vi "ScriptedStateMachine.vi"(8 "ErrorArray In":errorcluster[](array[cluster]), 9 "Data in":variant, 10 "Script":string[](array[string])=["Test,1,2,3", "stop"], 11 "Bus":refnum<class "Bus.lvclass">) -> (0 "ErrorArray Out":errorcluster[](array[cluster]), 2 "Data out":variant, 3 "Bus":refnum<class "Bus.lvclass">)   [LabVIEW 2014, in "Bus_class.lvlib" / "Bus.lvclass"]
uses:
  Bus.lvclass
  Public/TypeDefs/clBusData.ctl
  FrontPanel/TypeDefs/clEventConfig.ctl
  Modules/PmuImpairPlugins/PmuImpairPluginBase_class/TypeDefs/clImpairConfig.ctl
  Modules/EventPlugins/EventPluginBaseClass/TypeDefs/clEvtReportArray.ctl
  Modules/EventPlugins/EventPluginBaseClass/TypeDefs/clEvtReport.ctl
  Modules/EventPlugins/EventPluginBaseClass/TypeDefs/dblEvtSignalArray.ctl
  Modules/NetworkImpairmentModule/PublicAPI/Arguments/Broadcasts/dblNetworkTime.ctl
  Modules/NetworkImpairmentModule/PublicAPI/Arguments/Broadcasts/dblPktLoss.ctl
  Modules/FlagImpairModule/PublicAPI/Arguments/Broadcasts/ui32FlagImpairmentArray.ctl
  Modules/OutputToFilePlugins/OutputToFileBasePlugin/Typedefs/PmuCfgOpt.ctl
  Bus.lvclass/Bus.ctl
  BdcstInfo.ctl
  ModuleType.ctl
  FrontPanel/TypeDefs/clFrontPanelControlRefs.ctl
  Modules/PmuImpairModule/PublicAPI/Arguments/Broadcasts/clErrorRpt.ctl
  Modules/EventPlugins/EventPluginBaseClass/TypeDefs/clEvtConfig.ctl
  Accessors/Read AppModuleID.vi
  Accessors/Read OutputToFileModuleID.vi
  <vilib>/Utility/error.llb/Error Cluster From Error Code.vi
  <vilib>/Analysis/1siggen.llb/Ramp Pattern by Delta.vi
  <vilib>/ErrorRing/Error Ring.xnode
  <userlib>/NIST/NISTErrorLib/NISTErrorLib.lvlib
  Framework.lvlib
  Modules/EventModule/EventModule.lvlib
  Modules/EventPlugins/EventPluginBaseClass/EventPluginBaseClass.lvclass
  <vilib>/Analysis/NI_AALBase.lvlib
  Modules/PmuImpairModule/PmuImpairModule.lvlib
  Modules/NetworkImpairmentModule/NetworkImpairmentModule.lvlib
  Modules/FlagImpairModule/FlagImpairModule.lvlib
  Modules/PmuImpairPlugins/PmuImpairPluginBase_class/PmuImpairPluginBase.lvclass
  Modules/OutputToFilePlugins/OutputToFileBasePlugin/OutputToFileBasePlugin.lvclass
  Modules/OutputToFileModule/OutputToFileModule.lvlib
  Modules/AppModule/AppModule.lvlib
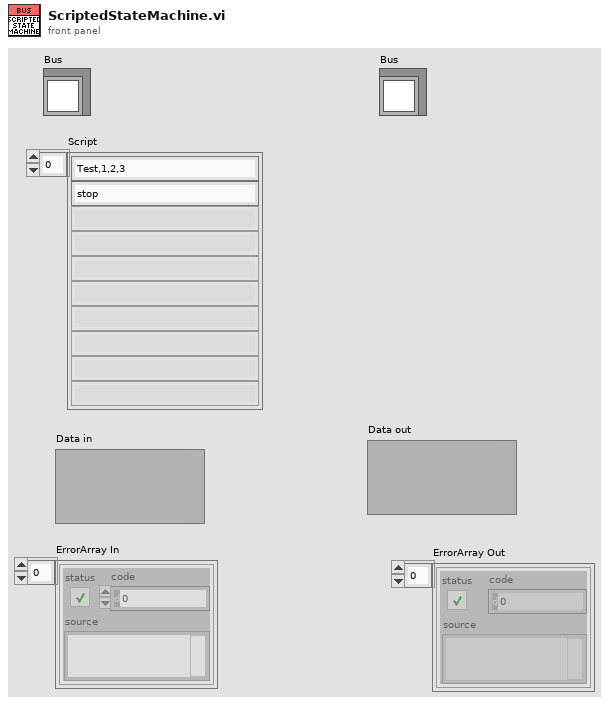
[diagram p1: front panel]
types:
  T1 = typedef "Bus_class.lvlib/Bus.lvclass/clBusData.ctl" = cluster{"BusNumber":u8, "EvtPluginINIFilePath":path, "EvtParams":string[][], "EvtConfig":T2, "Start Time":dbl, "End Time":dbl, "PmuImpairPluginINIFilePath":path, "PmuImpairParams ":string[][], "PmuImpairConfig":T3, "NetImpPluginINIFilePath":path, "NetImpParams":string[][], "FlagImpPluginINIFilePath":path, "FlagImpParams":string[][], "EvtReportArray":T4, "EventSignalArray":T6, "ImpairReportArray":T4, "NetworkTime":T7, "PktLoss":T8, "FlagImpArray":T9, "OutputToFilePluginINIFilePath":path, "Output File Path":path, "clConfigOptions":T10, "AppPluginINIFilePath":path, "AppConfig":variant, "AppOutput":variant}
  T2 = typedef "Framework.lvlib/clEventConfig.ctl" = cluster{"UTC Time 0":timestamp, "Nominal Frequency":u16, "Reporting Rate":u16, "Fsamp":u32, "PosSeq":bool}
  T3 = typedef "PmuImpairPlugins.lvlib/PmuImpairPluginBase.lvclass/clImpairConfig.ctl" = cluster{"FilterType":string, "bPosSeq":bool}
  T4 = typedef "EventPlugins.lvlib/EventPluginBaseClass.lvclass/clEvtReportArray.ctl" = T5[]
  T5 = typedef "EventPlugins.lvlib/EventPluginBaseClass.lvclass/clEvtReport.ctl" = cluster{"Timestamp":dbl, "Synx":cdb[], "Freq":dbl, "ROCOF":dbl, "ID":i16}
  T6 = typedef "EventPlugins.lvlib/EventPluginBaseClass.lvclass/dblEvtSignalArray.ctl" = dbl[][]
  T7 = typedef "NetworkImpairmentModule.lvlib/dblNetworkTime.ctl" = dbl[]
  T8 = typedef "NetworkImpairmentModule.lvlib/dblPktLoss.ctl" = dbl[]
  T9 = typedef "FlagImpairModule.lvlib/ui32FlagImpairmentArray.ctl" = u32[]
  T10 = typedef "OutputToFilePlugins.lvlib/OutputToFileBasePlugin.lvclass/PmuCfgOpt.ctl" = cluster{"TIME_BASE":u64, "STN":string, "IDCODE":u16, "rdoPolRect":enum32{"Rectangular", "Polar"}, "rdoFloatInt":enum32{"Float", "Integer"}, "PHUNIT":u64, "rdoFreqDfreq":enum32{"Float", "Integer"}, "CHNAM":string[], "chkCfg2Prefix":bool}
  T11 = typedef "Bus_class.lvlib/Bus.lvclass/ModuleType.ctl" = enum16{"PMU", "Event", "Network", "Flag", "App", "OutToFile"}
  T12 = typedef "Bus_class.lvlib/Bus.lvclass/BdcstInfo.ctl" = cluster{"ModuleType":T11, "ModuleID":i32, "UsrEvtRef":variant, "ScriptCmd":string}
  T13 = typedef "Framework.lvlib/clFrontPanelControlRefs.ctl" = cluster{"TestFilePathRef":refnum<vi>, "BusNumberRef":refnum<vi>, "NumberOfBusesRef":refnum<vi>, "EvtTypeRef":refnum<vi>, "EvtParamsRef":refnum<vi>, "EvtConfigRef":refnum<vi>, "StartTimeRef":refnum<vi>, "EndTimeRef":refnum<vi>, "PmuImpairTypeRef":refnum<vi>, "PmuImpairParamsRef":refnum<vi>, "NetImpairParamsRef":refnum<vi>, "FlagImpairTypeRef":refnum<vi>, "FlagImpairParamsRef":refnum<vi>, "NetImpairTypeRef":refnum<vi>, "OutputFileType":refnum<vi>, "PmuImpairConfigRef":refnum<vi>, "AppTypeRef":refnum<vi>, "ScriptPathRef":refnum<vi>, "ShowPanels?":refnum<vi>}
  T14 = typedef "PmuImpairModule.lvlib/clErrorRpt.ctl" = cluster{"error":errorcluster, "AdditionalInfo":string}
  T15 = typedef "EventPlugins.lvlib/EventPluginBaseClass.lvclass/clEvtConfig.ctl" = cluster{"T0(UTC)":dbl, "F0":dbl, "Fs":i32, "FSamp":u32, "bPosSeq":bool}
  T16 = typedef "EventModule.lvlib/clBroadcastEvents.ctl" = cluster{"DidInit":refnum<user-event>, "StatusUpdate":refnum<user-event>, "ErrorReport":refnum<user-event>, "DidStop":refnum<user-event>, "ReadEvtConfig":refnum<user-event>, "ReadTimeArray":refnum<user-event>, "ReadEvtParams":refnum<user-event>, "GetEvtReportArray":refnum<user-event>, "ReadPathToPlugin":refnum<user-event>, "GetEvtSignal":refnum<user-event>, "ReadBusNumber":refnum<user-event>}
  T17 = typedef "PmuImpairModule.lvlib/clBroadcastEvents.ctl" = cluster{"DidInit":refnum<user-event>, "StatusUpdate":refnum<user-event>, "ErrorReport":refnum<user-event>, "DidStop":refnum<user-event>, "ImpairConfig":refnum<user-event>, "ImpairParams":refnum<user-event>, "ImpairReports":refnum<user-event>, "PathToPlugin":refnum<user-event>, "BusNumber":refnum<user-event>}
  T18 = typedef "NetworkImpairmentModule.lvlib/clBroadcastEvents.ctl" = cluster{"DidInit":refnum<user-event>, "StatusUpdate":refnum<user-event>, "ErrorReport":refnum<user-event>, "DidStop":refnum<user-event>, "ReadNetImpParams":refnum<user-event>, "ReadLossThreshold":refnum<user-event>, "GetNetworkTime":refnum<user-event>, "GetPktLoss":refnum<user-event>, "ReadPathToPlugin":refnum<user-event>}
  T19 = typedef "FlagImpairModule.lvlib/clBroadcastEvents.ctl" = cluster{"DidInit":refnum<user-event>, "StatusUpdate":refnum<user-event>, "ErrorReport":refnum<user-event>, "DidStop":refnum<user-event>, "ReadFlagImpairConfig":refnum<user-event>, "ReadPluginINIFilePath":refnum<user-event>, "ReadFlagImpairParams":refnum<user-event>, "ReadTimeArray":refnum<user-event>, "GetFlagImpairment":refnum<user-event>}
  T20 = typedef "OutputToFileModule.lvlib/clBroadcastEvents.ctl" = cluster{"DidInit":refnum<user-event>, "StatusUpdate":refnum<user-event>, "ErrorReport":refnum<user-event>, "DidStop":refnum<user-event>, "PathToPlugin":refnum<user-event>, "PmuConfig":refnum<user-event>, "OutputPath":refnum<user-event>}
  T21 = typedef "AppModule.lvlib/clBroadcastEvents.ctl" = cluster{"DidInit":refnum<user-event>, "StatusUpdate":refnum<user-event>, "ErrorReport":refnum<user-event>, "DidStop":refnum<user-event>, "PathToINI":refnum<user-event>, "InputData":refnum<user-event>, "OutputData":refnum<user-event>, "BcAppInfo":refnum<user-event>, "ConfigData":refnum<user-event>}
  T22 = typedef "Framework.lvlib/clFrameworkData.ctl" = cluster{"EvtINIFilePaths":path[], "BusClassInstances":refnum<class "Bus.lvclass">[], "PmuImpairINIFilePaths":path[], "FlagImpairINIFilePaths":path[], "NetImpairINIFilePaths":path[], "OutputToFileINIFilePaths":path[], "AppINIFilePaths":path[], "AppModuleID":i32, "OutputToFileID":i32}
  T23 = typedef "Framework.lvlib/QueRef.ctl" = refnum<queue>
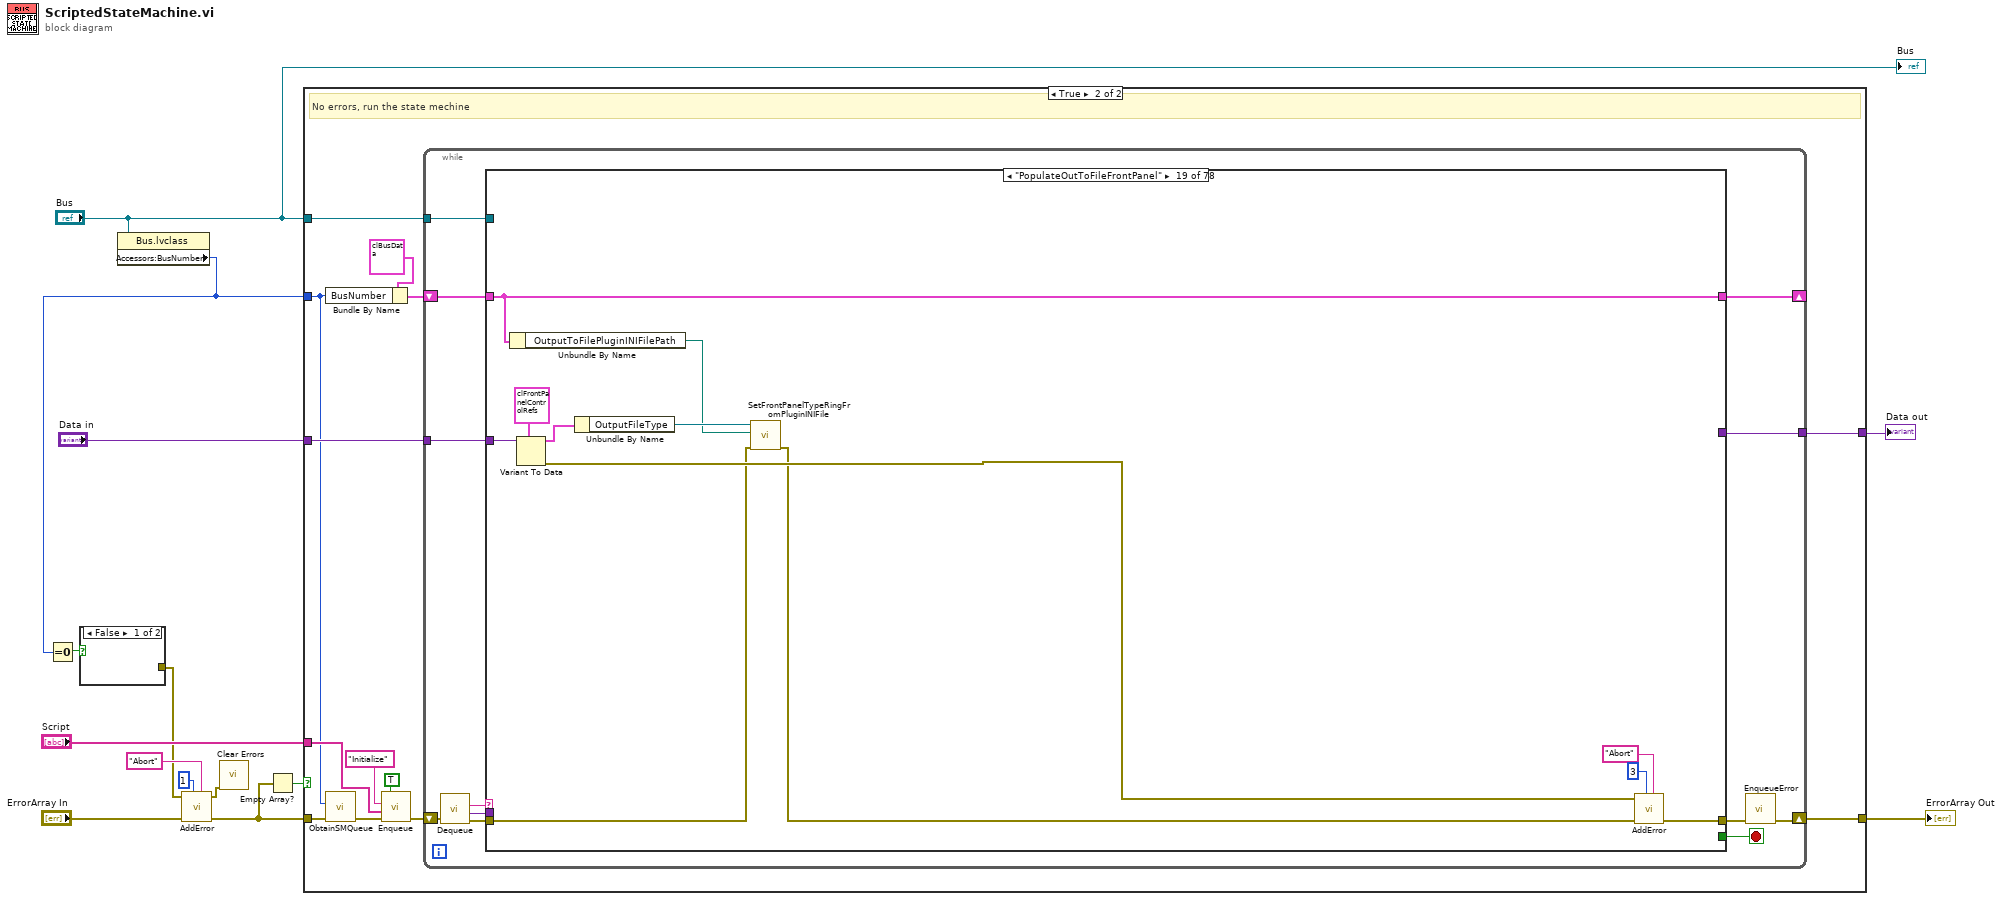
[diagram p0: block diagram]
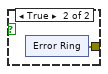
[diagram p2: hidden frame]
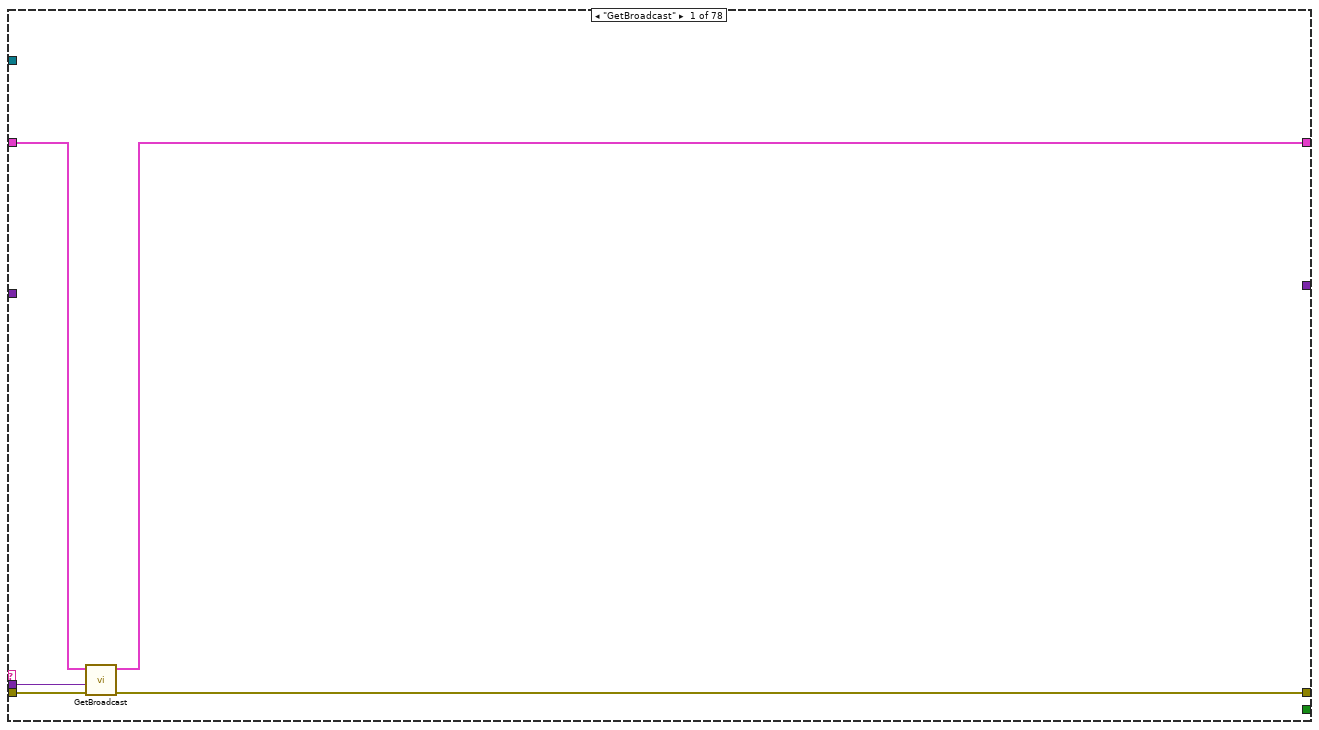
[diagram p4: hidden frame]
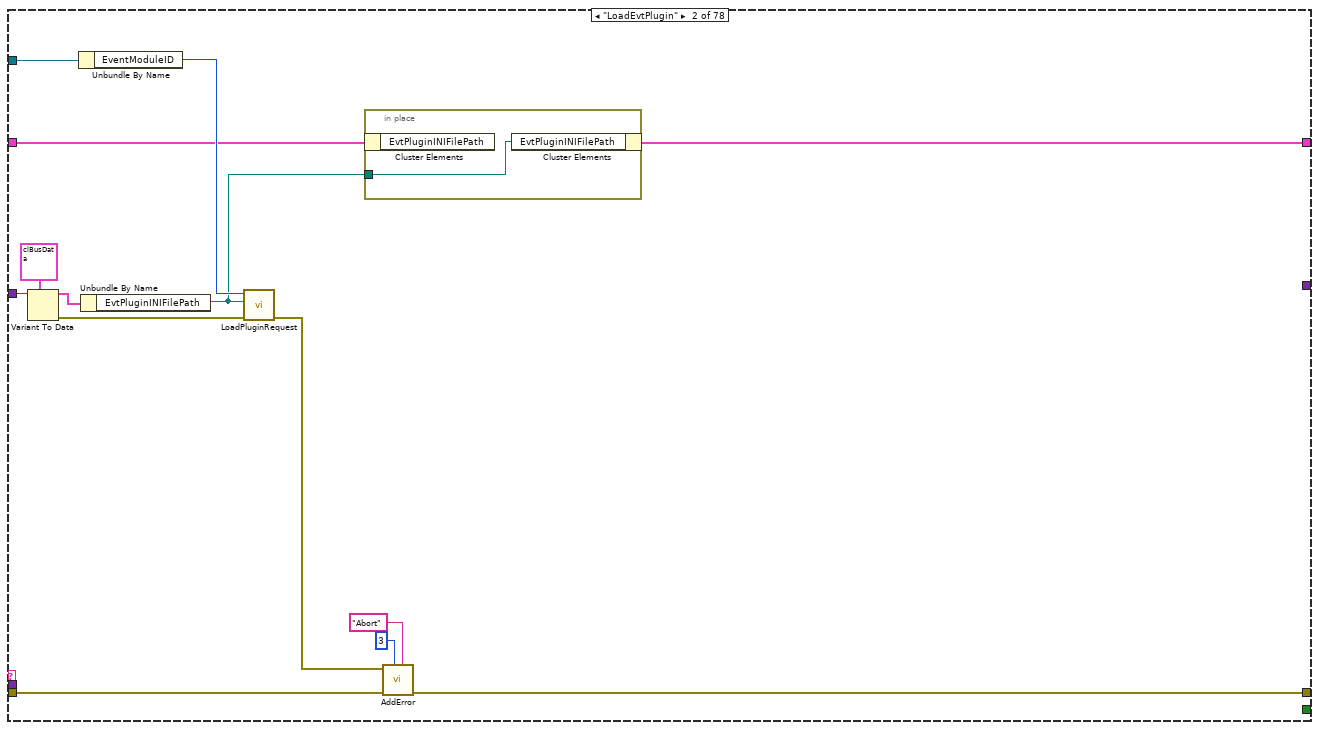
[diagram p5: hidden frame]
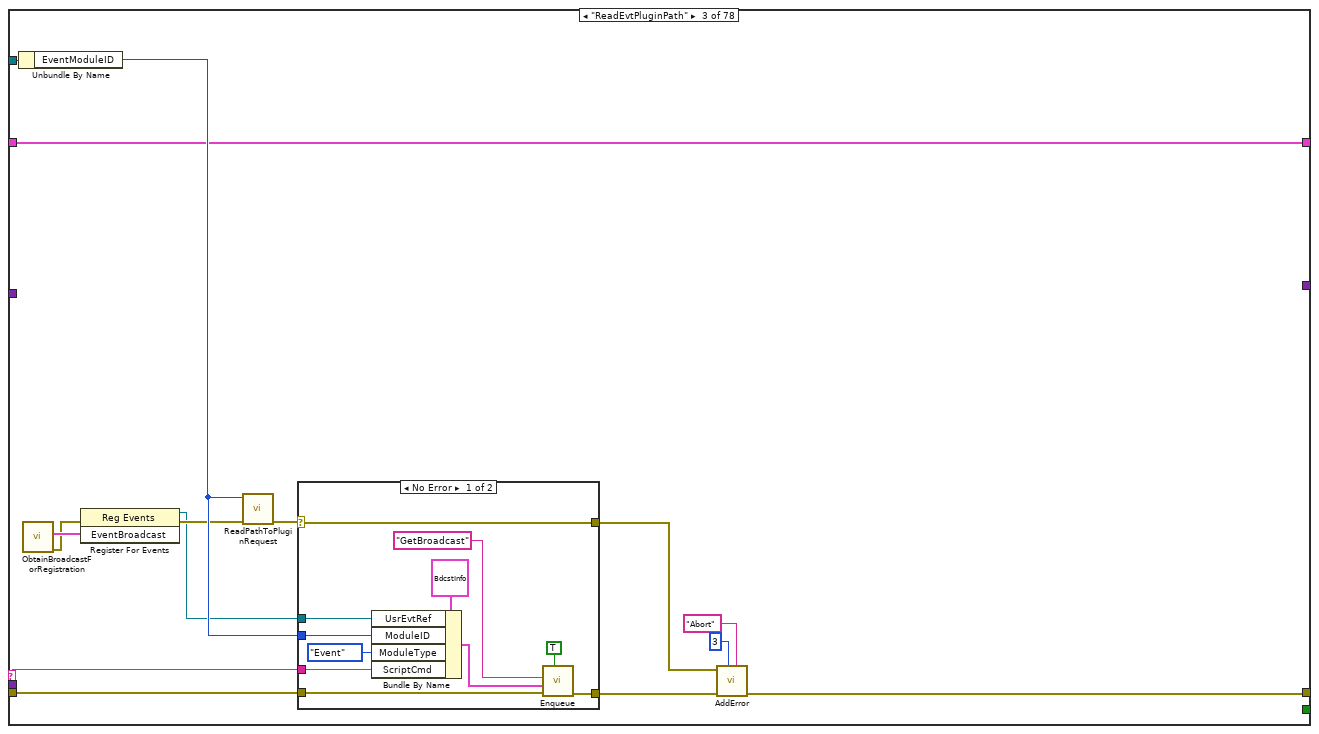
[diagram p6: hidden frame]
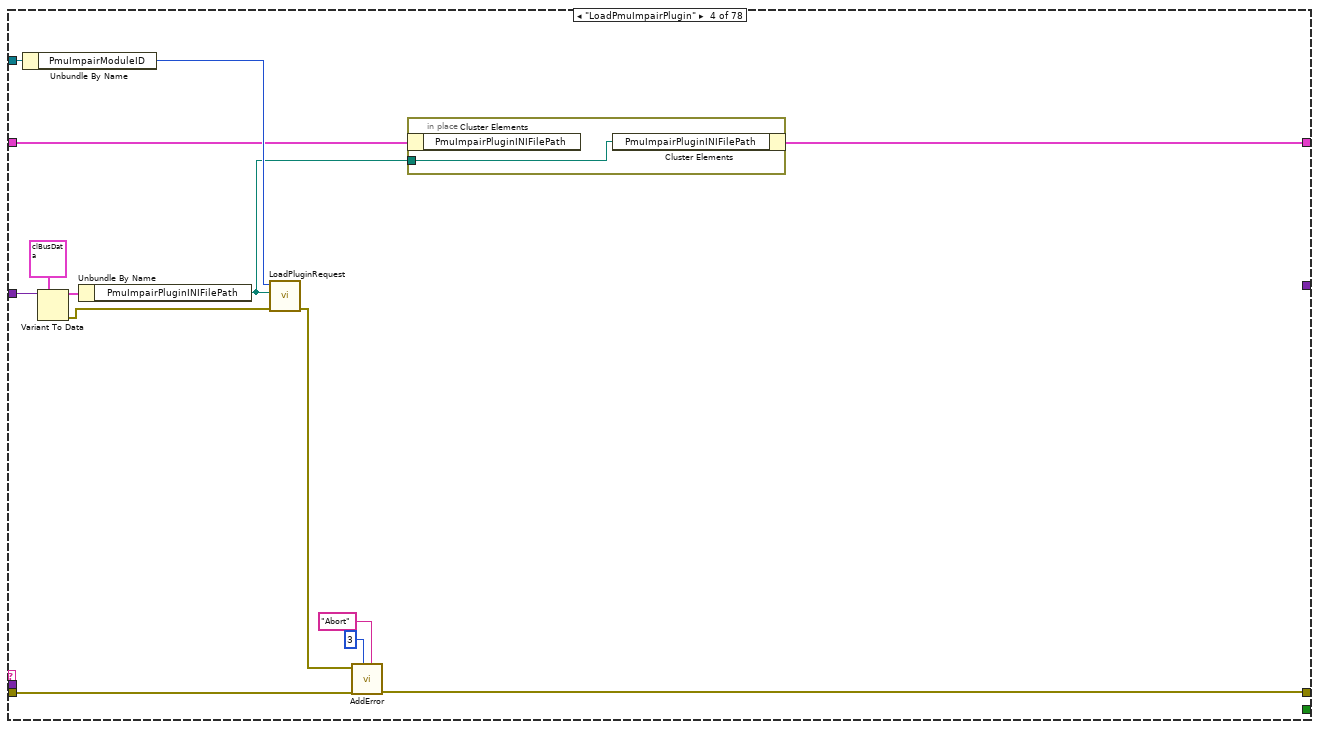
[diagram p8: hidden frame]
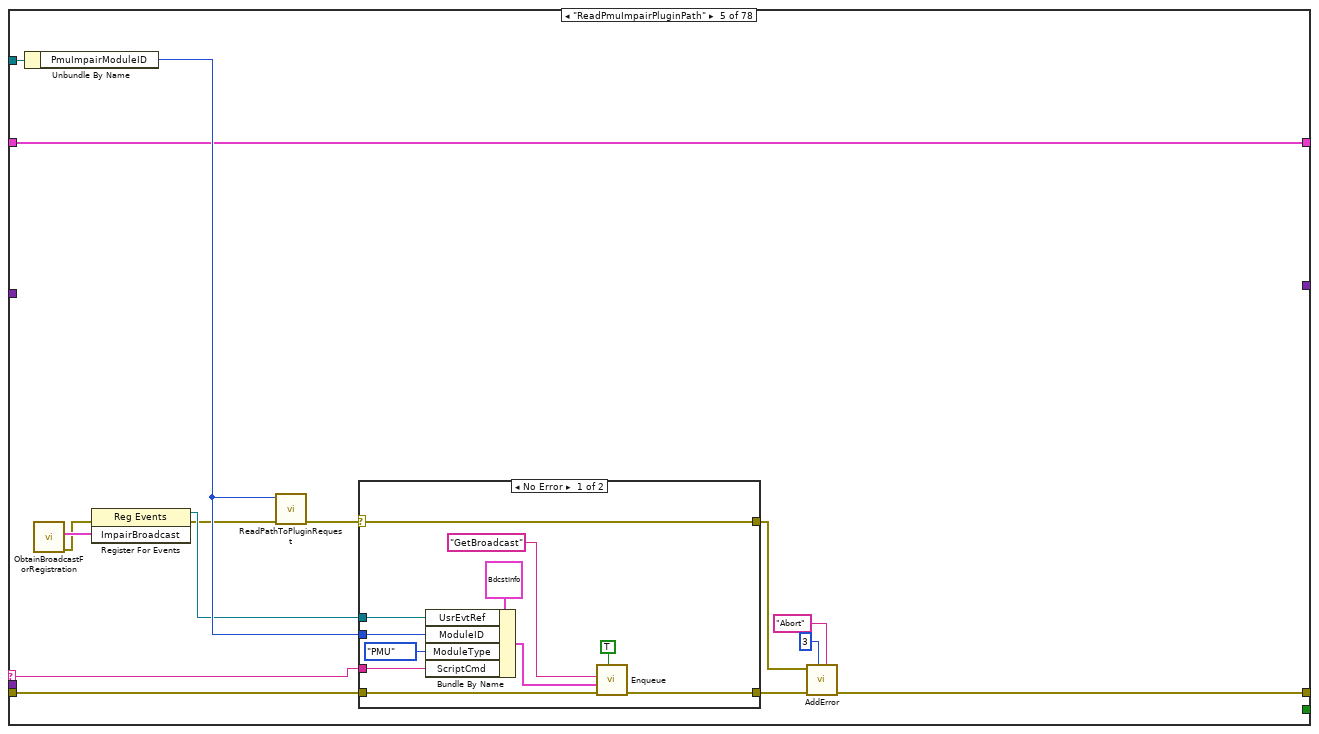
[diagram p9: hidden frame]
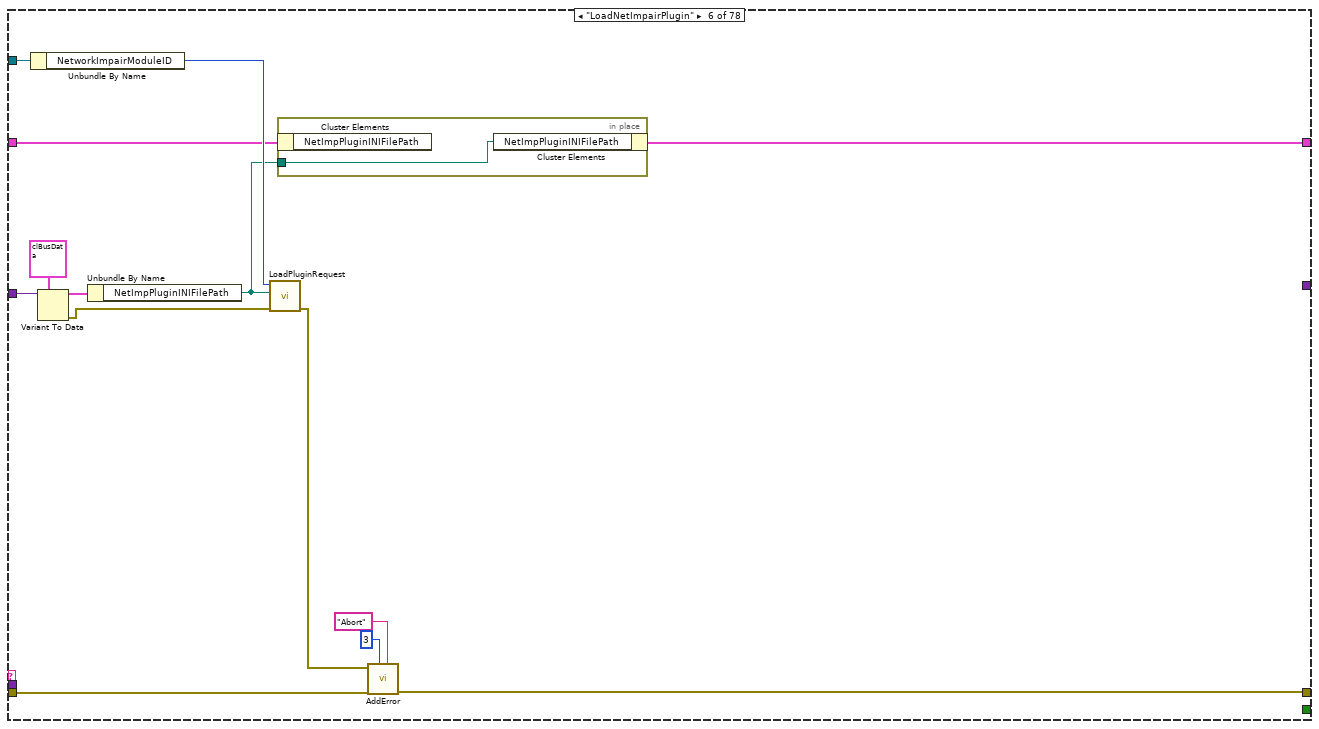
[diagram p11: hidden frame]
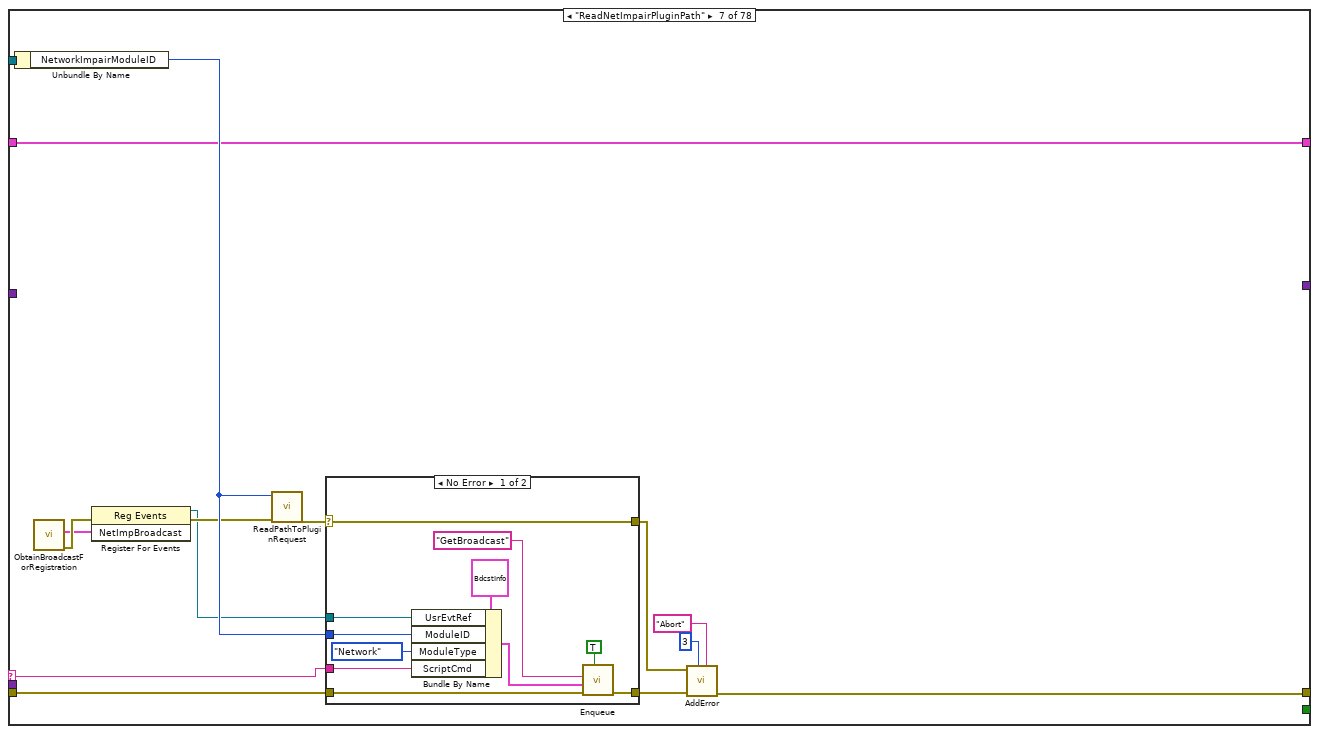
[diagram p12: hidden frame]
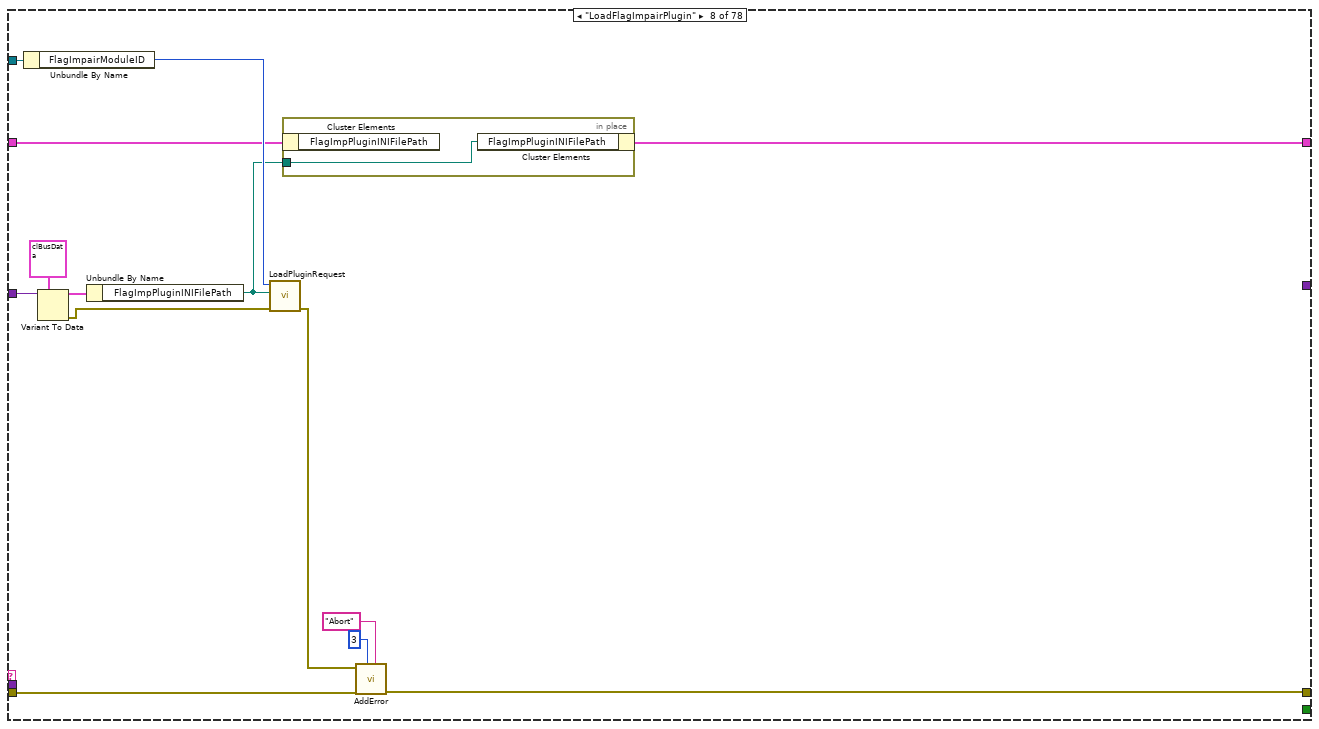
[diagram p14: hidden frame]
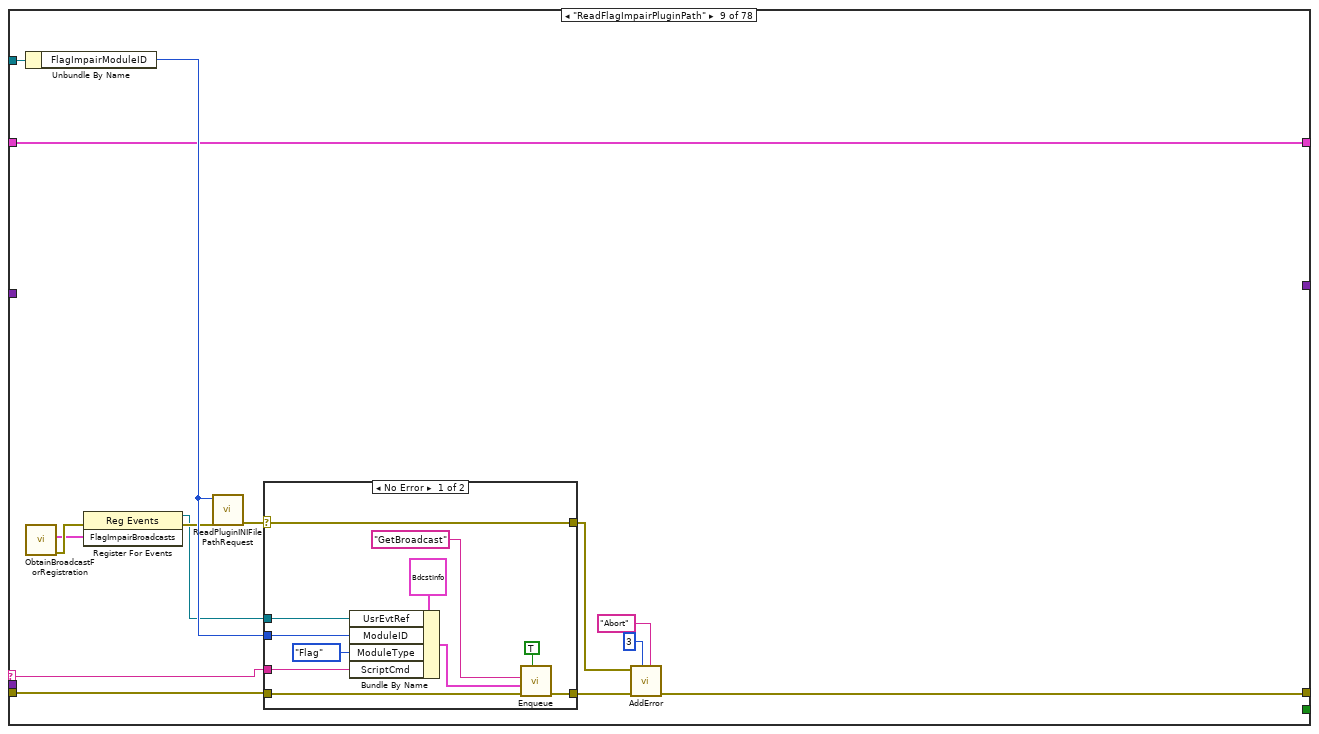
[diagram p15: hidden frame]
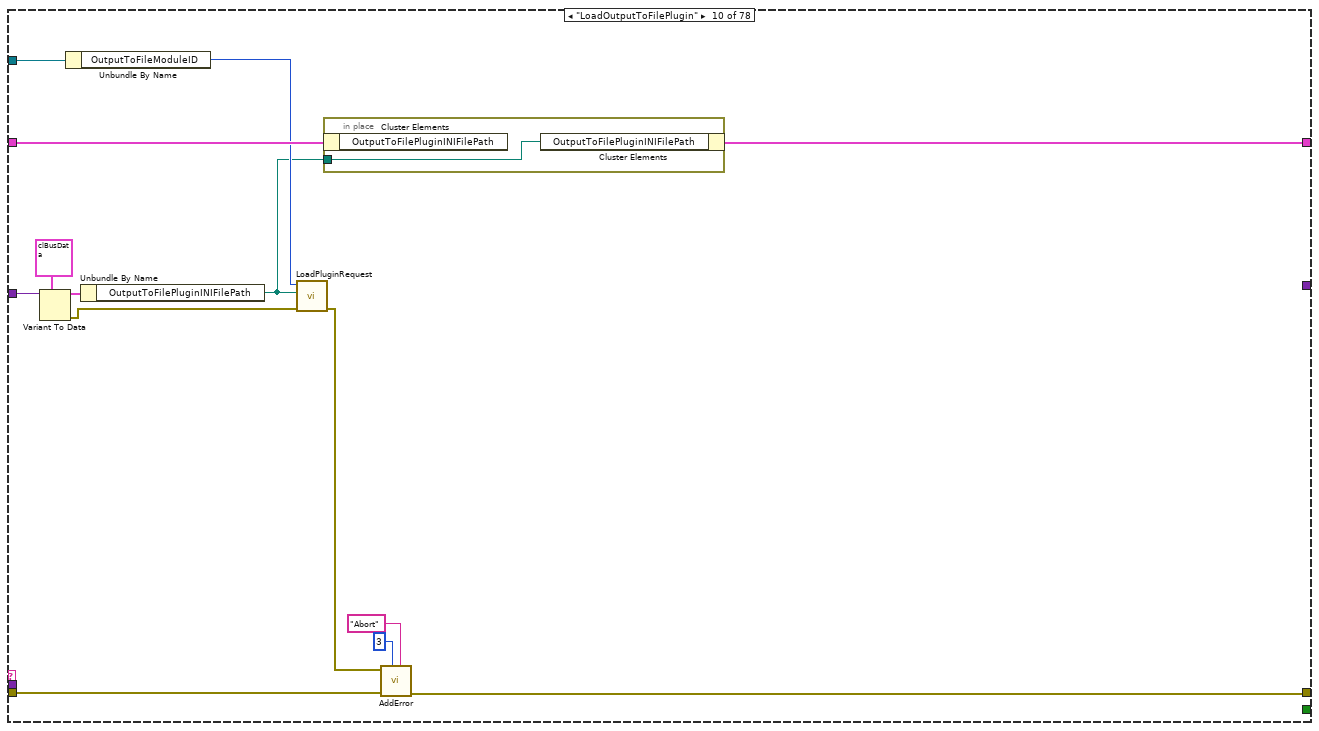
[diagram p17: hidden frame]
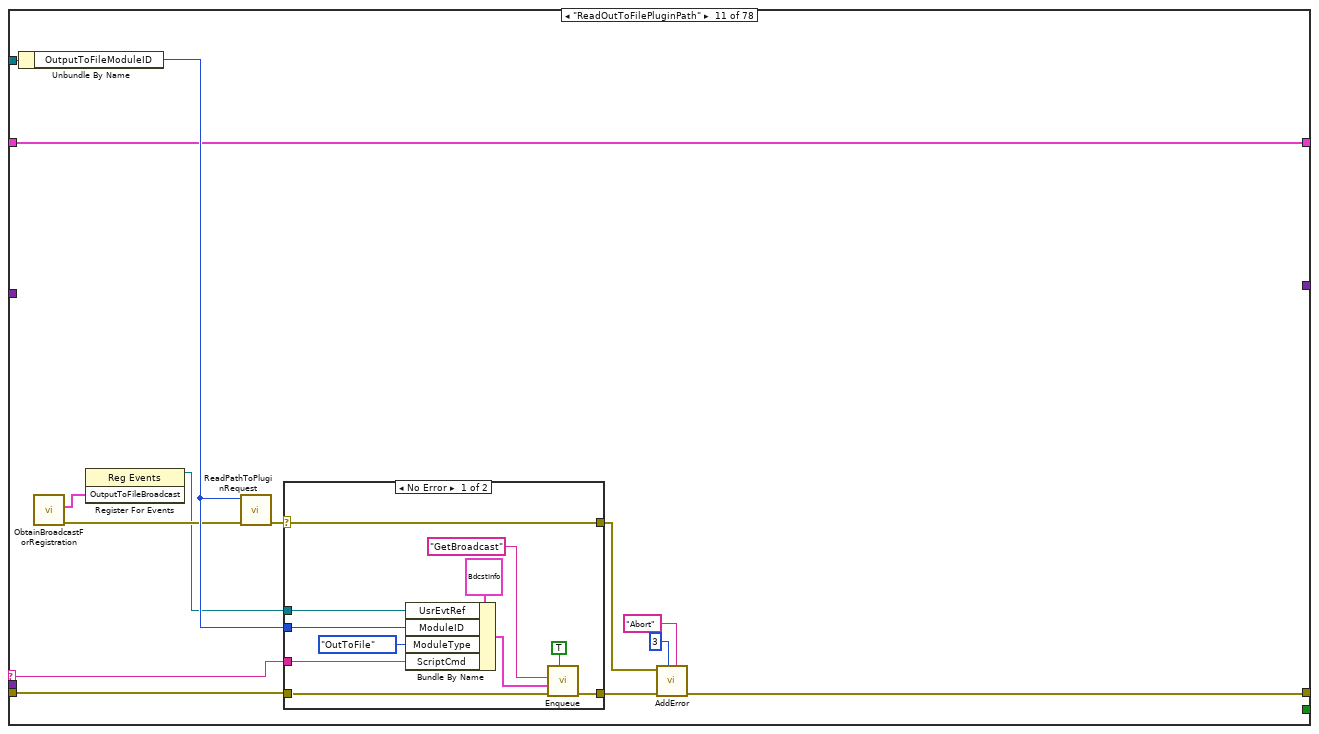
[diagram p18: hidden frame]
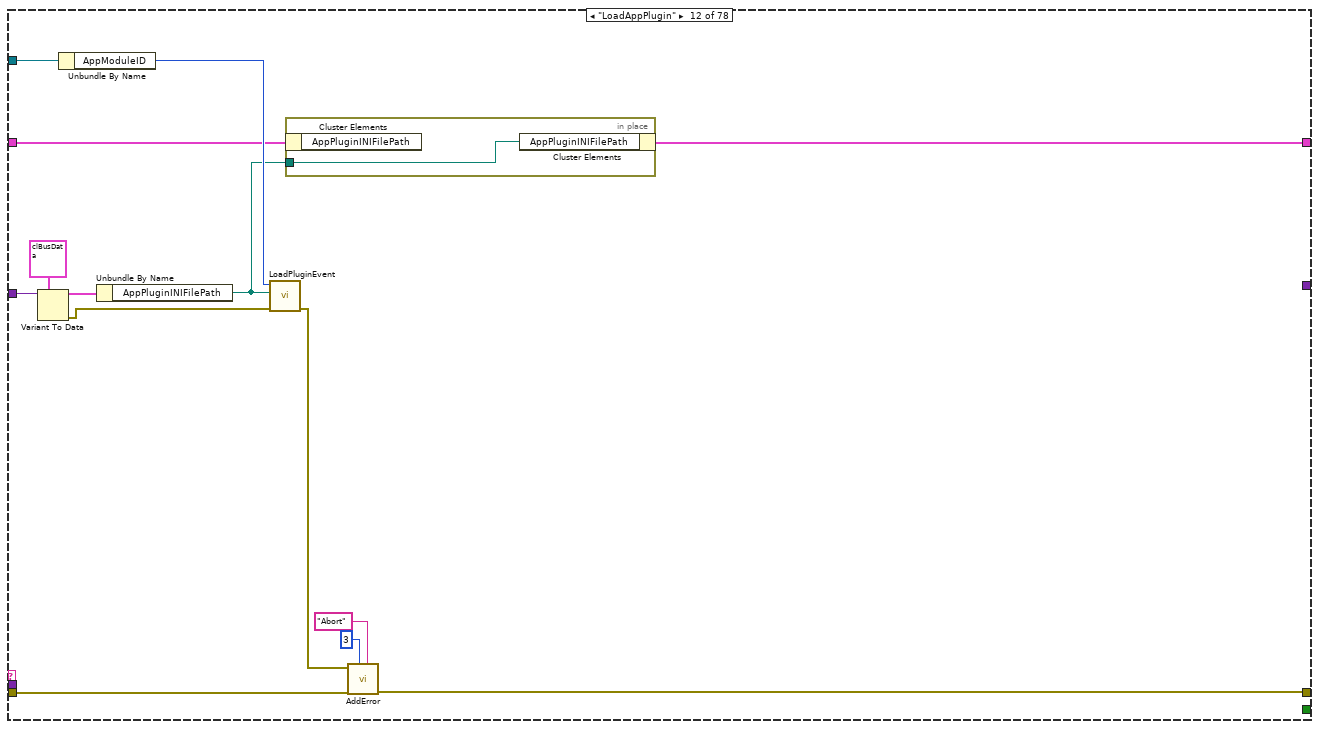
[diagram p20: hidden frame]
diagram:
  n1 = property class="Bus.lvclass"(reference="Bus") -> ("Accessors:BusNumber"=w2:u8)  [unwired: 1 in, 2 out]
  n2 = Equal To 0?(x=w2) -> (x = 0?=w5:bool)
  n3 = case shown="False" w5 {
    tunnel: [_ w15] -> w4
    frame False {
    }
    frame True {
      n4 = xnode "Error Ring"() -> ("error out"=w15:errorcluster)
    }
  }
  n5 = call <userlib>:"AddError.vi"("Severity"="Abort" ("String"), "Priority"=u8 1, "ErrorArray"="ErrorArray In", "error in (no error)"=w4) -> ("ErrorArray"=w8:errorcluster[], "error out"=w3:errorcluster)  [unwired: 6 in]
  n6 = call <vilib>:"Clear Errors.vi"("error in (no error)"=w3) -> ()  [unwired: 5 in, 2 out]
  n7 = Empty Array?(array=w8) -> (empty?=w14:bool)
  n8 = case shown="True" w14 {
    tunnel: w8 -> [w17 w30]
    tunnel: [w17 w25] -> w13
    tunnel: "Bus" -> [_ w24]
    tunnel: "Script" -> [_ w23]
    tunnel: "Data in" -> [_ w22]
    tunnel: [_ w21] -> w10
    tunnel: w2 -> [_ w18]
    frame False {
      # "Errors coming into the state machine, don't run it."
    }
    frame True {
      # "No errors, run the state mechine"
      n9 = Bundle By Name(cluster=T1 {"BusNumber"=0, "EvtPluginINIFilePath"=path "", "EvtParams"=[], "EvtConfig"={"UTC Time 0"=timestamp(0 s since 1904-01-01), "Nominal Frequency"=60, "Reporting Rate"=60, "Fsamp"=960, "PosSeq"=FALSE}, "Start Time"=0.0, "End Time"=0.0, "PmuImpairPluginINIFilePath"=path "", "PmuImpairParams "=[["960"], ["8.19"], ["164"]], "PmuImpairConfig"={"FilterType"="", "bPosSeq"=TRUE}, "NetImpPluginINIFilePath"=path "", "NetImpParams"=[], "FlagImpPluginINIFilePath"=path "", "FlagImpParams"=[], "EvtReportArray"=[], "EventSignalArray"=[], "ImpairReportArray"=[], "NetworkTime"=[], "PktLoss"=[], "FlagImpArray"=[], "OutputToFilePluginINIFilePath"=path "", "Output File Path"=path "", "clConfigOptions"={"TIME_BASE"=1000000, "STN"="Bus_1", "IDCODE"=0, "rdoPolRect"=enum."Rectangular", "rdoFloatInt"=enum."Float", "PHUNIT"=1000000, "rdoFreqDfreq"=enum."Float", "CHNAM"=["VA", "VB", "VC", "V+", "IA", "IB", "IC", "I+"], "chkCfg2Prefix"=TRUE}, "AppPluginINIFilePath"=path "", "AppConfig"=variant, "AppOutput"=variant} ("clBusData"), "BusNumber"=w18) -> (w19:T1)
      n10 = call "ObtainSMQueue.vi"("ErrorArray"=w30, "BusNumber"=w18) -> ("ErrorArray"=w29:errorcluster[])  [unwired: 8 in, 1 out]
      n11 = call "Enqueue.vi"("Priority (f)"=TRUE, "ErrorArray"=w29, "Data"=w23, "Msg"="Initialize") -> ("ErrorArray"=w26:errorcluster[])  [unwired: 7 in]
      n12 = while {
        shift-right: [w37] -> w25
        shift-left: w26 -> [w42]
        tunnel: w24 -> [w35]
        tunnel: w22 -> [w34]
        tunnel: [w33] -> w21
        shift-right: [w32] -> _
        shift-left: w19 -> [w31]
        stop <- w38 stop-if-true
        n13 = call "Dequeue.vi"("ErrorArray"=w42) -> ("ErrorArray"=w40:errorcluster[], "Data"=w39:variant, "Msg"=w41:string)  [unwired: 8 in]
        n14 = case shown="\"PopulateOutToFileFrontPanel\"" w41 {
          selector: w41 -> [_ _ w70 _ w114 _ w156 _ w199 _ w241 _ w283 _ _ _ _ _ _ _ w480 _ w524 w556 _ w602 w629 _ w671 _ w708 _ w754 _ w808 _ w879 w909 _ _ _ w994 _ w1044 _ w1089 _ _ w1145 _ _ _ _ _ _ _ _ _ _ _ _ w1355 _ _ w1416 _ _ _ _ _ w1539 _ w1590 w1619 _ w1662 w1710 w1747]
          tunnel: w40 -> [w44 w53 w69 w96 w112 w139 w155 w182 w198 w221 w240 w267 w282 w331 w339 w369 w385 w404 w416 w429 w478 w520 w529 w555 w586 w601 w628 w652 w670 w701 w715 w742 w761 w796 w815 w842 w886 w914 w953 w969 w980 w1001 w1029 w1042 w1069 w1087 w1115 w1129 w1143 w1223 w1233 w1243 w1253 w1263 w1274 w1284 w1294 w1310 w1319 w1329 w1343 w1363 w1385 w1404 w1424 w1446 w1463 w1481 w1517 w1532 w1538 _ w1595 w1624 w1648 w1668 w1707 w1753]
          tunnel: w39 -> [w43 _ _ _ _ _ _ _ _ _ _ _ _ _ _ _ _ _ _ _ _ _ _ _ _ _ _ _ _ _ _ _ _ _ _ _ _ _ _ _ _ _ _ _ _ _ _ _ _ _ _ _ _ _ _ _ _ _ _ _ _ _ _ _ _ _ _ w1479 _ _ _ w1558 _ _ _ _ _ _]
          tunnel: [w45 w55 w73 w97 w116 w140 w159 w183 w202 w223 w244 w268 w286 w305 w343 w376 w386 w407 w419 w429 w474 w515 w531 w559 w588 w605 w632 w654 w674 w703 w717 w744 w763 w798 w817 w843 w890 w916 w936 w970 w982 w1003 w1031 w1045 w1071 w1090 w1117 w1137 w1146 w1229 w1235 w1245 w1255 w1265 w1276 w1286 w1296 w1312 w1321 w1331 w1345 w1365 w1386 w1406 w1426 w1448 w1466 w1482 w1520 w1524 w1537 w1552 w1599 w1628 w1649 w1672 w1692 w1757] -> w36
          tunnel: [_ _ _ _ _ _ _ _ _ _ _ _ _ _ _ _ _ _ _ _ _ _ _ _ _ _ _ _ _ _ _ _ _ _ _ _ _ _ _ _ _ _ _ _ _ _ _ _ _ _ _ _ _ _ _ _ _ _ _ _ _ _ _ _ _ _ _ _ _ TRUE _ _ _ _ _ _ _ _] -> w38
          tunnel: w35 -> [_ w59 w77 w104 w120 w147 w163 w190 w206 w233 w248 w275 w290 _ _ _ _ _ _ _ w486 w522 w536 w563 w585 w609 w636 w659 w678 w700 w721 w741 w767 w805 w822 w853 w893 w921 _ w979 _ w1006 w1028 w1050 w1079 w1095 w1124 w1136 w1153 w1228 w1241 w1251 w1261 w1271 w1281 w1291 w1301 w1317 w1326 w1336 w1353 w1369 w1396 w1414 w1430 w1454 w1469 _ _ _ _ w1551 w1604 w1633 w1659 w1677 _ w1762]
          tunnel: w34 -> [_ w61 _ w102 _ w145 _ w188 _ w231 _ w273 _ w337 w361 w382 w402 w414 w426 _ _ _ _ _ w593 _ _ w663 _ w698 _ w750 _ w803 _ w852 _ _ _ _ _ _ w1024 _ w1077 _ w1122 w1134 _ w1226 _ _ _ _ _ _ _ _ _ _ w1351 _ _ w1412 _ w1459 _ _ _ _ _ _ _ _ _ _ _ _]
          tunnel: [_ _ _ _ _ _ _ _ _ _ _ _ _ _ _ _ _ _ _ _ _ _ _ _ _ _ _ _ _ _ _ _ _ _ _ _ _ _ _ _ _ _ _ _ _ _ _ _ _ _ _ _ _ _ _ _ _ _ _ _ _ _ _ _ _ _ _ _ _ w1522 variant ("Data in") _ _ _ _ _ _ _] -> w33
          tunnel: [w46 w48 w71 w91 w115 w134 w157 w178 w200 w226 w242 w262 w284 w304 w341 w374 w384 w406 w418 w427 w479 w516 w530 w557 w582 w603 w630 w651 w672 w692 w716 w736 w762 w783 w816 w839 w888 w915 w935 w956 w986 w1002 w1021 w1048 w1064 w1093 w1111 w1126 w1150 w1211 w1242 w1252 w1262 w1272 w1282 w1292 w1302 w1318 w1327 w1337 w1339 w1364 w1395 w1400 w1425 w1445 w1468 w1470 w1516 w1521 w1534 w1550 w1596 w1627 w1658 w1671 w1704 w1756] -> w32
          tunnel: w31 -> [w47 w49 w71 w92 w115 w136 w157 w179 w200 w232 w242 w264 w284 w304 w341 w374 w384 w406 w418 w428 w479 w516 w530 w557 w583 w603 w630 w661 w672 w694 w716 w737 w762 w784 w816 w840 w888 w915 w935 w956 w986 w1002 w1023 w1048 w1065 w1093 w1112 w1128 w1151 w1211 w1242 w1252 w1262 w1272 w1282 w1292 w1302 w1318 w1327 w1337 w1340 w1364 w1395 w1401 w1425 w1457 w1468 w1470 w1516 w1521 w1534 w1550 w1596 w1627 w1658 w1671 w1705 w1756]
          frame "GetBroadcast" {
            n15 = call "GetBroadcast.vi"("Error In"=w44, "BdcstInfo"=w43, "clBusData In"=w47) -> ("Error Out"=w45:errorcluster[], "clBusData Out"=w46:T1)  [unwired: 7 in]
          }
          frame "LoadEvtPlugin" {
            n16 = Variant To Data(type=T1 {"BusNumber"=0, "EvtPluginINIFilePath"=path "", "EvtParams"=[], "EvtConfig"={"UTC Time 0"=timestamp(0 s since 1904-01-01), "Nominal Frequency"=60, "Reporting Rate"=60, "Fsamp"=960, "PosSeq"=FALSE}, "Start Time"=0.0, "End Time"=0.0, "PmuImpairPluginINIFilePath"=path "", "PmuImpairParams "=[["960"], ["8.19"], ["164"]], "PmuImpairConfig"={"FilterType"="", "bPosSeq"=TRUE}, "NetImpPluginINIFilePath"=path "", "NetImpParams"=[], "FlagImpPluginINIFilePath"=path "", "FlagImpParams"=[], "EvtReportArray"=[], "EventSignalArray"=[], "ImpairReportArray"=[], "NetworkTime"=[], "PktLoss"=[], "FlagImpArray"=[], "OutputToFilePluginINIFilePath"=path "", "Output File Path"=path "", "clConfigOptions"={"TIME_BASE"=1000000, "STN"="Bus_1", "IDCODE"=0, "rdoPolRect"=enum."Rectangular", "rdoFloatInt"=enum."Float", "PHUNIT"=1000000, "rdoFreqDfreq"=enum."Float", "CHNAM"=["VA", "VB", "VC", "V+", "IA", "IB", "IC", "I+"], "chkCfg2Prefix"=TRUE}, "AppPluginINIFilePath"=path "", "AppConfig"=variant, "AppOutput"=variant} ("clBusData"), Variant=w61) -> (data=w51:T1, error out=w52:errorcluster)  [unwired: 1 in]
            n17 = Unbundle By Name(w59) -> ("EventModuleID"=w58:i32)
            n18 = Unbundle By Name(w51) -> ("EvtPluginINIFilePath"=w50:path)
            n19 = call "LoadPluginRequest.vi"("error in (no error)"=w52, "PathToPlugin"=w50, "ModuleID"=w58) -> ("error out"=w54:errorcluster)  [unwired: 8 in]
            n20 = in-place {
              in-place-border: w50 -> [w62]
              n21 = in-place-cluster #1(w49) -> ()  [unwired: 1 out]
              n22 = in-place-cluster #1("EvtPluginINIFilePath"=w62) -> (w48:T1)
            }
            n23 = call <userlib>:"AddError.vi"("Severity"="Abort" ("String"), "Priority"=u8 3, "ErrorArray"=w53, "error in (no error)"=w54) -> ("ErrorArray"=w55:errorcluster[])  [unwired: 6 in, 1 out]
          }
          frame "ReadEvtPluginPath" {
            n24 = Unbundle By Name(w77) -> ("EventModuleID"=w76:i32)
            n25 = call "ObtainBroadcastForRegistration.vi"() -> ("error out"=w65:errorcluster, "EventBroadcast"=w66:T16)  [unwired: 10 in]
            n26 = register-events(error in=w65, w66) -> (reference out=w63:refnum<event-registration>, error out=w64:errorcluster)  [unwired: 1 in]
            n27 = call "ReadPathToPluginRequest.vi"("error in (no error)"=w64, "ModuleID"=w76) -> ("error out"=w67:errorcluster)  [unwired: 9 in]
            n28 = case shown="No Error" w67 {
              selector: w67 -> [w80 w89]
              tunnel: w69 -> [w88 w90]
              tunnel: w76 -> [w85 _]
              tunnel: [w83 w90] -> w68
              tunnel: [w80 w89] -> w72
              tunnel: w70 -> [w79 _]
              tunnel: w63 -> [w78 _]
              frame No Error {
                n29 = Bundle By Name(cluster=T12 {"ModuleType"=enum."PMU", "ModuleID"=0, "UsrEvtRef"=variant, "ScriptCmd"=""} ("GetBdcstData"), "UsrEvtRef"=w78, "ModuleID"=w85, "ModuleType"=ModuleType."Event", "ScriptCmd"=w79) -> (w84:T12)
                n30 = call "Enqueue.vi"("Priority (f)"=TRUE, "ErrorArray"=w88, "Data"=w84, "Msg"="GetBroadcast") -> ("ErrorArray"=w83:errorcluster[])  [unwired: 7 in]
              }
              frame Error {
              }
            }
            n31 = call <userlib>:"AddError.vi"("Severity"="Abort" ("String"), "Priority"=u8 3, "ErrorArray"=w68, "error in (no error)"=w72) -> ("ErrorArray"=w73:errorcluster[])  [unwired: 6 in, 1 out]
          }
          frame "LoadPmuImpairPlugin" {
            n32 = Unbundle By Name(w104) -> ("PmuImpairModuleID"=w100:i32)
            n33 = Variant To Data(type=T1 {"BusNumber"=0, "EvtPluginINIFilePath"=path "", "EvtParams"=[], "EvtConfig"={"UTC Time 0"=timestamp(0 s since 1904-01-01), "Nominal Frequency"=60, "Reporting Rate"=60, "Fsamp"=960, "PosSeq"=FALSE}, "Start Time"=0.0, "End Time"=0.0, "PmuImpairPluginINIFilePath"=path "", "PmuImpairParams "=[["960"], ["8.19"], ["164"]], "PmuImpairConfig"={"FilterType"="", "bPosSeq"=TRUE}, "NetImpPluginINIFilePath"=path "", "NetImpParams"=[], "FlagImpPluginINIFilePath"=path "", "FlagImpParams"=[], "EvtReportArray"=[], "EventSignalArray"=[], "ImpairReportArray"=[], "NetworkTime"=[], "PktLoss"=[], "FlagImpArray"=[], "OutputToFilePluginINIFilePath"=path "", "Output File Path"=path "", "clConfigOptions"={"TIME_BASE"=1000000, "STN"="Bus_1", "IDCODE"=0, "rdoPolRect"=enum."Rectangular", "rdoFloatInt"=enum."Float", "PHUNIT"=1000000, "rdoFreqDfreq"=enum."Float", "CHNAM"=["VA", "VB", "VC", "V+", "IA", "IB", "IC", "I+"], "chkCfg2Prefix"=TRUE}, "AppPluginINIFilePath"=path "", "AppConfig"=variant, "AppOutput"=variant} ("clBusData"), Variant=w102) -> (data=w101:T1, error out=w95:errorcluster)  [unwired: 1 in]
            n34 = Unbundle By Name(w101) -> ("PmuImpairPluginINIFilePath"=w93:path)
            n35 = call "LoadPluginRequest.vi"("error in (no error)"=w95, "PathToPlugin"=w93, "ModuleID"=w100) -> ("error out"=w94:errorcluster)  [unwired: 8 in]
            n36 = call <userlib>:"AddError.vi"("Severity"="Abort" ("String"), "Priority"=u8 3, "ErrorArray"=w96, "error in (no error)"=w94) -> ("ErrorArray"=w97:errorcluster[])  [unwired: 6 in, 1 out]
            n37 = in-place {
              in-place-border: w93 -> [w105]
              n38 = in-place-cluster #2(w92) -> ()  [unwired: 1 out]
              n39 = in-place-cluster #2("PmuImpairPluginINIFilePath"=w105) -> (w91:T1)
            }
          }
          frame "ReadPmuImpairPluginPath" {
            n40 = Unbundle By Name(w120) -> ("PmuImpairModuleID"=w119:i32)
            n41 = call "ObtainBroadcastForRegistration.vi"() -> ("error out"=w108:errorcluster, "ImpairBroadcast"=w109:T17)  [unwired: 10 in]
            n42 = register-events(error in=w108, w109) -> (reference out=w107:refnum<event-registration>, error out=w106:errorcluster)  [unwired: 1 in]
            n43 = call "ReadPathToPluginRequest.vi"("error in (no error)"=w106, "ModuleID"=w119) -> ("error out"=w110:errorcluster)  [unwired: 9 in]
            n44 = case shown="No Error" w110 {
              selector: w110 -> [w125 w133]
              tunnel: [w128 w132] -> w111
              tunnel: [w125 w133] -> w113
              tunnel: w112 -> [w124 w132]
              tunnel: w119 -> [w123 _]
              tunnel: w114 -> [w122 _]
              tunnel: w107 -> [w121 _]
              frame No Error {
                n45 = Bundle By Name(cluster=T12 {"ModuleType"=enum."PMU", "ModuleID"=0, "UsrEvtRef"=variant, "ScriptCmd"=""} ("GetBdcstData"), "UsrEvtRef"=w121, "ModuleID"=w123, "ModuleType"=ModuleType."PMU", "ScriptCmd"=w122) -> (w129:T12)
                n46 = call "Enqueue.vi"("Priority (f)"=TRUE, "ErrorArray"=w124, "Data"=w129, "Msg"="GetBroadcast") -> ("ErrorArray"=w128:errorcluster[])  [unwired: 7 in]
              }
              frame Error {
              }
            }
            n47 = call <userlib>:"AddError.vi"("Severity"="Abort" ("String"), "Priority"=u8 3, "ErrorArray"=w111, "error in (no error)"=w113) -> ("ErrorArray"=w116:errorcluster[])  [unwired: 6 in, 1 out]
          }
          frame "LoadNetImpairPlugin" {
            n48 = Unbundle By Name(w147) -> ("NetworkImpairModuleID"=w143:i32)
            n49 = Variant To Data(type=T1 {"BusNumber"=0, "EvtPluginINIFilePath"=path "", "EvtParams"=[], "EvtConfig"={"UTC Time 0"=timestamp(0 s since 1904-01-01), "Nominal Frequency"=60, "Reporting Rate"=60, "Fsamp"=960, "PosSeq"=FALSE}, "Start Time"=0.0, "End Time"=0.0, "PmuImpairPluginINIFilePath"=path "", "PmuImpairParams "=[["960"], ["8.19"], ["164"]], "PmuImpairConfig"={"FilterType"="", "bPosSeq"=TRUE}, "NetImpPluginINIFilePath"=path "", "NetImpParams"=[], "FlagImpPluginINIFilePath"=path "", "FlagImpParams"=[], "EvtReportArray"=[], "EventSignalArray"=[], "ImpairReportArray"=[], "NetworkTime"=[], "PktLoss"=[], "FlagImpArray"=[], "OutputToFilePluginINIFilePath"=path "", "Output File Path"=path "", "clConfigOptions"={"TIME_BASE"=1000000, "STN"="Bus_1", "IDCODE"=0, "rdoPolRect"=enum."Rectangular", "rdoFloatInt"=enum."Float", "PHUNIT"=1000000, "rdoFreqDfreq"=enum."Float", "CHNAM"=["VA", "VB", "VC", "V+", "IA", "IB", "IC", "I+"], "chkCfg2Prefix"=TRUE}, "AppPluginINIFilePath"=path "", "AppConfig"=variant, "AppOutput"=variant} ("clBusData"), Variant=w145) -> (data=w144:T1, error out=w138:errorcluster)  [unwired: 1 in]
            n50 = Unbundle By Name(w144) -> ("NetImpPluginINIFilePath"=w135:path)
            n51 = call "LoadPluginRequest.vi"("error in (no error)"=w138, "PathToPlugin"=w135, "ModuleID"=w143) -> ("error out"=w137:errorcluster)  [unwired: 8 in]
            n52 = in-place {
              in-place-border: w135 -> [w148]
              n53 = in-place-cluster #3(w136) -> ()  [unwired: 1 out]
              n54 = in-place-cluster #3("NetImpPluginINIFilePath"=w148) -> (w134:T1)
            }
            n55 = call <userlib>:"AddError.vi"("Severity"="Abort" ("String"), "Priority"=u8 3, "ErrorArray"=w139, "error in (no error)"=w137) -> ("ErrorArray"=w140:errorcluster[])  [unwired: 6 in, 1 out]
          }
          frame "ReadNetImpairPluginPath" {
            n56 = Unbundle By Name(w163) -> ("NetworkImpairModuleID"=w162:i32)
            n57 = call "ObtainBroadcastForRegistration.vi"() -> ("error out"=w152:errorcluster, "NetImpBroadcast"=w151:T18)  [unwired: 10 in]
            n58 = register-events(error in=w152, w151) -> (reference out=w149:refnum<event-registration>, error out=w150:errorcluster)  [unwired: 1 in]
            n59 = call "ReadPathToPluginRequest.vi"("error in (no error)"=w150, "ModuleID"=w162) -> ("error out"=w153:errorcluster)  [unwired: 9 in]
            n60 = case shown="No Error" w153 {
              selector: w153 -> [w168 w176]
              tunnel: [w171 w175] -> w154
              tunnel: [w168 w176] -> w158
              tunnel: w155 -> [w167 w175]
              tunnel: w162 -> [w166 _]
              tunnel: w156 -> [w165 _]
              tunnel: w149 -> [w164 _]
              frame No Error {
                n61 = Bundle By Name(cluster=T12 {"ModuleType"=enum."PMU", "ModuleID"=0, "UsrEvtRef"=variant, "ScriptCmd"=""} ("GetBdcstData"), "UsrEvtRef"=w164, "ModuleID"=w166, "ModuleType"=ModuleType."Network", "ScriptCmd"=w165) -> (w172:T12)
                n62 = call "Enqueue.vi"("Priority (f)"=TRUE, "ErrorArray"=w167, "Data"=w172, "Msg"="GetBroadcast") -> ("ErrorArray"=w171:errorcluster[])  [unwired: 7 in]
              }
              frame Error {
              }
            }
            n63 = call <userlib>:"AddError.vi"("Severity"="Abort" ("String"), "Priority"=u8 3, "ErrorArray"=w154, "error in (no error)"=w158) -> ("ErrorArray"=w159:errorcluster[])  [unwired: 6 in, 1 out]
          }
          frame "LoadFlagImpairPlugin" {
            n64 = Unbundle By Name(w190) -> ("FlagImpairModuleID"=w186:i32)
            n65 = Variant To Data(type=T1 {"BusNumber"=0, "EvtPluginINIFilePath"=path "", "EvtParams"=[], "EvtConfig"={"UTC Time 0"=timestamp(0 s since 1904-01-01), "Nominal Frequency"=60, "Reporting Rate"=60, "Fsamp"=960, "PosSeq"=FALSE}, "Start Time"=0.0, "End Time"=0.0, "PmuImpairPluginINIFilePath"=path "", "PmuImpairParams "=[["960"], ["8.19"], ["164"]], "PmuImpairConfig"={"FilterType"="", "bPosSeq"=TRUE}, "NetImpPluginINIFilePath"=path "", "NetImpParams"=[], "FlagImpPluginINIFilePath"=path "", "FlagImpParams"=[], "EvtReportArray"=[], "EventSignalArray"=[], "ImpairReportArray"=[], "NetworkTime"=[], "PktLoss"=[], "FlagImpArray"=[], "OutputToFilePluginINIFilePath"=path "", "Output File Path"=path "", "clConfigOptions"={"TIME_BASE"=1000000, "STN"="Bus_1", "IDCODE"=0, "rdoPolRect"=enum."Rectangular", "rdoFloatInt"=enum."Float", "PHUNIT"=1000000, "rdoFreqDfreq"=enum."Float", "CHNAM"=["VA", "VB", "VC", "V+", "IA", "IB", "IC", "I+"], "chkCfg2Prefix"=TRUE}, "AppPluginINIFilePath"=path "", "AppConfig"=variant, "AppOutput"=variant} ("clBusData"), Variant=w188) -> (data=w187:T1, error out=w181:errorcluster)  [unwired: 1 in]
            n66 = Unbundle By Name(w187) -> ("FlagImpPluginINIFilePath"=w177:path)
            n67 = call "LoadPluginRequest.vi"("error in (no error)"=w181, "PathToPlugin"=w177, "ModuleID"=w186) -> ("error out"=w180:errorcluster)  [unwired: 8 in]
            n68 = in-place {
              in-place-border: w177 -> [w191]
              n69 = in-place-cluster #4(w179) -> ()  [unwired: 1 out]
              n70 = in-place-cluster #4("FlagImpPluginINIFilePath"=w191) -> (w178:T1)
            }
            n71 = call <userlib>:"AddError.vi"("Severity"="Abort" ("String"), "Priority"=u8 3, "ErrorArray"=w182, "error in (no error)"=w180) -> ("ErrorArray"=w183:errorcluster[])  [unwired: 6 in, 1 out]
          }
          frame "ReadFlagImpairPluginPath" {
            n72 = Unbundle By Name(w206) -> ("FlagImpairModuleID"=w205:i32)
            n73 = call "ObtainBroadcastForRegistration.vi"() -> ("error out"=w195:errorcluster, "FlagImpairBroadcasts"=w194:T19)  [unwired: 10 in]
            n74 = register-events(error in=w195, w194) -> (reference out=w192:refnum<event-registration>, error out=w193:errorcluster)  [unwired: 1 in]
            n75 = call "ReadPluginINIFilePathRequest.vi"("error in (no error)"=w193, "ModuleID"=w205) -> ("error out"=w196:errorcluster)  [unwired: 9 in]
            n76 = case shown="No Error" w196 {
              selector: w196 -> [w211 w219]
              tunnel: [w214 w218] -> w197
              tunnel: [w211 w219] -> w201
              tunnel: w198 -> [w210 w218]
              tunnel: w205 -> [w209 _]
              tunnel: w199 -> [w208 _]
              tunnel: w192 -> [w207 _]
              frame No Error {
                n77 = Bundle By Name(cluster=T12 {"ModuleType"=enum."PMU", "ModuleID"=0, "UsrEvtRef"=variant, "ScriptCmd"=""} ("GetBdcstData"), "UsrEvtRef"=w207, "ModuleID"=w209, "ModuleType"=ModuleType."Flag", "ScriptCmd"=w208) -> (w215:T12)
                n78 = call "Enqueue.vi"("Priority (f)"=TRUE, "ErrorArray"=w210, "Data"=w215, "Msg"="GetBroadcast") -> ("ErrorArray"=w214:errorcluster[])  [unwired: 7 in]
              }
              frame Error {
              }
            }
            n79 = call <userlib>:"AddError.vi"("Severity"="Abort" ("String"), "Priority"=u8 3, "ErrorArray"=w197, "error in (no error)"=w201) -> ("ErrorArray"=w202:errorcluster[])  [unwired: 6 in, 1 out]
          }
          frame "LoadOutputToFilePlugin" {
            n80 = Variant To Data(type=T1 {"BusNumber"=0, "EvtPluginINIFilePath"=path "", "EvtParams"=[], "EvtConfig"={"UTC Time 0"=timestamp(0 s since 1904-01-01), "Nominal Frequency"=60, "Reporting Rate"=60, "Fsamp"=960, "PosSeq"=FALSE}, "Start Time"=0.0, "End Time"=0.0, "PmuImpairPluginINIFilePath"=path "", "PmuImpairParams "=[["960"], ["8.19"], ["164"]], "PmuImpairConfig"={"FilterType"="", "bPosSeq"=TRUE}, "NetImpPluginINIFilePath"=path "", "NetImpParams"=[], "FlagImpPluginINIFilePath"=path "", "FlagImpParams"=[], "EvtReportArray"=[], "EventSignalArray"=[], "ImpairReportArray"=[], "NetworkTime"=[], "PktLoss"=[], "FlagImpArray"=[], "OutputToFilePluginINIFilePath"=path "", "Output File Path"=path "", "clConfigOptions"={"TIME_BASE"=1000000, "STN"="Bus_1", "IDCODE"=0, "rdoPolRect"=enum."Rectangular", "rdoFloatInt"=enum."Float", "PHUNIT"=1000000, "rdoFreqDfreq"=enum."Float", "CHNAM"=["VA", "VB", "VC", "V+", "IA", "IB", "IC", "I+"], "chkCfg2Prefix"=TRUE}, "AppPluginINIFilePath"=path "", "AppConfig"=variant, "AppOutput"=variant} ("clBusData"), Variant=w231) -> (data=w229:T1, error out=w227:errorcluster)  [unwired: 1 in]
            n81 = Unbundle By Name(w233) -> ("OutputToFileModuleID"=w228:i32)
            n82 = Unbundle By Name(w229) -> ("OutputToFilePluginINIFilePath"=w220:path)
            n83 = call "LoadPluginRequest.vi"("error in (no error)"=w227, "PathToPlugin"=w220, "Numeric"=w228) -> ("error out"=w222:errorcluster)  [unwired: 8 in]
            n84 = in-place {
              in-place-border: w220 -> [w234]
              n85 = in-place-cluster #5(w232) -> ()  [unwired: 1 out]
              n86 = in-place-cluster #5("OutputToFilePluginINIFilePath"=w234) -> (w226:T1)
            }
            n87 = call <userlib>:"AddError.vi"("Severity"="Abort" ("String"), "Priority"=u8 3, "ErrorArray"=w221, "error in (no error)"=w222) -> ("ErrorArray"=w223:errorcluster[])  [unwired: 6 in, 1 out]
          }
          frame "ReadOutToFilePluginPath" {
            n88 = Unbundle By Name(w248) -> ("OutputToFileModuleID"=w247:i32)
            n89 = call "ObtainBroadcastForRegistration.vi"() -> ("error out"=w237:errorcluster, "OutputToFileBroadcast"=w236:T20)  [unwired: 10 in]
            n90 = register-events(w236) -> (reference out=w235:refnum<event-registration>)  [unwired: 2 in, 1 out]
            n91 = call "ReadPathToPluginRequest.vi"("error in (no error)"=w237, "ModuleID"=w247) -> ("error out"=w238:errorcluster)  [unwired: 9 in]
            n92 = case shown="No Error" w238 {
              selector: w238 -> [w253 w261]
              tunnel: [w256 w260] -> w239
              tunnel: [w253 w261] -> w243
              tunnel: w240 -> [w252 w260]
              tunnel: w247 -> [w251 _]
              tunnel: w235 -> [w250 _]
              tunnel: w241 -> [w249 _]
              frame No Error {
                n93 = Bundle By Name(cluster=T12 {"ModuleType"=enum."PMU", "ModuleID"=0, "UsrEvtRef"=variant, "ScriptCmd"=""} ("GetBdcstData"), "UsrEvtRef"=w250, "ModuleID"=w251, "ModuleType"=ModuleType."OutToFile", "ScriptCmd"=w249) -> (w257:T12)
                n94 = call "Enqueue.vi"("Priority (f)"=TRUE, "ErrorArray"=w252, "Data"=w257, "Msg"="GetBroadcast") -> ("ErrorArray"=w256:errorcluster[])  [unwired: 7 in]
              }
              frame Error {
              }
            }
            n95 = call <userlib>:"AddError.vi"("Severity"="Abort" ("String"), "Priority"=u8 3, "ErrorArray"=w239, "error in (no error)"=w243) -> ("ErrorArray"=w244:errorcluster[])  [unwired: 6 in, 1 out]
          }
          frame "LoadAppPlugin" {
            n96 = Variant To Data(type=T1 {"BusNumber"=0, "EvtPluginINIFilePath"=path "", "EvtParams"=[], "EvtConfig"={"UTC Time 0"=timestamp(0 s since 1904-01-01), "Nominal Frequency"=60, "Reporting Rate"=60, "Fsamp"=960, "PosSeq"=FALSE}, "Start Time"=0.0, "End Time"=0.0, "PmuImpairPluginINIFilePath"=path "", "PmuImpairParams "=[["960"], ["8.19"], ["164"]], "PmuImpairConfig"={"FilterType"="", "bPosSeq"=TRUE}, "NetImpPluginINIFilePath"=path "", "NetImpParams"=[], "FlagImpPluginINIFilePath"=path "", "FlagImpParams"=[], "EvtReportArray"=[], "EventSignalArray"=[], "ImpairReportArray"=[], "NetworkTime"=[], "PktLoss"=[], "FlagImpArray"=[], "OutputToFilePluginINIFilePath"=path "", "Output File Path"=path "", "clConfigOptions"={"TIME_BASE"=1000000, "STN"="Bus_1", "IDCODE"=0, "rdoPolRect"=enum."Rectangular", "rdoFloatInt"=enum."Float", "PHUNIT"=1000000, "rdoFreqDfreq"=enum."Float", "CHNAM"=["VA", "VB", "VC", "V+", "IA", "IB", "IC", "I+"], "chkCfg2Prefix"=TRUE}, "AppPluginINIFilePath"=path "", "AppConfig"=variant, "AppOutput"=variant} ("clBusData"), Variant=w273) -> (data=w272:T1, error out=w266:errorcluster)  [unwired: 1 in]
            n97 = Unbundle By Name(w275) -> ("AppModuleID"=w271:i32)
            n98 = Unbundle By Name(w272) -> ("AppPluginINIFilePath"=w263:path)
            n99 = call "LoadPluginEvent.vi"("error in (no error)"=w266, "PathToPlugin"=w263, "ModuleID"=w271) -> ("error out"=w265:errorcluster)  [unwired: 8 in]
            n100 = in-place {
              in-place-border: w263 -> [w276]
              n101 = in-place-cluster #6(w264) -> ()  [unwired: 1 out]
              n102 = in-place-cluster #6("AppPluginINIFilePath"=w276) -> (w262:T1)
            }
            n103 = call <userlib>:"AddError.vi"("Severity"="Abort" ("String"), "Priority"=u8 3, "ErrorArray"=w267, "error in (no error)"=w265) -> ("ErrorArray"=w268:errorcluster[])  [unwired: 6 in, 1 out]
          }
          frame "ReadAppPluginPath" {
            n104 = call "ObtainBroadcastForRegistration.vi"() -> ("error out"=w279:errorcluster, "AppModuleBroadcast"=w278:T21)  [unwired: 10 in]
            n105 = Unbundle By Name(w290) -> ("AppModuleID"=w289:i32)
            n106 = register-events(w278) -> (reference out=w277:refnum<event-registration>)  [unwired: 2 in, 1 out]
            n107 = call "ReadPathToIniRequest.vi"("error in (no error)"=w279, "ModuleID"=w289) -> ("error out"=w280:errorcluster)  [unwired: 9 in]
            n108 = case shown="No Error" w280 {
              selector: w280 -> [w295 w303]
              tunnel: [w298 w302] -> w281
              tunnel: [w295 w303] -> w285
              tunnel: w282 -> [w294 w302]
              tunnel: w289 -> [w293 _]
              tunnel: w277 -> [w292 _]
              tunnel: w283 -> [w291 _]
              frame No Error {
                n109 = Bundle By Name(cluster=T12 {"ModuleType"=enum."PMU", "ModuleID"=0, "UsrEvtRef"=variant, "ScriptCmd"=""} ("GetBdcstData"), "UsrEvtRef"=w292, "ModuleID"=w293, "ModuleType"=ModuleType."App", "ScriptCmd"=w291) -> (w299:T12)
                n110 = call "Enqueue.vi"("Priority (f)"=TRUE, "ErrorArray"=w294, "Data"=w299, "Msg"="GetBroadcast") -> ("ErrorArray"=w298:errorcluster[])  [unwired: 7 in]
              }
              frame Error {
              }
            }
            n111 = call <userlib>:"AddError.vi"("Severity"="Abort" ("String"), "Priority"=u8 3, "ErrorArray"=w281, "error in (no error)"=w285) -> ("ErrorArray"=w286:errorcluster[])  [unwired: 6 in, 1 out]
          }
          frame "PopulateEvtFrontPanel" {
            n112 = Unbundle By Name(w304) -> ("EvtPluginINIFilePath"=w326:path)
            n113 = Variant To Data(type=T13 {"TestFilePathRef"=refnum, "BusNumberRef"=refnum, "NumberOfBusesRef"=refnum, "EvtTypeRef"=refnum, "EvtParamsRef"=refnum, "EvtConfigRef"=refnum, "StartTimeRef"=refnum, "EndTimeRef"=refnum, "PmuImpairTypeRef"=refnum, "PmuImpairParamsRef"=refnum, "NetImpairParamsRef"=refnum, "FlagImpairTypeRef"=refnum, "FlagImpairParamsRef"=refnum, "NetImpairTypeRef"=refnum, "OutputFileType"=refnum, "PmuImpairConfigRef"=refnum, "AppTypeRef"=refnum, "ScriptPathRef"=refnum, "ShowPanels?"=refnum} ("clFrontPanelControlRefs"), Variant=w337) -> (data=w318:T13, error out=w332:errorcluster)  [unwired: 1 in]
            n114 = Unbundle By Name(w318) -> ("EvtParamsRef"=w328:refnum<vi>, "EvtTypeRef"=w335:refnum<vi>)
            n115 = call <userlib>:"AddError.vi"("Severity"="Abort" ("String"), "Priority"=u8 3, "ErrorArray"=w331, "error in (no error)"=w332) -> ("ErrorArray"=w330:errorcluster[])  [unwired: 6 in, 1 out]
            n116 = call "GetSetFrameworkData.vi"("Set (F)"=FALSE ("Set/Get")) -> ("clFrameworkData Out"=w324:T22)  [unwired: 10 in]
            n117 = Unbundle By Name(w324) -> ("EvtINIFilePaths"=w323:path[])
            n118 = Unbundle By Name(w304) -> ("EvtParams"=w322:string[][])
            n119 = call "SetFrontPanelTypeRingFromPluginINIFile.vi"("ErrorArray In"=w330, "INIFilePath"=w326, "TypeRef In"=w335) -> ("ErrorArray Out"=w327:errorcluster[], "TypeRef Out"=w329:refnum<vi>)  [unwired: 7 in]
            n120 = call "UpdateParamsHeaders.vi"("ErrorArray In"=w327, "INIFilePaths (from Framework Data)"=w323, "ParamsRef In"=w328, "TypeRef"=w329) -> ("ErrorArray Out"=w307:errorcluster[], "ParamsRef Out"=w321:refnum<vi>)  [unwired: 6 in]
            n121 = Unbundle By Name(w304) -> ("EvtConfig"=w319:T2)
            n122 = Unbundle By Name(w318) -> ("EvtConfigRef"=w320:refnum<vi>)
            n123 = property class="Tbl (strict)"(reference=w321, "Value"=w322) -> (error out=w310:errorcluster)  [unwired: 1 in, 1 out]
            n124 = property class="Clust (strict)"(reference=w320, "Value"=w319) -> (error out=w311:errorcluster)  [unwired: 1 in, 1 out]
            n125 = Unbundle By Name(w318) -> ("StartTimeRef"=w317:refnum<vi>, "EndTimeRef"=w316:refnum<vi>)
            n126 = Unbundle By Name(w304) -> ("Start Time"=w315:dbl, "End Time"=w314:dbl)
            n127 = property class="DigNum (strict)"(reference=w317, "Value"=w315) -> (error out=w312:errorcluster)  [unwired: 1 in, 1 out]
            n128 = property class="DigNum (strict)"(reference=w316, "Value"=w314) -> (error out=w313:errorcluster)  [unwired: 1 in, 1 out]
            n129 = Merge Errors(w312, w313, w311, w310) -> (w306:errorcluster)
            n130 = call <userlib>:"AddError.vi"("Severity"="Abort" ("String"), "Priority"=u8 3, "ErrorArray"=w307, "error in (no error)"=w306) -> ("ErrorArray"=w305:errorcluster[])  [unwired: 6 in, 1 out]
          }
          frame "PopulatePmuImpairFrontPanel" {
            # "Get the path to the module's plugin's .ini file.\nThen, set the event type from the .ini file and\nupdate the Params row and column headers."
            n131 = Unbundle By Name(w341) -> ("PmuImpairConfig"=w349:T3, "PmuImpairParams"=w351:string[][], "PmuImpairPluginINIFilePath"=w357:path)
            n132 = Variant To Data(type=T13 {"TestFilePathRef"=refnum, "BusNumberRef"=refnum, "NumberOfBusesRef"=refnum, "EvtTypeRef"=refnum, "EvtParamsRef"=refnum, "EvtConfigRef"=refnum, "StartTimeRef"=refnum, "EndTimeRef"=refnum, "PmuImpairTypeRef"=refnum, "PmuImpairParamsRef"=refnum, "NetImpairParamsRef"=refnum, "FlagImpairTypeRef"=refnum, "FlagImpairParamsRef"=refnum, "NetImpairTypeRef"=refnum, "OutputFileType"=refnum, "PmuImpairConfigRef"=refnum, "AppTypeRef"=refnum, "ScriptPathRef"=refnum, "ShowPanels?"=refnum} ("clFrontPanelControlRefs"), Variant=w361) -> (data=w359:T13, error out=w348:errorcluster)  [unwired: 1 in]
            n133 = Unbundle By Name(w359) -> ("PmuImpairConfigRef"=w350:refnum<vi>, "PmuImpairTypeRef"=w358:refnum<vi>, "PmuImpairParamsRef"=w353:refnum<vi>)
            n134 = call "GetSetFrameworkData.vi"("Set (F)"=FALSE ("Set/Get")) -> ("clFrameworkData Out"=w356:T22)  [unwired: 10 in]
            n135 = Unbundle By Name(w356) -> ("PmuImpairINIFilePaths"=w354:path[])
            n136 = call "SetFrontPanelTypeRingFromPluginINIFile.vi"("ErrorArray In"=w339, "INIFilePath"=w357, "TypeRef In"=w358) -> ("ErrorArray Out"=w340:errorcluster[], "TypeRef Out"=w355:refnum<vi>)  [unwired: 7 in]
            n137 = call "UpdateParamsHeaders.vi"("ErrorArray In"=w340, "INIFilePaths (from Framework Data)"=w354, "ParamsRef In"=w353, "TypeRef"=w355) -> ("ErrorArray Out"=w338:errorcluster[], "ParamsRef Out"=w352:refnum<vi>)  [unwired: 6 in]
            n138 = property class="Tbl (strict)"(reference=w352, error in=w348, "Value"=w351) -> (error out=w347:errorcluster)  [unwired: 1 out]
            n139 = property class="Clust (strict)"(reference=w350, error in=w347, "Value"=w349) -> (error out=w342:errorcluster)  [unwired: 1 out]
            n140 = call <userlib>:"AddError.vi"("Severity"="Abort" ("String"), "Priority"=u8 3, "ErrorArray"=w338, "error in (no error)"=w342) -> ("ErrorArray"=w343:errorcluster[])  [unwired: 6 in, 1 out]
          }
          frame "PopulateNetImpairFrontPanel" {
            n141 = Unbundle By Name(w374) -> ("NetImpParams"=w379:string[][], "NetImpPluginINIFilePath"=w371:path)
            n142 = Variant To Data(type=T13 {"TestFilePathRef"=refnum, "BusNumberRef"=refnum, "NumberOfBusesRef"=refnum, "EvtTypeRef"=refnum, "EvtParamsRef"=refnum, "EvtConfigRef"=refnum, "StartTimeRef"=refnum, "EndTimeRef"=refnum, "PmuImpairTypeRef"=refnum, "PmuImpairParamsRef"=refnum, "NetImpairParamsRef"=refnum, "FlagImpairTypeRef"=refnum, "FlagImpairParamsRef"=refnum, "NetImpairTypeRef"=refnum, "OutputFileType"=refnum, "PmuImpairConfigRef"=refnum, "AppTypeRef"=refnum, "ScriptPathRef"=refnum, "ShowPanels?"=refnum} ("clFrontPanelControlRefs"), Variant=w382) -> (data=w380:T13, error out=w370:errorcluster)  [unwired: 1 in]
            n143 = call "GetSetFrameworkData.vi"("Set (F)"=FALSE) -> ("clFrameworkData Out"=w373:T22)  [unwired: 10 in]
            n144 = Unbundle By Name(w380) -> ("NetImpairParamsRef"=w364:refnum<vi>, "NetImpairTypeRef"=w372:refnum<vi>)
            n145 = Unbundle By Name(w373) -> ("NetImpairINIFilePaths"=w365:path[])
            n146 = call "SetFrontPanelTypeRingFromPluginINIFile.vi"("ErrorArray In"=w369, "INIFilePath"=w371, "TypeRef In"=w372) -> ("ErrorArray Out"=w367:errorcluster[], "TypeRef Out"=w368:refnum<vi>)  [unwired: 7 in]
            n147 = call "UpdateParamsHeaders.vi"("ErrorArray In"=w367, "INIFilePaths (from Framework Data)"=w365, "ParamsRef In"=w364, "TypeRef"=w368) -> ("ErrorArray Out"=w366:errorcluster[], "ParamsRef Out"=w363:refnum<vi>)  [unwired: 6 in]
            n148 = property class="Tbl (strict)"(reference=w363, error in=w370, "Value"=w379) -> (error out=w375:errorcluster)  [unwired: 1 out]
            n149 = call <userlib>:"AddError.vi"("Severity"="Abort" ("String"), "Priority"=u8 3, "ErrorArray"=w366, "error in (no error)"=w375) -> ("ErrorArray"=w376:errorcluster[])  [unwired: 6 in, 1 out]
          }
          frame "PopulateFlagImpairFrontPanel" {
            # "Get the path to the module's plugin's .ini file.\nThen, set the event type from the .ini file and\nupdate the Params row and column headers."
            n150 = Variant To Data(type=T13 {"TestFilePathRef"=refnum, "BusNumberRef"=refnum, "NumberOfBusesRef"=refnum, "EvtTypeRef"=refnum, "EvtParamsRef"=refnum, "EvtConfigRef"=refnum, "StartTimeRef"=refnum, "EndTimeRef"=refnum, "PmuImpairTypeRef"=refnum, "PmuImpairParamsRef"=refnum, "NetImpairParamsRef"=refnum, "FlagImpairTypeRef"=refnum, "FlagImpairParamsRef"=refnum, "NetImpairTypeRef"=refnum, "OutputFileType"=refnum, "PmuImpairConfigRef"=refnum, "AppTypeRef"=refnum, "ScriptPathRef"=refnum, "ShowPanels?"=refnum} ("clFrontPanelControlRefs"), Variant=w402) -> (data=w400:T13, error out=w391:errorcluster)  [unwired: 1 in]
            n151 = Unbundle By Name(w384) -> ("FlagImpParams"=w392:string[][], "FlagImpPluginINIFilePath"=w398:path)
            n152 = Unbundle By Name(w400) -> ("FlagImpairTypeRef"=w399:refnum<vi>, "FlagImpairParamsRef"=w394:refnum<vi>)
            n153 = call "GetSetFrameworkData.vi"("Set (F)"=FALSE ("Set/Get")) -> ("clFrameworkData Out"=w397:T22)  [unwired: 10 in]
            n154 = Unbundle By Name(w397) -> ("FlagImpairINIFilePaths"=w395:path[])
            n155 = call "SetFrontPanelTypeRingFromPluginINIFile.vi"("INIFilePath"=w398, "TypeRef In"=w399) -> ("TypeRef Out"=w396:refnum<vi>)  [unwired: 8 in, 1 out]
            n156 = call "UpdateParamsHeaders.vi"("INIFilePaths (from Framework Data)"=w395, "ParamsRef In"=w394, "TypeRef"=w396) -> ("ParamsRef Out"=w393:refnum<vi>)  [unwired: 7 in, 1 out]
            n157 = property class="Tbl (strict)"(reference=w393, error in=w391, "Value"=w392) -> (error out=w383:errorcluster)  [unwired: 1 out]
            n158 = call <userlib>:"AddError.vi"("Severity"="Abort" ("String"), "Priority"=u8 3, "ErrorArray"=w385, "error in (no error)"=w383) -> ("ErrorArray"=w386:errorcluster[], "error out"=w387:errorcluster)  [unwired: 6 in]
            n159 = call <vilib>:"Clear Errors.vi"("error in (no error)"=w387) -> ()  [unwired: 5 in, 2 out]
          }
          frame "PopulateAppFrontPanel" {
            n160 = Variant To Data(type=T13 {"TestFilePathRef"=refnum, "BusNumberRef"=refnum, "NumberOfBusesRef"=refnum, "EvtTypeRef"=refnum, "EvtParamsRef"=refnum, "EvtConfigRef"=refnum, "StartTimeRef"=refnum, "EndTimeRef"=refnum, "PmuImpairTypeRef"=refnum, "PmuImpairParamsRef"=refnum, "NetImpairParamsRef"=refnum, "FlagImpairTypeRef"=refnum, "FlagImpairParamsRef"=refnum, "NetImpairTypeRef"=refnum, "OutputFileType"=refnum, "PmuImpairConfigRef"=refnum, "AppTypeRef"=refnum, "ScriptPathRef"=refnum, "ShowPanels?"=refnum} ("clFrontPanelControlRefs"), Variant=w414) -> (data=w412:T13, error out=w405:errorcluster)  [unwired: 1 in]
            n161 = Unbundle By Name(w406) -> ("AppPluginINIFilePath"=w410:path)
            n162 = Unbundle By Name(w412) -> ("AppTypeRef"=w411:refnum<vi>)
            n163 = call "SetFrontPanelTypeRingFromPluginINIFile.vi"("ErrorArray In"=w404, "INIFilePath"=w410, "TypeRef In"=w411) -> ("ErrorArray Out"=w403:errorcluster[])  [unwired: 7 in, 1 out]
            n164 = call <userlib>:"AddError.vi"("Severity"="Abort" ("String"), "Priority"=u8 3, "ErrorArray"=w403, "error in (no error)"=w405) -> ("ErrorArray"=w407:errorcluster[])  [unwired: 6 in, 1 out]
          }
          frame "PopulateOutToFileFrontPanel" {
            n165 = Unbundle By Name(w418) -> ("OutputToFilePluginINIFilePath"=w422:path)
            n166 = Variant To Data(type=T13 {"TestFilePathRef"=refnum, "BusNumberRef"=refnum, "NumberOfBusesRef"=refnum, "EvtTypeRef"=refnum, "EvtParamsRef"=refnum, "EvtConfigRef"=refnum, "StartTimeRef"=refnum, "EndTimeRef"=refnum, "PmuImpairTypeRef"=refnum, "PmuImpairParamsRef"=refnum, "NetImpairParamsRef"=refnum, "FlagImpairTypeRef"=refnum, "FlagImpairParamsRef"=refnum, "NetImpairTypeRef"=refnum, "OutputFileType"=refnum, "PmuImpairConfigRef"=refnum, "AppTypeRef"=refnum, "ScriptPathRef"=refnum, "ShowPanels?"=refnum} ("clFrontPanelControlRefs"), Variant=w426) -> (data=w424:T13, error out=w417:errorcluster)  [unwired: 1 in]
            n167 = Unbundle By Name(w424) -> ("OutputFileType"=w423:refnum<vi>)
            n168 = call "SetFrontPanelTypeRingFromPluginINIFile.vi"("ErrorArray In"=w416, "INIFilePath"=w422, "TypeRef In"=w423) -> ("ErrorArray Out"=w415:errorcluster[])  [unwired: 7 in, 1 out]
            n169 = call <userlib>:"AddError.vi"("Severity"="Abort" ("String"), "Priority"=u8 3, "ErrorArray"=w415, "error in (no error)"=w417) -> ("ErrorArray"=w419:errorcluster[])  [unwired: 6 in, 1 out]
          }
          frame "StripIniPaths" {
            n170 = in-place {
              n171 = in-place-cluster #7(w428) -> ("EvtPluginINIFilePath"=w459:path, "PmuImpairPluginINIFilePath"=w461:path, "NetImpPluginINIFilePath"=w463:path, "FlagImpPluginINIFilePath"=w465:path, "OutputToFilePluginINIFilePath"=w471:path, "AppPluginINIFilePath"=w434:path)
              n172 = Strip Path(path=w471) -> (stripped path=w469:path, name=w467:string)
              n173 = Strip Path(path=w434) -> (stripped path=w430:path, name=w436:string)
              n174 = Strip Path(path=w459) -> (stripped path=w460:path, name=w442:string)
              n175 = Strip Path(path=w465) -> (stripped path=w466:path, name=w448:string)
              n176 = Strip Path(path=w461) -> (stripped path=w462:path, name=w444:string)
              n177 = Strip Path(path=w463) -> (stripped path=w464:path, name=w446:string)
              n178 = Strip Path(path=w469) -> (name=w458:string)  [unwired: 1 out]
              n179 = Strip Path(path=w430) -> (name=w433:string)  [unwired: 1 out]
              n180 = Strip Path(path=w460) -> (name=w441:string)  [unwired: 1 out]
              n181 = Strip Path(path=w466) -> (name=w447:string)  [unwired: 1 out]
              n182 = Strip Path(path=w462) -> (name=w443:string)  [unwired: 1 out]
              n183 = Strip Path(path=w464) -> (name=w445:string)  [unwired: 1 out]
              n184 = Concatenate Strings(w458, "\\" ("string"), w467) -> (w468:string)
              n185 = Concatenate Strings(w433, "\\" ("string"), w436) -> (w435:string)
              n186 = Concatenate Strings(w445, "\\" ("string"), w446) -> (w454:string)
              n187 = Concatenate Strings(w447, "\\" ("string"), w448) -> (w455:string)
              n188 = Concatenate Strings(w443, "\\" ("string"), w444) -> (w451:string)
              n189 = Concatenate Strings(w441, "\\" ("string"), w442) -> (w450:string)
              n190 = String To Path(string=w468) -> (path=w470:path)
              n191 = String To Path(string=w435) -> (path=w432:path)
              n192 = String To Path(string=w454) -> (path=w439:path)
              n193 = String To Path(string=w455) -> (path=w440:path)
              n194 = String To Path(string=w451) -> (path=w438:path)
              n195 = String To Path(string=w450) -> (path=w437:path)
              n196 = in-place-cluster #7("EvtPluginINIFilePath"=w437, "PmuImpairPluginINIFilePath"=w438, "NetImpPluginINIFilePath"=w439, "FlagImpPluginINIFilePath"=w440, "OutputToFilePluginINIFilePath"=w470, "AppPluginINIFilePath"=w432) -> (w427:T1)
            }
          }
          frame "Aggregate" {
            n197 = call "ObtainBroadcastForRegistration.vi"() -> ("error out"=w485:errorcluster, "AppModuleBroadcast"=w484:T21)  [unwired: 10 in]
            n198 = Unbundle By Name(w486) -> ("AppModuleID"=w481:i32)
            n199 = register-events(w484) -> (reference out=w483:refnum<event-registration>)  [unwired: 2 in, 1 out]
            n200 = call "AggregateRequest.vi"("error in (no error)"=w485, "ModuleID"=w481) -> ("error out"=w482:errorcluster)  [unwired: 9 in]
            n201 = while {
              tunnel: w483 -> [w497]
              tunnel: w480 -> [w494]
              tunnel: w482 -> [w496]
              shift-right: [w489] -> w476
              shift-left: w478 -> [w491]
              tunnel: [w487] -> w477
              stop <- w488 stop-if-true
              # "Loop waits for Errors, Completion Msg, or Timeout"
              n202 = event shown="[0] <AppModuleBroadcast.StatusUpdate>: User Event" {
                selector: w497 -> [_ _ _]
                dyn-events: [_ _ _] -> w487
                timeout: 10000 -> [_ _ _]
                tunnel: w496 -> [_ _ w504]
                tunnel: [_ w499 w505] -> w490
                tunnel: w494 -> [_ _ w506]
                tunnel: [TRUE _ TRUE] -> w488
                event User Event {
                  n203 = event-data() -> ()  [unwired: 1 in, 1 out]
                }
                event User Event {
                  n204 = event-data() -> ("Data"=w500:variant)  [unwired: 1 in]
                  n205 = Variant To Data(type=T14 {"error"={"status"=FALSE, "code"=0, "source"=""}, "AdditionalInfo"=""} ("Cluster"), Variant=w500) -> (data=w501:T14)  [unwired: 1 in, 1 out]
                  n206 = Unbundle By Name(w501) -> ("error"=w499:errorcluster)
                }
                event Timeout {
                  n207 = event-data() -> ()  [unwired: 1 in, 1 out]
                  n208 = xnode "Error Ring"("parameter 0"=w506) -> ("error out"=w507:errorcluster)
                  n209 = Merge Errors(w504, w507) -> (w505:errorcluster)
                }
              }
              n210 = call <userlib>:"AddError.vi"("Severity"="Abort" ("String"), "Priority"=u8 3, "ErrorArray"=w491, "error in (no error)"=w490) -> ("ErrorArray"=w489:errorcluster[])  [unwired: 6 in, 1 out]
            }
            n211 = Unregister For Events(event registration refnum=w477) -> (error out=w475:errorcluster)  [unwired: 1 in]
            n212 = call <userlib>:"AddError.vi"("Severity"="Inform", "Priority"=u8 4, "ErrorArray"=w476, "error in (no error)"=w475) -> ("ErrorArray"=w474:errorcluster[])  [unwired: 6 in, 1 out]
          }
          frame "CalcAppOutput" {
            n213 = property class="Bus.lvclass"(reference=w522) -> ("Accessors:AppModuleID"=w521:i32)  [unwired: 1 in, 2 out]
            n214 = call "CalcAppOutputRequest.vi"("ModuleID"=w521) -> ("error out"=w519:errorcluster)  [unwired: 10 in]
            n215 = call <userlib>:"AddError.vi"("Severity"="Abort", "Priority"=u8 3, "ErrorArray"=w520, "error in (no error)"=w519) -> ("ErrorArray"=w515:errorcluster[])  [unwired: 6 in, 1 out]
          }
          frame "GetAppOutput" {
            n216 = call "ObtainBroadcastForRegistration.vi"() -> ("error out"=w535:errorcluster, "AppModuleBroadcast"=w534:T21)  [unwired: 10 in]
            n217 = Unbundle By Name(w536) -> ("AppModuleID"=w525:i32)
            n218 = register-events(w534) -> (reference out=w526:refnum<event-registration>)  [unwired: 2 in, 1 out]
            n219 = call "GetAppOutputRequest.vi"("error in (no error)"=w535, "ModuleID"=w525) -> ("error out"=w527:errorcluster)  [unwired: 9 in]
            n220 = case shown="No Error" w527 {
              selector: w527 -> [w541 w549]
              tunnel: [w544 w548] -> w528
              tunnel: [w541 w549] -> w523
              tunnel: w529 -> [w540 w548]
              tunnel: w525 -> [w539 _]
              tunnel: w526 -> [w538 _]
              tunnel: w524 -> [w537 _]
              frame No Error {
                n221 = Bundle By Name(cluster=T12 {"ModuleType"=enum."PMU", "ModuleID"=0, "UsrEvtRef"=variant, "ScriptCmd"=""} ("GetBdcstData"), "UsrEvtRef"=w538, "ModuleID"=w539, "ModuleType"=ModuleType."App", "ScriptCmd"=w537) -> (w545:T12)
                n222 = call "Enqueue.vi"("Priority (f)"=TRUE, "ErrorArray"=w540, "Data"=w545, "Msg"="GetBroadcast") -> ("ErrorArray"=w544:errorcluster[])  [unwired: 7 in]
              }
              frame Error {
              }
            }
            n223 = call <userlib>:"AddError.vi"("Severity"="Abort" ("String"), "Priority"=u8 3, "ErrorArray"=w528, "error in (no error)"=w523) -> ("ErrorArray"=w531:errorcluster[])  [unwired: 6 in, 1 out]
          }
          frame "ReadAppInputData" {
            n224 = Unbundle By Name(w563) -> ("AppModuleID"=w562:i32)
            n225 = call "ObtainBroadcastForRegistration.vi"() -> ("error out"=w552:errorcluster, "AppModuleBroadcast"=w551:T21)  [unwired: 10 in]
            n226 = register-events(w551) -> (reference out=w550:refnum<event-registration>)  [unwired: 2 in, 1 out]
            n227 = call "ReadAppInputDataRequest.vi"("error in (no error)"=w552, "ModuleID"=w562) -> ("error out"=w553:errorcluster)  [unwired: 9 in]
            n228 = case shown="No Error" w553 {
              selector: w553 -> [w568 w576]
              tunnel: [w571 w575] -> w554
              tunnel: [w568 w576] -> w558
              tunnel: w555 -> [w567 w575]
              tunnel: w562 -> [w566 _]
              tunnel: w550 -> [w565 _]
              tunnel: w556 -> [w564 _]
              frame No Error {
                n229 = Bundle By Name(cluster=T12 {"ModuleType"=enum."PMU", "ModuleID"=0, "UsrEvtRef"=variant, "ScriptCmd"=""} ("GetBdcstData"), "UsrEvtRef"=w565, "ModuleID"=w566, "ModuleType"=ModuleType."App", "ScriptCmd"=w564) -> (w572:T12)
                n230 = call "Enqueue.vi"("Priority (f)"=TRUE, "ErrorArray"=w567, "Data"=w572, "Msg"="GetBroadcast") -> ("ErrorArray"=w571:errorcluster[])  [unwired: 7 in]
              }
              frame Error {
              }
            }
            n231 = call <userlib>:"AddError.vi"("Severity"="Abort" ("String"), "Priority"=u8 3, "ErrorArray"=w554, "error in (no error)"=w558) -> ("ErrorArray"=w559:errorcluster[])  [unwired: 6 in, 1 out]
          }
          frame "WriteAppConfig" {
            # "Write the App Config XML to the App"
            n232 = Variant To Data(type=T1 {"BusNumber"=0, "EvtPluginINIFilePath"=path "", "EvtParams"=[], "EvtConfig"={"UTC Time 0"=timestamp(0 s since 1904-01-01), "Nominal Frequency"=60, "Reporting Rate"=60, "Fsamp"=960, "PosSeq"=FALSE}, "Start Time"=0.0, "End Time"=0.0, "PmuImpairPluginINIFilePath"=path "", "PmuImpairParams "=[["960"], ["8.19"], ["164"]], "PmuImpairConfig"={"FilterType"="", "bPosSeq"=TRUE}, "NetImpPluginINIFilePath"=path "", "NetImpParams"=[], "FlagImpPluginINIFilePath"=path "", "FlagImpParams"=[], "EvtReportArray"=[], "EventSignalArray"=[], "ImpairReportArray"=[], "NetworkTime"=[], "PktLoss"=[], "FlagImpArray"=[], "OutputToFilePluginINIFilePath"=path "", "Output File Path"=path "", "clConfigOptions"={"TIME_BASE"=1000000, "STN"="Bus_1", "IDCODE"=0, "rdoPolRect"=enum."Rectangular", "rdoFloatInt"=enum."Float", "PHUNIT"=1000000, "rdoFreqDfreq"=enum."Float", "CHNAM"=["VA", "VB", "VC", "V+", "IA", "IB", "IC", "I+"], "chkCfg2Prefix"=TRUE}, "AppPluginINIFilePath"=path "", "AppConfig"=variant, "AppOutput"=variant} ("clBusData"), Variant=w593) -> (data=w592:T1, error out=w580:errorcluster)  [unwired: 1 in]
            n233 = Unbundle By Name(w585) -> ("AppModuleID"=w584:i32)
            n234 = Unbundle By Name(w592) -> ("AppConfig"=w577:variant)
            n235 = Variant To Data(error in=w580, type="", Variant=w577) -> (data=w581:string, error out=w579:errorcluster)
            n236 = call "WriteAppConfigRequest.vi"("error in (no error)"=w579, "AppConfigXML"=w581, "ModuleID"=w584) -> ("error out"=w587:errorcluster)  [unwired: 8 in]
            n237 = in-place {
              in-place-border: w577 -> [w595]
              n238 = in-place-cluster #8(w583) -> ()  [unwired: 1 out]
              n239 = in-place-cluster #8("AppConfig"=w595) -> (w582:T1)
            }
            n240 = call <userlib>:"AddError.vi"("Severity"="Abort" ("String"), "Priority"=u8 3, "ErrorArray"=w586, "error in (no error)"=w587) -> ("ErrorArray"=w588:errorcluster[], "error out"=w589:errorcluster)  [unwired: 6 in]
            n241 = call <vilib>:"Clear Errors.vi"("error in (no error)"=w589) -> ()  [unwired: 5 in, 2 out]
          }
          frame "ReadAppConfig" {
            n242 = Unbundle By Name(w609) -> ("AppModuleID"=w608:i32)
            n243 = call "ObtainBroadcastForRegistration.vi"() -> ("error out"=w598:errorcluster, "AppModuleBroadcast"=w597:T21)  [unwired: 10 in]
            n244 = register-events(w597) -> (reference out=w596:refnum<event-registration>)  [unwired: 2 in, 1 out]
            n245 = call "ReadAppConfigRequest.vi"("error in (no error)"=w598, "ModuleID"=w608) -> ("error out"=w599:errorcluster)  [unwired: 9 in]
            n246 = case shown="No Error" w599 {
              selector: w599 -> [w614 w622]
              tunnel: [w617 w621] -> w600
              tunnel: [w614 w622] -> w604
              tunnel: w601 -> [w613 w621]
              tunnel: w608 -> [w612 _]
              tunnel: w596 -> [w611 _]
              tunnel: w602 -> [w610 _]
              frame No Error {
                n247 = Bundle By Name(cluster=T12 {"ModuleType"=enum."PMU", "ModuleID"=0, "UsrEvtRef"=variant, "ScriptCmd"=""} ("GetBdcstData"), "UsrEvtRef"=w611, "ModuleID"=w612, "ModuleType"=ModuleType."App", "ScriptCmd"=w610) -> (w618:T12)
                n248 = call "Enqueue.vi"("Priority (f)"=TRUE, "ErrorArray"=w613, "Data"=w618, "Msg"="GetBroadcast") -> ("ErrorArray"=w617:errorcluster[])  [unwired: 7 in]
              }
              frame Error {
              }
            }
            n249 = call <userlib>:"AddError.vi"("Severity"="Abort" ("String"), "Priority"=u8 3, "ErrorArray"=w600, "error in (no error)"=w604) -> ("ErrorArray"=w605:errorcluster[])  [unwired: 6 in, 1 out]
          }
          frame "ReadOutputFilePath" {
            n250 = Unbundle By Name(w636) -> ("OutputToFileModuleID"=w635:i32)
            n251 = call "ObtainBroadcastForRegistration.vi"() -> ("error out"=w625:errorcluster, "OutputToFileBroadcast"=w624:T20)  [unwired: 10 in]
            n252 = register-events(w624) -> (reference out=w623:refnum<event-registration>)  [unwired: 2 in, 1 out]
            n253 = call "ReadOutputPathRequest.vi"("error in (no error)"=w625, "ModuleID"=w635) -> ("error out"=w626:errorcluster)  [unwired: 9 in]
            n254 = case shown="No Error" w626 {
              selector: w626 -> [w641 w649]
              tunnel: [w644 w648] -> w627
              tunnel: [w641 w649] -> w631
              tunnel: w628 -> [w640 w648]
              tunnel: w635 -> [w639 _]
              tunnel: w623 -> [w638 _]
              tunnel: w629 -> [w637 _]
              frame No Error {
                n255 = Bundle By Name(cluster=T12 {"ModuleType"=enum."PMU", "ModuleID"=0, "UsrEvtRef"=variant, "ScriptCmd"=""} ("GetBdcstData"), "UsrEvtRef"=w638, "ModuleID"=w639, "ModuleType"=ModuleType."OutToFile", "ScriptCmd"=w637) -> (w645:T12)
                n256 = call "Enqueue.vi"("Priority (f)"=TRUE, "ErrorArray"=w640, "Data"=w645, "Msg"="GetBroadcast") -> ("ErrorArray"=w644:errorcluster[])  [unwired: 7 in]
              }
              frame Error {
              }
            }
            n257 = call <userlib>:"AddError.vi"("Severity"="Abort" ("String"), "Priority"=u8 3, "ErrorArray"=w627, "error in (no error)"=w631) -> ("ErrorArray"=w632:errorcluster[])  [unwired: 6 in, 1 out]
          }
          frame "WriteOutputFilePath" {
            n258 = property class="Bus.lvclass"(reference=w659) -> ("Accessors:OutputToFileModuleID"=w658:i32)  [unwired: 1 in, 2 out]
            n259 = Variant To Data(type=T1 {"BusNumber"=0, "EvtPluginINIFilePath"=path "", "EvtParams"=[], "EvtConfig"={"UTC Time 0"=timestamp(0 s since 1904-01-01), "Nominal Frequency"=60, "Reporting Rate"=60, "Fsamp"=960, "PosSeq"=FALSE}, "Start Time"=0.0, "End Time"=0.0, "PmuImpairPluginINIFilePath"=path "", "PmuImpairParams "=[["960"], ["8.19"], ["164"]], "PmuImpairConfig"={"FilterType"="", "bPosSeq"=TRUE}, "NetImpPluginINIFilePath"=path "", "NetImpParams"=[], "FlagImpPluginINIFilePath"=path "", "FlagImpParams"=[], "EvtReportArray"=[], "EventSignalArray"=[], "ImpairReportArray"=[], "NetworkTime"=[], "PktLoss"=[], "FlagImpArray"=[], "OutputToFilePluginINIFilePath"=path "", "Output File Path"=path "", "clConfigOptions"={"TIME_BASE"=1000000, "STN"="Bus_1", "IDCODE"=0, "rdoPolRect"=enum."Rectangular", "rdoFloatInt"=enum."Float", "PHUNIT"=1000000, "rdoFreqDfreq"=enum."Float", "CHNAM"=["VA", "VB", "VC", "V+", "IA", "IB", "IC", "I+"], "chkCfg2Prefix"=TRUE}, "AppPluginINIFilePath"=path "", "AppConfig"=variant, "AppOutput"=variant} ("clBusData"), Variant=w663) -> (data=w660:T1, error out=w657:errorcluster)  [unwired: 1 in]
            n260 = Unbundle By Name(w660) -> ("Output File Path"=w650:path)
            n261 = in-place {
              in-place-border: w650 -> [w664]
              n262 = in-place-cluster #9(w661) -> ()  [unwired: 1 out]
              n263 = in-place-cluster #9("Output File Path"=w664) -> (w651:T1)
            }
            n264 = call "WriteOutputPathRequest.vi"("error in (no error)"=w657, "OutPath"=w650, "ModuleID"=w658) -> ("error out"=w653:errorcluster)  [unwired: 8 in]
            n265 = call <userlib>:"AddError.vi"("Severity"="Abort" ("String"), "Priority"=u8 3, "ErrorArray"=w652, "error in (no error)"=w653) -> ("ErrorArray"=w654:errorcluster[])  [unwired: 6 in, 1 out]
          }
          frame "ReadOutToFileConfig" {
            n266 = Unbundle By Name(w678) -> ("OutputToFileModuleID"=w677:i32)
            n267 = call "ObtainBroadcastForRegistration.vi"() -> ("error out"=w667:errorcluster, "OutputToFileBroadcast"=w666:T20)  [unwired: 10 in]
            n268 = register-events(w666) -> (reference out=w665:refnum<event-registration>)  [unwired: 2 in, 1 out]
            n269 = call "ReadPmuConfigRequest.vi"("error in (no error)"=w667, "ModuleID"=w677) -> ("error out"=w668:errorcluster)  [unwired: 9 in]
            n270 = case shown="No Error" w668 {
              selector: w668 -> [w683 w691]
              tunnel: [w686 w690] -> w669
              tunnel: [w683 w691] -> w673
              tunnel: w670 -> [w682 w690]
              tunnel: w677 -> [w681 _]
              tunnel: w665 -> [w680 _]
              tunnel: w671 -> [w679 _]
              frame No Error {
                n271 = Bundle By Name(cluster=T12 {"ModuleType"=enum."PMU", "ModuleID"=0, "UsrEvtRef"=variant, "ScriptCmd"=""} ("GetBdcstData"), "UsrEvtRef"=w680, "ModuleID"=w681, "ModuleType"=ModuleType."OutToFile", "ScriptCmd"=w679) -> (w687:T12)
                n272 = call "Enqueue.vi"("Priority (f)"=TRUE, "ErrorArray"=w682, "Data"=w687, "Msg"="GetBroadcast") -> ("ErrorArray"=w686:errorcluster[])  [unwired: 7 in]
              }
              frame Error {
              }
            }
            n273 = call <userlib>:"AddError.vi"("Severity"="Abort" ("String"), "Priority"=u8 3, "ErrorArray"=w669, "error in (no error)"=w673) -> ("ErrorArray"=w674:errorcluster[])  [unwired: 6 in, 1 out]
          }
          frame "WriteEvtBusNumber" {
            # "Write the event parameters to the event module"
            n274 = Variant To Data(type=T1 {"BusNumber"=0, "EvtPluginINIFilePath"=path "", "EvtParams"=[], "EvtConfig"={"UTC Time 0"=timestamp(0 s since 1904-01-01), "Nominal Frequency"=60, "Reporting Rate"=60, "Fsamp"=960, "PosSeq"=FALSE}, "Start Time"=0.0, "End Time"=0.0, "PmuImpairPluginINIFilePath"=path "", "PmuImpairParams "=[["960"], ["8.19"], ["164"]], "PmuImpairConfig"={"FilterType"="", "bPosSeq"=TRUE}, "NetImpPluginINIFilePath"=path "", "NetImpParams"=[], "FlagImpPluginINIFilePath"=path "", "FlagImpParams"=[], "EvtReportArray"=[], "EventSignalArray"=[], "ImpairReportArray"=[], "NetworkTime"=[], "PktLoss"=[], "FlagImpArray"=[], "OutputToFilePluginINIFilePath"=path "", "Output File Path"=path "", "clConfigOptions"={"TIME_BASE"=1000000, "STN"="Bus_1", "IDCODE"=0, "rdoPolRect"=enum."Rectangular", "rdoFloatInt"=enum."Float", "PHUNIT"=1000000, "rdoFreqDfreq"=enum."Float", "CHNAM"=["VA", "VB", "VC", "V+", "IA", "IB", "IC", "I+"], "chkCfg2Prefix"=TRUE}, "AppPluginINIFilePath"=path "", "AppConfig"=variant, "AppOutput"=variant} ("clBusData"), Variant=w698) -> (data=w696:T1, error out=w695:errorcluster)  [unwired: 1 in]
            n275 = Unbundle By Name(w700) -> ("EventModuleID"=w699:i32)
            n276 = Unbundle By Name(w696) -> ("BusNumber"=w693:u8)
            n277 = call "WriteBusNumberRequest.vi"("error in (no error)"=w695, "BusNumber"=w693, "ModuleID"=w699) -> ("error out"=w702:errorcluster)  [unwired: 8 in]
            n278 = in-place {
              in-place-border: w693 -> [w706]
              n279 = in-place-cluster #10(w694) -> ()  [unwired: 1 out]
              n280 = in-place-cluster #10("BusNumber"=w706) -> (w692:T1)
            }
            n281 = call <userlib>:"AddError.vi"("Severity"="Abort" ("String"), "Priority"=u8 3, "ErrorArray"=w701, "error in (no error)"=w702) -> ("ErrorArray"=w703:errorcluster[])  [unwired: 6 in, 1 out]
          }
          frame "ReadEvtBusNumber" {
            n282 = call "ObtainBroadcastForRegistration.vi"() -> ("error out"=w713:errorcluster, "EventBroadcast"=w722:T16)  [unwired: 10 in]
            n283 = Unbundle By Name(w721) -> ("EventModuleID"=w709:i32)
            n284 = register-events(error in=w713, w722) -> (reference out=w710:refnum<event-registration>, error out=w712:errorcluster)  [unwired: 1 in]
            n285 = call "ReadBusNumberRequest.vi"("error in (no error)"=w712, "ModuleID"=w709) -> ("error out"=w711:errorcluster)  [unwired: 9 in]
            n286 = case shown="No Error" w711 {
              selector: w711 -> [w727 w735]
              tunnel: [w730 w734] -> w714
              tunnel: [w727 w735] -> w707
              tunnel: w715 -> [w726 w734]
              tunnel: w710 -> [w725 _]
              tunnel: w709 -> [w724 _]
              tunnel: w708 -> [w723 _]
              frame No Error {
                n287 = Bundle By Name(cluster=T12 {"ModuleType"=enum."PMU", "ModuleID"=0, "UsrEvtRef"=variant, "ScriptCmd"=""} ("GetBdcstData"), "UsrEvtRef"=w725, "ModuleID"=w724, "ModuleType"=ModuleType."Event", "ScriptCmd"=w723) -> (w731:T12)
                n288 = call "Enqueue.vi"("Priority (f)"=TRUE, "ErrorArray"=w726, "Data"=w731, "Msg"="GetBroadcast") -> ("ErrorArray"=w730:errorcluster[])  [unwired: 7 in]
              }
              frame Error {
              }
            }
            n289 = call <userlib>:"AddError.vi"("Severity"="Abort" ("String"), "Priority"=u8 3, "ErrorArray"=w714, "error in (no error)"=w707) -> ("ErrorArray"=w717:errorcluster[], "error out"=w718:errorcluster)  [unwired: 6 in]
            n290 = call <vilib>:"Clear Errors.vi"("error in (no error)"=w718) -> ()  [unwired: 5 in, 2 out]
          }
          frame "WriteEvtParams" {
            # "Write the event parameters to the event module"
            n291 = Variant To Data(type=T1 {"BusNumber"=0, "EvtPluginINIFilePath"=path "", "EvtParams"=[], "EvtConfig"={"UTC Time 0"=timestamp(0 s since 1904-01-01), "Nominal Frequency"=60, "Reporting Rate"=60, "Fsamp"=960, "PosSeq"=FALSE}, "Start Time"=0.0, "End Time"=0.0, "PmuImpairPluginINIFilePath"=path "", "PmuImpairParams "=[["960"], ["8.19"], ["164"]], "PmuImpairConfig"={"FilterType"="", "bPosSeq"=TRUE}, "NetImpPluginINIFilePath"=path "", "NetImpParams"=[], "FlagImpPluginINIFilePath"=path "", "FlagImpParams"=[], "EvtReportArray"=[], "EventSignalArray"=[], "ImpairReportArray"=[], "NetworkTime"=[], "PktLoss"=[], "FlagImpArray"=[], "OutputToFilePluginINIFilePath"=path "", "Output File Path"=path "", "clConfigOptions"={"TIME_BASE"=1000000, "STN"="Bus_1", "IDCODE"=0, "rdoPolRect"=enum."Rectangular", "rdoFloatInt"=enum."Float", "PHUNIT"=1000000, "rdoFreqDfreq"=enum."Float", "CHNAM"=["VA", "VB", "VC", "V+", "IA", "IB", "IC", "I+"], "chkCfg2Prefix"=TRUE}, "AppPluginINIFilePath"=path "", "AppConfig"=variant, "AppOutput"=variant} ("clBusData"), Variant=w750) -> (data=w749:T1, error out=w739:errorcluster)  [unwired: 1 in]
            n292 = Unbundle By Name(w741) -> ("EventModuleID"=w740:i32)
            n293 = Unbundle By Name(w749) -> ("EvtParams"=w738:string[][])
            n294 = call "2DstrTableTodblArray.vi"("strTable"=w738) -> ("dbl2DArray"=w748:dbl[][])  [unwired: 10 in]
            n295 = call "WriteEvtParamsRequest.vi"("error in (no error)"=w739, "EvtParams"=w748, "ModuleID"=w740) -> ("error out"=w743:errorcluster)  [unwired: 8 in]
            n296 = in-place {
              in-place-border: w738 -> [w752]
              n297 = in-place-cluster #11(w737) -> ()  [unwired: 1 out]
              n298 = in-place-cluster #11("EvtParams"=w752) -> (w736:T1)
            }
            n299 = call <userlib>:"AddError.vi"("Severity"="Abort" ("String"), "Priority"=u8 3, "ErrorArray"=w742, "error in (no error)"=w743) -> ("ErrorArray"=w744:errorcluster[], "error out"=w745:errorcluster)  [unwired: 6 in]
            n300 = call <vilib>:"Clear Errors.vi"("error in (no error)"=w745) -> ()  [unwired: 5 in, 2 out]
          }
          frame "ReadEvtParams" {
            n301 = call "ObtainBroadcastForRegistration.vi"() -> ("error out"=w759:errorcluster, "EventBroadcast"=w768:T16)  [unwired: 10 in]
            n302 = Unbundle By Name(w767) -> ("EventModuleID"=w755:i32)
            n303 = register-events(error in=w759, w768) -> (reference out=w756:refnum<event-registration>, error out=w758:errorcluster)  [unwired: 1 in]
            n304 = call "ReadEvtParamsRequest.vi"("error in (no error)"=w758, "ModuleID"=w755) -> ("error out"=w757:errorcluster)  [unwired: 9 in]
            n305 = case shown="No Error" w757 {
              selector: w757 -> [w773 w781]
              tunnel: [w776 w780] -> w760
              tunnel: [w773 w781] -> w753
              tunnel: w761 -> [w772 w780]
              tunnel: w756 -> [w771 _]
              tunnel: w755 -> [w770 _]
              tunnel: w754 -> [w769 _]
              frame No Error {
                n306 = Bundle By Name(cluster=T12 {"ModuleType"=enum."PMU", "ModuleID"=0, "UsrEvtRef"=variant, "ScriptCmd"=""} ("GetBdcstData"), "UsrEvtRef"=w771, "ModuleID"=w770, "ModuleType"=ModuleType."Event", "ScriptCmd"=w769) -> (w777:T12)
                n307 = call "Enqueue.vi"("Priority (f)"=TRUE, "ErrorArray"=w772, "Data"=w777, "Msg"="GetBroadcast") -> ("ErrorArray"=w776:errorcluster[])  [unwired: 7 in]
              }
              frame Error {
              }
            }
            n308 = call <userlib>:"AddError.vi"("Severity"="Abort" ("String"), "Priority"=u8 3, "ErrorArray"=w760, "error in (no error)"=w753) -> ("ErrorArray"=w763:errorcluster[], "error out"=w764:errorcluster)  [unwired: 6 in]
            n309 = call <vilib>:"Clear Errors.vi"("error in (no error)"=w764) -> ()  [unwired: 5 in, 2 out]
          }
          frame "WriteEvtConfig" {
            # "Write the event parameters to the event module"
            n310 = Variant To Data(type=T1 {"BusNumber"=0, "EvtPluginINIFilePath"=path "", "EvtParams"=[], "EvtConfig"={"UTC Time 0"=timestamp(0 s since 1904-01-01), "Nominal Frequency"=60, "Reporting Rate"=60, "Fsamp"=960, "PosSeq"=FALSE}, "Start Time"=0.0, "End Time"=0.0, "PmuImpairPluginINIFilePath"=path "", "PmuImpairParams "=[["960"], ["8.19"], ["164"]], "PmuImpairConfig"={"FilterType"="", "bPosSeq"=TRUE}, "NetImpPluginINIFilePath"=path "", "NetImpParams"=[], "FlagImpPluginINIFilePath"=path "", "FlagImpParams"=[], "EvtReportArray"=[], "EventSignalArray"=[], "ImpairReportArray"=[], "NetworkTime"=[], "PktLoss"=[], "FlagImpArray"=[], "OutputToFilePluginINIFilePath"=path "", "Output File Path"=path "", "clConfigOptions"={"TIME_BASE"=1000000, "STN"="Bus_1", "IDCODE"=0, "rdoPolRect"=enum."Rectangular", "rdoFloatInt"=enum."Float", "PHUNIT"=1000000, "rdoFreqDfreq"=enum."Float", "CHNAM"=["VA", "VB", "VC", "V+", "IA", "IB", "IC", "I+"], "chkCfg2Prefix"=TRUE}, "AppPluginINIFilePath"=path "", "AppConfig"=variant, "AppOutput"=variant} ("clBusData"), Variant=w803) -> (data=w785:T1, error out=w786:errorcluster)  [unwired: 1 in]
            n311 = Unbundle By Name(w805) -> ("EventModuleID"=w802:i32)
            n312 = Unbundle By Name(w785) -> ("EvtConfig.UTC Time 0"=w793:timestamp, "EvtConfig.Nominal Frequency"=w791:u16, "EvtConfig.Reporting Rate"=w789:u16, "EvtConfig.Fsamp"=w788:u32, "EvtConfig.PosSeq"=w782:bool)
            n313 = To Double Precision Float(number=w793) -> (double precision float=w792:dbl)
            n314 = To Double Precision Float(number=w791) -> (double precision float=w790:dbl)
            n315 = To Long Integer(number=w789) -> (32bit integer=w794:i32)
            n316 = Bundle By Name(cluster=T15 {"T0(UTC)"=0.0, "F0"=0.0, "Fs"=0, "FSamp"=0, "bPosSeq"=FALSE} ("clEvtConfig"), "T0(UTC)"=w792, "F0"=w790, "Fs"=w794, "FSamp"=w788, "bPosSeq"=w782) -> (w787:T15)
            n317 = call "WriteEvtConfigRequest.vi"("error in (no error)"=w786, "clEvtConfig"=w787, "ModuleID"=w802) -> ("error out"=w797:errorcluster)  [unwired: 8 in]
            n318 = in-place {
              n319 = in-place-cluster #12(w784) -> ()  [unwired: 1 out]
              n320 = in-place-cluster #13(w785) -> ("EvtConfig"=w806:T2)
              n321 = in-place-cluster #12("EvtConfig"=w806) -> (w783:T1)
              n322 = in-place-cluster #13("EvtConfig"=w806) -> ()  [unwired: 1 out]
            }
            n323 = call <userlib>:"AddError.vi"("Severity"="Abort" ("String"), "Priority"=u8 3, "ErrorArray"=w796, "error in (no error)"=w797) -> ("ErrorArray"=w798:errorcluster[], "error out"=w799:errorcluster)  [unwired: 6 in]
            n324 = call <vilib>:"Clear Errors.vi"("error in (no error)"=w799) -> ()  [unwired: 5 in, 2 out]
          }
          frame "ReadEvtConfig" {
            n325 = Unbundle By Name(w822) -> ("EventModuleID"=w810:i32)
            n326 = call "ObtainBroadcastForRegistration.vi"() -> ("error out"=w813:errorcluster, "EventBroadcast"=w821:T16)  [unwired: 10 in]
            n327 = register-events(error in=w813, w821) -> (reference out=w809:refnum<event-registration>, error out=w812:errorcluster)  [unwired: 1 in]
            n328 = call "ReadEvtConfigRequest.vi"("error in (no error)"=w812, "ModuleID"=w810) -> ("error out"=w811:errorcluster)  [unwired: 9 in]
            n329 = case shown="No Error" w811 {
              selector: w811 -> [w827 w835]
              tunnel: [w830 w834] -> w814
              tunnel: [w827 w835] -> w807
              tunnel: w815 -> [w826 w834]
              tunnel: w809 -> [w825 _]
              tunnel: w810 -> [w824 _]
              tunnel: w808 -> [w823 _]
              frame No Error {
                n330 = Bundle By Name(cluster=T12 {"ModuleType"=enum."PMU", "ModuleID"=0, "UsrEvtRef"=variant, "ScriptCmd"=""} ("GetBdcstData"), "UsrEvtRef"=w825, "ModuleID"=w824, "ModuleType"=ModuleType."Event", "ScriptCmd"=w823) -> (w831:T12)
                n331 = call "Enqueue.vi"("Priority (f)"=TRUE, "ErrorArray"=w826, "Data"=w831, "Msg"="GetBroadcast") -> ("ErrorArray"=w830:errorcluster[])  [unwired: 7 in]
              }
              frame Error {
              }
            }
            n332 = call <userlib>:"AddError.vi"("Severity"="Abort" ("String"), "Priority"=u8 3, "ErrorArray"=w814, "error in (no error)"=w807) -> ("ErrorArray"=w817:errorcluster[], "error out"=w818:errorcluster)  [unwired: 6 in]
            n333 = call <vilib>:"Clear Errors.vi"("error in (no error)"=w818) -> ()  [unwired: 5 in, 2 out]
          }
          frame "WriteEvtRptTimeArray" {
            # "The Event time array  for generating PMU reports, there is also an Event Signal Time Array which adds 2 filter delays to the beginning and end"
            n334 = Unbundle By Name(w853) -> ("EventModuleID"=w848:i32)
            n335 = Variant To Data(type=T1 {"BusNumber"=0, "EvtPluginINIFilePath"=path "", "EvtParams"=[], "EvtConfig"={"UTC Time 0"=timestamp(0 s since 1904-01-01), "Nominal Frequency"=60, "Reporting Rate"=60, "Fsamp"=960, "PosSeq"=FALSE}, "Start Time"=0.0, "End Time"=0.0, "PmuImpairPluginINIFilePath"=path "", "PmuImpairParams "=[["960"], ["8.19"], ["164"]], "PmuImpairConfig"={"FilterType"="", "bPosSeq"=TRUE}, "NetImpPluginINIFilePath"=path "", "NetImpParams"=[], "FlagImpPluginINIFilePath"=path "", "FlagImpParams"=[], "EvtReportArray"=[], "EventSignalArray"=[], "ImpairReportArray"=[], "NetworkTime"=[], "PktLoss"=[], "FlagImpArray"=[], "OutputToFilePluginINIFilePath"=path "", "Output File Path"=path "", "clConfigOptions"={"TIME_BASE"=1000000, "STN"="Bus_1", "IDCODE"=0, "rdoPolRect"=enum."Rectangular", "rdoFloatInt"=enum."Float", "PHUNIT"=1000000, "rdoFreqDfreq"=enum."Float", "CHNAM"=["VA", "VB", "VC", "V+", "IA", "IB", "IC", "I+"], "chkCfg2Prefix"=TRUE}, "AppPluginINIFilePath"=path "", "AppConfig"=variant, "AppOutput"=variant} ("clBusData"), Variant=w852) -> (data=w851:T1, error out=w847:errorcluster)  [unwired: 1 in]
            n336 = Unbundle By Name(w851) -> ("EvtConfig.Reporting Rate"=w849:u16, "End Time"=w837:dbl, "Start Time"=w836:dbl)
            n337 = Greater?(x=w837, y=w836) -> (0:w838:bool)
            n338 = case shown="True" w838 {
              tunnel: w849 -> [_ w876]
              tunnel: w848 -> [_ w875]
              tunnel: w847 -> [_ w873]
              tunnel: [w854 w872] -> w841
              tunnel: w837 -> [w856 w871]
              tunnel: w836 -> [w855 w870]
              tunnel: w840 -> [w857 w869]
              tunnel: [w857 w868] -> w839
              frame False {
                n339 = xnode "Error Ring"("parameter 0"=w855, "parameter 1"=w856) -> ("error out"=w854:errorcluster)
              }
              frame True {
                n340 = in-place {
                  in-place-border: w871 -> [w877]
                  in-place-border: w870 -> [w878]
                  n341 = in-place-cluster #14(w869) -> ()  [unwired: 2 out]
                  n342 = in-place-cluster #14("End Time"=w877, "Start Time"=w878) -> (w868:T1)
                }
                n343 = To Double Precision Float(number=w876) -> (double precision float=w867:dbl)
                n344 = Reciprocal(x=w867) -> (1/x=w866:dbl)
                n345 = call-poly <vilib>:"Ramp Pattern.vi"("start"=w870, "end"=w871, "delta"=w866) -> ("Ramp Pattern"=w874:dbl[])  [unwired: 6 in, 2 out]
                n346 = call "WriteTimeArrayRequest.vi"("error in (no error)"=w873, "TimeArray"=w874, "ModuleID"=w875) -> ("error out"=w872:errorcluster)  [unwired: 8 in]
              }
            }
            n347 = call <userlib>:"AddError.vi"("Severity"="Abort" ("String"), "Priority"=u8 3, "ErrorArray"=w842, "error in (no error)"=w841) -> ("ErrorArray"=w843:errorcluster[], "error out"=w844:errorcluster)  [unwired: 6 in]
            n348 = call <vilib>:"Clear Errors.vi"("error in (no error)"=w844) -> ()  [unwired: 5 in, 2 out]
          }
          frame "ReadEvtTime" {
            n349 = Unbundle By Name(w893) -> ("EventModuleID"=w880:i32)
            n350 = call "ObtainBroadcastForRegistration.vi"() -> ("error out"=w887:errorcluster, "EventBroadcast"=w894:T16)  [unwired: 10 in]
            n351 = register-events(error in=w887, w894) -> (reference out=w881:refnum<event-registration>, error out=w883:errorcluster)  [unwired: 1 in]
            n352 = call "ReadTimeArrayRequest.vi"("error in (no error)"=w883, "ModuleID"=w880) -> ("error out"=w882:errorcluster)  [unwired: 9 in]
            n353 = case shown="No Error" w882 {
              selector: w882 -> [w899 w907]
              tunnel: [w902 w906] -> w885
              tunnel: [w899 w907] -> w884
              tunnel: w886 -> [w898 w906]
              tunnel: w881 -> [w897 _]
              tunnel: w880 -> [w896 _]
              tunnel: w879 -> [w895 _]
              frame No Error {
                n354 = Bundle By Name(cluster=T12 {"ModuleType"=enum."PMU", "ModuleID"=0, "UsrEvtRef"=variant, "ScriptCmd"=""} ("GetBdcstData"), "UsrEvtRef"=w897, "ModuleID"=w896, "ModuleType"=ModuleType."Event", "ScriptCmd"=w895) -> (w903:T12)
                n355 = call "Enqueue.vi"("Priority (f)"=TRUE, "ErrorArray"=w898, "Data"=w903, "Msg"="GetBroadcast") -> ("ErrorArray"=w902:errorcluster[])  [unwired: 7 in]
              }
              frame Error {
              }
            }
            n356 = call <userlib>:"AddError.vi"("Severity"="Abort" ("String"), "Priority"=u8 3, "ErrorArray"=w885, "error in (no error)"=w884) -> ("ErrorArray"=w890:errorcluster[], "error out"=w889:errorcluster)  [unwired: 6 in]
            n357 = call <vilib>:"Clear Errors.vi"("error in (no error)"=w889) -> ()  [unwired: 5 in, 2 out]
          }
          frame "GetEvtReports" {
            n358 = call "ObtainBroadcastForRegistration.vi"() -> ("error out"=w919:errorcluster, "EventBroadcast"=w920:T16)  [unwired: 10 in]
            n359 = Unbundle By Name(w921) -> ("EventModuleID"=w910:i32)
            n360 = register-events(w920) -> (reference out=w911:refnum<event-registration>)  [unwired: 2 in, 1 out]
            n361 = call "GetEvtReportsRequest.vi"("error in (no error)"=w919, "ModuleID"=w910) -> ("error out"=w912:errorcluster)  [unwired: 9 in]
            n362 = case shown="No Error" w912 {
              selector: w912 -> [w926 w934]
              tunnel: [w929 w933] -> w913
              tunnel: [w926 w934] -> w908
              tunnel: w914 -> [w925 w933]
              tunnel: w911 -> [w924 _]
              tunnel: w910 -> [w923 _]
              tunnel: w909 -> [w922 _]
              frame No Error {
                n363 = Bundle By Name(cluster=T12 {"ModuleType"=enum."PMU", "ModuleID"=0, "UsrEvtRef"=variant, "ScriptCmd"=""} ("GetBdcstData"), "UsrEvtRef"=w924, "ModuleID"=w923, "ModuleType"=ModuleType."Event", "ScriptCmd"=w922) -> (w930:T12)
                n364 = call "Enqueue.vi"("Priority (f)"=TRUE, "ErrorArray"=w925, "Data"=w930, "Msg"="GetBroadcast") -> ("ErrorArray"=w929:errorcluster[])  [unwired: 7 in]
              }
              frame Error {
              }
            }
            n365 = call <userlib>:"AddError.vi"("Severity"="Abort" ("String"), "Priority"=u8 3, "ErrorArray"=w913, "error in (no error)"=w908) -> ("ErrorArray"=w916:errorcluster[])  [unwired: 6 in, 1 out]
          }
          frame "GetEvtSignal" {
            # "Note that these are being pushed into the front of the queue in the reverse order in which they will be executed"
            n366 = call "Enqueue.vi"("Priority (f)"=TRUE, "ErrorArray"=w953, "Msg"="TransferEvtTimeArrayToEvt") -> ("ErrorArray"=w952:errorcluster[])  [unwired: 8 in]
            n367 = call "Enqueue.vi"("Priority (f)"=TRUE, "ErrorArray"=w952, "Msg"="AquireEvtSignal") -> ("ErrorArray"=w948:errorcluster[])  [unwired: 8 in]
            n368 = call "Enqueue.vi"("Priority (f)"=TRUE, "ErrorArray"=w948, "Msg"="WriteEvtSigTimeArray") -> ("ErrorArray"=w944:errorcluster[])  [unwired: 8 in]
            n369 = call "Enqueue.vi"("Priority (f)"=TRUE, "ErrorArray"=w944, "Msg"="ReadEvtTime") -> ("ErrorArray"=w941:errorcluster[])  [unwired: 8 in]
            n370 = call "Enqueue.vi"("Priority (f)"=TRUE, "ErrorArray"=w941, "Msg"="ReadPmuImpairParams") -> ("ErrorArray"=w938:errorcluster[])  [unwired: 8 in]
            n371 = call "Enqueue.vi"("Priority (f)"=TRUE, "ErrorArray"=w938, "Msg"="ReadEvtConfig") -> ("ErrorArray"=w936:errorcluster[])  [unwired: 8 in]
          }
          frame "WriteEvtSigTimeArray" {
            # "Assumes all this has been read back from the event and PMU Impair modules\nSo before calling this, be sure to call the following:\nReadEvtConfig, ReadEvtTime, ReadPmuImpairParams.\n\nAfter getting the event signal, be sure to call RefreshEvtSTimeArray to replace the signal time array with the event reports time array"
            # "The Event time array  for generating Event signal and extends the time array by 2 filter periods at each end, There is also an Event Report Time Array."
            n372 = Unbundle By Name(w979) -> ("EventModuleID"=w975:i32)
            n373 = Unbundle By Name(w956) -> ("EvtConfig.Reporting Rate"=w978:u16, "End Time"=w962:dbl, "Start Time"=w964:dbl, "PmuImpairParams"=w967:string[][], "EvtConfig.Fsamp"=w958:u32)
            n374 = Index Array(array=w967, index (row)=1, index (col)=0 ("disabled index (col)")) -> (element=w960:string)
            n375 = Decimal String To Number(string=w960) -> (number=w959:i32)  [unwired: 2 in, 1 out]
            n376 = Compound Arithmetic op=MULTIPLY(w959, invert w958, 2.0 ("value")) -> (w957:dbl)
            n377 = Add(x=w962, y=w957) -> (x+y=w961:dbl)
            n378 = Subtract(x=w964, y=w957) -> (x-y=w963:dbl)
            n379 = To Double Precision Float(number=w978) -> (double precision float=w977:dbl)
            n380 = Reciprocal(x=w977) -> (1/x=w976:dbl)
            n381 = call-poly <vilib>:"Ramp Pattern.vi"("start"=w963, "end"=w961, "delta"=w976) -> ("Ramp Pattern"=w974:dbl[])  [unwired: 6 in, 2 out]
            n382 = call "WriteTimeArrayRequest.vi"("TimeArray"=w974, "ModuleID"=w975) -> ("error out"=w968:errorcluster)  [unwired: 9 in]
            n383 = call <userlib>:"AddError.vi"("Severity"="Abort" ("String"), "Priority"=u8 3, "ErrorArray"=w969, "error in (no error)"=w968) -> ("ErrorArray"=w970:errorcluster[], "error out"=w971:errorcluster)  [unwired: 6 in]
            n384 = call <vilib>:"Clear Errors.vi"("error in (no error)"=w971) -> ()  [unwired: 5 in, 2 out]
          }
          frame "TransferEvtTimeArrayToEvt" {
            n385 = Unbundle By Name(w986) -> ("EvtConfig.Reporting Rate"=w992:u16, "End Time"=w988:dbl, "Start Time"=w987:dbl)
            n386 = To Double Precision Float(number=w992) -> (double precision float=w991:dbl)
            n387 = Reciprocal(x=w991) -> (1/x=w990:dbl)
            n388 = call-poly <vilib>:"Ramp Pattern.vi"("start"=w987, "end"=w988, "delta"=w990) -> ("Ramp Pattern"=w989:dbl[])  [unwired: 6 in, 2 out]
            n389 = call "WriteTimeArrayRequest.vi"("TimeArray"=w989) -> ("error out"=w981:errorcluster)  [unwired: 10 in]
            n390 = call <userlib>:"AddError.vi"("Severity"="Abort" ("String"), "Priority"=u8 3, "ErrorArray"=w980, "error in (no error)"=w981) -> ("ErrorArray"=w982:errorcluster[], "error out"=w983:errorcluster)  [unwired: 6 in]
            n391 = call <vilib>:"Clear Errors.vi"("error in (no error)"=w983) -> ()  [unwired: 5 in, 2 out]
          }
          frame "AquireEvtSignal" {
            n392 = Unbundle By Name(w1006) -> ("EventModuleID"=w995:i32)
            n393 = call "ObtainBroadcastForRegistration.vi"() -> ("error out"=w998:errorcluster, "EventBroadcast"=w1007:T16)  [unwired: 10 in]
            n394 = register-events(error in=w998, w1007) -> (reference out=w996:refnum<event-registration>, error out=w997:errorcluster)  [unwired: 1 in]
            n395 = call "GetEvtSignalRequest.vi"("error in (no error)"=w997, "ModuleID"=w995) -> ("error out"=w999:errorcluster)  [unwired: 9 in]
            n396 = case shown="No Error" w999 {
              selector: w999 -> [w1012 w1020]
              tunnel: [w1015 w1019] -> w1000
              tunnel: [w1012 w1020] -> w993
              tunnel: w1001 -> [w1011 w1019]
              tunnel: w995 -> [w1010 _]
              tunnel: w994 -> [w1009 _]
              tunnel: w996 -> [w1008 _]
              frame No Error {
                n397 = Bundle By Name(cluster=T12 {"ModuleType"=enum."PMU", "ModuleID"=0, "UsrEvtRef"=variant, "ScriptCmd"=""} ("GetBdcstData"), "UsrEvtRef"=w1008, "ModuleID"=w1010, "ModuleType"=ModuleType."Event", "ScriptCmd"=w1009) -> (w1016:T12)
                n398 = call "Enqueue.vi"("Priority (f)"=TRUE, "ErrorArray"=w1011, "Data"=w1016, "Msg"="GetBroadcast") -> ("ErrorArray"=w1015:errorcluster[])  [unwired: 7 in]
              }
              frame Error {
              }
            }
            n399 = call <userlib>:"AddError.vi"("Severity"="Abort" ("String"), "Priority"=u8 3, "ErrorArray"=w1000, "error in (no error)"=w993) -> ("ErrorArray"=w1003:errorcluster[])  [unwired: 6 in, 1 out]
          }
          frame "WritePmuImpairBusNumber" {
            # "Write the event parameters to the event module"
            n400 = Unbundle By Name(w1028) -> ("PmuImpairModuleID"=w1027:i32)
            n401 = Variant To Data(type=T1 {"BusNumber"=0, "EvtPluginINIFilePath"=path "", "EvtParams"=[], "EvtConfig"={"UTC Time 0"=timestamp(0 s since 1904-01-01), "Nominal Frequency"=60, "Reporting Rate"=60, "Fsamp"=960, "PosSeq"=FALSE}, "Start Time"=0.0, "End Time"=0.0, "PmuImpairPluginINIFilePath"=path "", "PmuImpairParams "=[["960"], ["8.19"], ["164"]], "PmuImpairConfig"={"FilterType"="", "bPosSeq"=TRUE}, "NetImpPluginINIFilePath"=path "", "NetImpParams"=[], "FlagImpPluginINIFilePath"=path "", "FlagImpParams"=[], "EvtReportArray"=[], "EventSignalArray"=[], "ImpairReportArray"=[], "NetworkTime"=[], "PktLoss"=[], "FlagImpArray"=[], "OutputToFilePluginINIFilePath"=path "", "Output File Path"=path "", "clConfigOptions"={"TIME_BASE"=1000000, "STN"="Bus_1", "IDCODE"=0, "rdoPolRect"=enum."Rectangular", "rdoFloatInt"=enum."Float", "PHUNIT"=1000000, "rdoFreqDfreq"=enum."Float", "CHNAM"=["VA", "VB", "VC", "V+", "IA", "IB", "IC", "I+"], "chkCfg2Prefix"=TRUE}, "AppPluginINIFilePath"=path "", "AppConfig"=variant, "AppOutput"=variant} ("clBusData"), Variant=w1024) -> (data=w1025:T1)  [unwired: 1 in, 1 out]
            n402 = Unbundle By Name(w1025) -> ("BusNumber"=w1022:u8)
            n403 = call "WriteBusNumberRequest.vi"("BusNumber"=w1022, "ModuleID"=w1027) -> ("error out"=w1030:errorcluster)  [unwired: 9 in]
            n404 = in-place {
              in-place-border: w1022 -> [w1035]
              n405 = in-place-cluster #15(w1023) -> ()  [unwired: 1 out]
              n406 = in-place-cluster #15("BusNumber"=w1035) -> (w1021:T1)
            }
            n407 = call <userlib>:"AddError.vi"("Severity"="Abort" ("String"), "Priority"=u8 3, "ErrorArray"=w1029, "error in (no error)"=w1030) -> ("ErrorArray"=w1031:errorcluster[], "error out"=w1032:errorcluster)  [unwired: 6 in]
            n408 = call <vilib>:"Clear Errors.vi"("error in (no error)"=w1032) -> ()  [unwired: 5 in, 2 out]
          }
          frame "ReadPmuImpairBusNumber" {
            n409 = Unbundle By Name(w1050) -> ("PmuImpairModuleID"=w1049:i32)
            n410 = call "ObtainBroadcastForRegistration.vi"() -> ("error out"=w1036:errorcluster, "ImpairBroadcast"=w1037:T17)  [unwired: 10 in]
            n411 = register-events(error in=w1036, w1037) -> (reference out=w1040:refnum<event-registration>, error out=w1039:errorcluster)  [unwired: 1 in]
            n412 = call "ReadBusNumberRequest.vi"("error in (no error)"=w1039, "ModuleID"=w1049) -> ("error out"=w1038:errorcluster)  [unwired: 9 in]
            n413 = case shown="No Error" w1038 {
              selector: w1038 -> [w1055 w1063]
              tunnel: [w1058 w1062] -> w1041
              tunnel: [w1055 w1063] -> w1043
              tunnel: w1042 -> [w1054 w1062]
              tunnel: w1049 -> [w1053 _]
              tunnel: w1044 -> [w1052 _]
              tunnel: w1040 -> [w1051 _]
              frame No Error {
                n414 = Bundle By Name(cluster=T12 {"ModuleType"=enum."PMU", "ModuleID"=0, "UsrEvtRef"=variant, "ScriptCmd"=""} ("GetBdcstData"), "UsrEvtRef"=w1051, "ModuleID"=w1053, "ModuleType"=ModuleType."PMU", "ScriptCmd"=w1052) -> (w1059:T12)
                n415 = call "Enqueue.vi"("Priority (f)"=TRUE, "ErrorArray"=w1054, "Data"=w1059, "Msg"="GetBroadcast") -> ("ErrorArray"=w1058:errorcluster[])  [unwired: 7 in]
              }
              frame Error {
              }
            }
            n416 = call <userlib>:"AddError.vi"("Severity"="Abort" ("String"), "Priority"=u8 3, "ErrorArray"=w1041, "error in (no error)"=w1043) -> ("ErrorArray"=w1045:errorcluster[])  [unwired: 6 in, 1 out]
          }
          frame "WritePMUImpairParams" {
            # "Write the event parameters to the event module"
            n417 = Variant To Data(type=T1 {"BusNumber"=0, "EvtPluginINIFilePath"=path "", "EvtParams"=[], "EvtConfig"={"UTC Time 0"=timestamp(0 s since 1904-01-01), "Nominal Frequency"=60, "Reporting Rate"=60, "Fsamp"=960, "PosSeq"=FALSE}, "Start Time"=0.0, "End Time"=0.0, "PmuImpairPluginINIFilePath"=path "", "PmuImpairParams "=[["960"], ["8.19"], ["164"]], "PmuImpairConfig"={"FilterType"="", "bPosSeq"=TRUE}, "NetImpPluginINIFilePath"=path "", "NetImpParams"=[], "FlagImpPluginINIFilePath"=path "", "FlagImpParams"=[], "EvtReportArray"=[], "EventSignalArray"=[], "ImpairReportArray"=[], "NetworkTime"=[], "PktLoss"=[], "FlagImpArray"=[], "OutputToFilePluginINIFilePath"=path "", "Output File Path"=path "", "clConfigOptions"={"TIME_BASE"=1000000, "STN"="Bus_1", "IDCODE"=0, "rdoPolRect"=enum."Rectangular", "rdoFloatInt"=enum."Float", "PHUNIT"=1000000, "rdoFreqDfreq"=enum."Float", "CHNAM"=["VA", "VB", "VC", "V+", "IA", "IB", "IC", "I+"], "chkCfg2Prefix"=TRUE}, "AppPluginINIFilePath"=path "", "AppConfig"=variant, "AppOutput"=variant} ("clBusData"), Variant=w1077) -> (data=w1076:T1, error out=w1067:errorcluster)  [unwired: 1 in]
            n418 = Unbundle By Name(w1079) -> ("PmuImpairModuleID"=w1075:i32)
            n419 = Unbundle By Name(w1076) -> ("PmuImpairParams"=w1066:string[][])
            n420 = call "2DstrTableTodblArray.vi"("strTable"=w1066) -> ("dbl2DArray"=w1068:dbl[][])  [unwired: 10 in]
            n421 = call "WriteImpairParamsRequest.vi"("error in (no error)"=w1067, "dblImpairParams"=w1068, "ModuleID"=w1075) -> ("error out"=w1070:errorcluster)  [unwired: 8 in]
            n422 = in-place {
              in-place-border: w1066 -> [w1080]
              n423 = in-place-cluster #16(w1065) -> ()  [unwired: 1 out]
              n424 = in-place-cluster #16("PmuImpairParams"=w1080) -> (w1064:T1)
            }
            n425 = call <userlib>:"AddError.vi"("Severity"="Abort" ("String"), "Priority"=u8 3, "ErrorArray"=w1069, "error in (no error)"=w1070) -> ("ErrorArray"=w1071:errorcluster[], "error out"=w1072:errorcluster)  [unwired: 6 in]
            n426 = call <vilib>:"Clear Errors.vi"("error in (no error)"=w1072) -> ()  [unwired: 5 in, 2 out]
          }
          frame "ReadPMUImpairParams" {
            n427 = Unbundle By Name(w1095) -> ("PmuImpairModuleID"=w1094:i32)
            n428 = call "ObtainBroadcastForRegistration.vi"() -> ("error out"=w1081:errorcluster, "ImpairBroadcast"=w1082:T17)  [unwired: 10 in]
            n429 = register-events(error in=w1081, w1082) -> (reference out=w1085:refnum<event-registration>, error out=w1084:errorcluster)  [unwired: 1 in]
            n430 = call "ReadImpairParamsRequest.vi"("error in (no error)"=w1084, "ModuleID"=w1094) -> ("error out"=w1083:errorcluster)  [unwired: 9 in]
            n431 = case shown="No Error" w1083 {
              selector: w1083 -> [w1100 w1108]
              tunnel: [w1103 w1107] -> w1086
              tunnel: [w1100 w1108] -> w1088
              tunnel: w1087 -> [w1099 w1107]
              tunnel: w1094 -> [w1098 _]
              tunnel: w1089 -> [w1097 _]
              tunnel: w1085 -> [w1096 _]
              frame No Error {
                n432 = Bundle By Name(cluster=T12 {"ModuleType"=enum."PMU", "ModuleID"=0, "UsrEvtRef"=variant, "ScriptCmd"=""} ("GetBdcstData"), "UsrEvtRef"=w1096, "ModuleID"=w1098, "ModuleType"=ModuleType."PMU", "ScriptCmd"=w1097) -> (w1104:T12)
                n433 = call "Enqueue.vi"("Priority (f)"=TRUE, "ErrorArray"=w1099, "Data"=w1104, "Msg"="GetBroadcast") -> ("ErrorArray"=w1103:errorcluster[])  [unwired: 7 in]
              }
              frame Error {
              }
            }
            n434 = call <userlib>:"AddError.vi"("Severity"="Abort" ("String"), "Priority"=u8 3, "ErrorArray"=w1086, "error in (no error)"=w1088) -> ("ErrorArray"=w1090:errorcluster[])  [unwired: 6 in, 1 out]
          }
          frame "WritePmuImpairEvtParams" {
            # "Write the event parameters to the event module"
            n435 = Variant To Data(type=T1 {"BusNumber"=0, "EvtPluginINIFilePath"=path "", "EvtParams"=[], "EvtConfig"={"UTC Time 0"=timestamp(0 s since 1904-01-01), "Nominal Frequency"=60, "Reporting Rate"=60, "Fsamp"=960, "PosSeq"=FALSE}, "Start Time"=0.0, "End Time"=0.0, "PmuImpairPluginINIFilePath"=path "", "PmuImpairParams "=[["960"], ["8.19"], ["164"]], "PmuImpairConfig"={"FilterType"="", "bPosSeq"=TRUE}, "NetImpPluginINIFilePath"=path "", "NetImpParams"=[], "FlagImpPluginINIFilePath"=path "", "FlagImpParams"=[], "EvtReportArray"=[], "EventSignalArray"=[], "ImpairReportArray"=[], "NetworkTime"=[], "PktLoss"=[], "FlagImpArray"=[], "OutputToFilePluginINIFilePath"=path "", "Output File Path"=path "", "clConfigOptions"={"TIME_BASE"=1000000, "STN"="Bus_1", "IDCODE"=0, "rdoPolRect"=enum."Rectangular", "rdoFloatInt"=enum."Float", "PHUNIT"=1000000, "rdoFreqDfreq"=enum."Float", "CHNAM"=["VA", "VB", "VC", "V+", "IA", "IB", "IC", "I+"], "chkCfg2Prefix"=TRUE}, "AppPluginINIFilePath"=path "", "AppConfig"=variant, "AppOutput"=variant} ("clBusData"), Variant=w1122) -> (data=w1110:T1, error out=w1113:errorcluster)  [unwired: 1 in]
            n436 = Unbundle By Name(w1124) -> ("PmuImpairModuleID"=w1121:i32)
            n437 = Unbundle By Name(w1110) -> ("EvtParams"=w1109:string[][])
            n438 = call "2DstrTableTodblArray.vi"("strTable"=w1109) -> ("dbl2DArray"=w1114:dbl[][])  [unwired: 10 in]
            n439 = call "WriteEvtParamsRequest.vi"("error in (no error)"=w1113, "EvtParams"=w1114, "ModuleID"=w1121) -> ("error out"=w1116:errorcluster)  [unwired: 8 in]
            n440 = in-place {
              in-place-border: w1109 -> [w1125]
              n441 = in-place-cluster #17(w1112) -> ()  [unwired: 1 out]
              n442 = in-place-cluster #17("EvtParams"=w1125) -> (w1111:T1)
            }
            n443 = call <userlib>:"AddError.vi"("Severity"="Abort" ("String"), "Priority"=u8 3, "ErrorArray"=w1115, "error in (no error)"=w1116) -> ("ErrorArray"=w1117:errorcluster[], "error out"=w1118:errorcluster)  [unwired: 6 in]
            n444 = call <vilib>:"Clear Errors.vi"("error in (no error)"=w1118) -> ()  [unwired: 5 in, 2 out]
          }
          frame "WritePmuImpairConfig" {
            n445 = Unbundle By Name(w1136) -> ("PmuImpairModuleID"=w1131:i32)
            n446 = Variant To Data(type=T1 {"BusNumber"=0, "EvtPluginINIFilePath"=path "", "EvtParams"=[], "EvtConfig"={"UTC Time 0"=timestamp(0 s since 1904-01-01), "Nominal Frequency"=60, "Reporting Rate"=60, "Fsamp"=960, "PosSeq"=FALSE}, "Start Time"=0.0, "End Time"=0.0, "PmuImpairPluginINIFilePath"=path "", "PmuImpairParams "=[["960"], ["8.19"], ["164"]], "PmuImpairConfig"={"FilterType"="", "bPosSeq"=TRUE}, "NetImpPluginINIFilePath"=path "", "NetImpParams"=[], "FlagImpPluginINIFilePath"=path "", "FlagImpParams"=[], "EvtReportArray"=[], "EventSignalArray"=[], "ImpairReportArray"=[], "NetworkTime"=[], "PktLoss"=[], "FlagImpArray"=[], "OutputToFilePluginINIFilePath"=path "", "Output File Path"=path "", "clConfigOptions"={"TIME_BASE"=1000000, "STN"="Bus_1", "IDCODE"=0, "rdoPolRect"=enum."Rectangular", "rdoFloatInt"=enum."Float", "PHUNIT"=1000000, "rdoFreqDfreq"=enum."Float", "CHNAM"=["VA", "VB", "VC", "V+", "IA", "IB", "IC", "I+"], "chkCfg2Prefix"=TRUE}, "AppPluginINIFilePath"=path "", "AppConfig"=variant, "AppOutput"=variant} ("clBusData"), Variant=w1134) -> (data=w1133:T1, error out=w1132:errorcluster)  [unwired: 1 in]
            n447 = Unbundle By Name(w1133) -> ("PmuImpairConfig"=w1127:T3)
            n448 = call "WriteImpairConfigRequest.vi"("error in (no error)"=w1132, "clImpairConfig"=w1127, "ModuleID"=w1131) -> ("error out"=w1130:errorcluster)  [unwired: 8 in]
            n449 = in-place {
              in-place-border: w1127 -> [w1141]
              n450 = in-place-cluster #18(w1128) -> ()  [unwired: 1 out]
              n451 = in-place-cluster #18("PmuImpairConfig"=w1141) -> (w1126:T1)
            }
            n452 = call <userlib>:"AddError.vi"("Severity"="Abort" ("String"), "Priority"=u8 3, "ErrorArray"=w1129, "error in (no error)"=w1130) -> ("ErrorArray"=w1137:errorcluster[], "error out"=w1138:errorcluster)  [unwired: 6 in]
            n453 = call <vilib>:"Clear Errors.vi"("error in (no error)"=w1138) -> ()  [unwired: 5 in, 2 out]
          }
          frame "ReadPmuImpairConfig" {
            n454 = Unbundle By Name(w1153) -> ("PmuImpairModuleID"=w1152:i32)
            n455 = disable-structure shown="Enabled" {
              disable-tunnel: w1152 -> [w1166 w1188]
              disable-tunnel: w1151 -> [w1160 w1186]
              disable-tunnel: [w1158 w1186] -> w1150
              disable-tunnel: w1145 -> [w1157 w1187]
              disable-tunnel: [w1154 w1189] -> w1144
              disable-tunnel: w1143 -> [_ w1191]
              disable-tunnel: [_ w1190] -> w1142
              frame Disabled {
                n456 = call "ObtainBroadcastForRegistration.vi"() -> ("error out"=w1161:errorcluster, "ImpairBroadcast"=w1163:T17)  [unwired: 10 in]
                n457 = register-events(w1163) -> (reference out=w1162:refnum<event-registration>)  [unwired: 2 in, 1 out]
                n458 = call "ReadImpairConfigRequest.vi"("error in (no error)"=w1161, "ModuleID"=w1166) -> ("error out"=w1164:errorcluster)  [unwired: 9 in]
                n459 = event shown="[0] <ImpairBroadcast.ImpairConfig>: User Event" {
                  selector: w1162 -> [_ _ _]
                  dyn-events: [_ _ _] -> w1156
                  timeout: 5000 -> [_ _ _]
                  tunnel: w1164 -> [w1171 _ _]
                  tunnel: [w1170 w1174 w1178] -> w1155
                  tunnel: [w1168 _ _] -> w1159
                  tunnel: w1157 -> [_ _ w1177]
                  event User Event {
                    n460 = event-data() -> ("Data"=w1172:variant)  [unwired: 1 in]
                    n461 = Variant To Data(error in=w1171, type=T3 {"FilterType"="", "bPosSeq"=TRUE} ("clImpairConfig"), Variant=w1172) -> (data=w1168:T3, error out=w1170:errorcluster)
                  }
                  event User Event {
                    n462 = event-data() -> ("Data"=w1173:variant)  [unwired: 1 in]
                    n463 = Variant To Data(type=T14 {"error"={"status"=FALSE, "code"=0, "source"=""}, "AdditionalInfo"=""} ("Cluster"), Variant=w1173) -> (data=w1175:T14)  [unwired: 1 in, 1 out]
                    n464 = Unbundle By Name(w1175) -> ("error"=w1174:errorcluster)
                  }
                  event Timeout {
                    n465 = event-data() -> ()  [unwired: 1 in, 3 out]
                    n466 = xnode "Error Ring"("parameter 0"=w1177) -> ("error out"=w1178:errorcluster)
                  }
                }
                n467 = Unregister For Events(event registration refnum=w1156, error in=w1155) -> (error out=w1154:errorcluster)
                n468 = in-place {
                  in-place-border: w1159 -> [w1167]
                  n469 = in-place-cluster #19(w1160) -> ()  [unwired: 1 out]
                  n470 = in-place-cluster #19("PmuImpairConfig"=w1167) -> (w1158:T1)
                }
              }
              frame Enabled {
                n471 = call "ObtainBroadcastForRegistration.vi"() -> ("error out"=w1195:errorcluster, "ImpairBroadcast"=w1194:T17)  [unwired: 10 in]
                n472 = register-events(error in=w1195, w1194) -> (reference out=w1196:refnum<event-registration>, error out=w1193:errorcluster)  [unwired: 1 in]
                n473 = call "ReadImpairConfigRequest.vi"("error in (no error)"=w1193, "ModuleID"=w1188) -> ("error out"=w1192:errorcluster)  [unwired: 9 in]
                n474 = case shown="No Error" w1192 {
                  selector: w1192 -> [w1201 w1209]
                  tunnel: [w1204 w1208] -> w1190
                  tunnel: [w1201 w1209] -> w1189
                  tunnel: w1191 -> [w1200 w1208]
                  tunnel: w1188 -> [w1199 _]
                  tunnel: w1187 -> [w1198 _]
                  tunnel: w1196 -> [w1197 _]
                  frame No Error {
                    n475 = Bundle By Name(cluster=T12 {"ModuleType"=enum."PMU", "ModuleID"=0, "UsrEvtRef"=variant, "ScriptCmd"=""} ("GetBdcstData"), "UsrEvtRef"=w1197, "ModuleID"=w1199, "ModuleType"=ModuleType."PMU", "ScriptCmd"=w1198) -> (w1205:T12)
                    n476 = call "Enqueue.vi"("Priority (f)"=TRUE, "ErrorArray"=w1200, "Data"=w1205, "Msg"="GetBroadcast") -> ("ErrorArray"=w1204:errorcluster[])  [unwired: 7 in]
                  }
                  frame Error {
                  }
                }
              }
            }
            n477 = call <userlib>:"AddError.vi"("Severity"="Abort" ("String"), "Priority"=u8 3, "ErrorArray"=w1142, "error in (no error)"=w1144) -> ("ErrorArray"=w1146:errorcluster[], "error out"=w1147:errorcluster)  [unwired: 6 in]
            n478 = call <vilib>:"Clear Errors.vi"("error in (no error)"=w1147) -> ()  [unwired: 5 in, 2 out]
          }
          frame "WritePmuImpairEvtConfig" {
            n479 = Unbundle By Name(w1228) -> ("PmuImpairModuleID"=w1225:i32)
            n480 = Variant To Data(type=T1 {"BusNumber"=0, "EvtPluginINIFilePath"=path "", "EvtParams"=[], "EvtConfig"={"UTC Time 0"=timestamp(0 s since 1904-01-01), "Nominal Frequency"=60, "Reporting Rate"=60, "Fsamp"=960, "PosSeq"=FALSE}, "Start Time"=0.0, "End Time"=0.0, "PmuImpairPluginINIFilePath"=path "", "PmuImpairParams "=[["960"], ["8.19"], ["164"]], "PmuImpairConfig"={"FilterType"="", "bPosSeq"=TRUE}, "NetImpPluginINIFilePath"=path "", "NetImpParams"=[], "FlagImpPluginINIFilePath"=path "", "FlagImpParams"=[], "EvtReportArray"=[], "EventSignalArray"=[], "ImpairReportArray"=[], "NetworkTime"=[], "PktLoss"=[], "FlagImpArray"=[], "OutputToFilePluginINIFilePath"=path "", "Output File Path"=path "", "clConfigOptions"={"TIME_BASE"=1000000, "STN"="Bus_1", "IDCODE"=0, "rdoPolRect"=enum."Rectangular", "rdoFloatInt"=enum."Float", "PHUNIT"=1000000, "rdoFreqDfreq"=enum."Float", "CHNAM"=["VA", "VB", "VC", "V+", "IA", "IB", "IC", "I+"], "chkCfg2Prefix"=TRUE}, "AppPluginINIFilePath"=path "", "AppConfig"=variant, "AppOutput"=variant} ("clBusData"), Variant=w1226) -> (data=w1212:T1, error out=w1213:errorcluster)  [unwired: 1 in]
            n481 = Unbundle By Name(w1212) -> ("EvtConfig.UTC Time 0"=w1220:timestamp, "EvtConfig.Nominal Frequency"=w1218:u16, "EvtConfig.Reporting Rate"=w1216:u16, "EvtConfig.Fsamp"=w1215:u32, "EvtConfig.PosSeq"=w1210:bool)
            n482 = To Double Precision Float(number=w1220) -> (double precision float=w1219:dbl)
            n483 = To Double Precision Float(number=w1218) -> (double precision float=w1217:dbl)
            n484 = To Long Integer(number=w1216) -> (32bit integer=w1221:i32)
            n485 = Bundle By Name(cluster=T15 {"T0(UTC)"=0.0, "F0"=0.0, "Fs"=0, "FSamp"=0, "bPosSeq"=FALSE} ("clEvtConfig"), "T0(UTC)"=w1219, "F0"=w1217, "Fs"=w1221, "FSamp"=w1215, "bPosSeq"=w1210) -> (w1214:T15)
            n486 = call "WriteEvtConfigRequest.vi"("error in (no error)"=w1213, "EvtConfig"=w1214, "ModuleID"=w1225) -> ("error out"=w1224:errorcluster)  [unwired: 8 in]
            n487 = call <userlib>:"AddError.vi"("Severity"="Abort" ("String"), "Priority"=u8 3, "ErrorArray"=w1223, "error in (no error)"=w1224) -> ("ErrorArray"=w1229:errorcluster[], "error out"=w1230:errorcluster)  [unwired: 6 in]
            n488 = call <vilib>:"Clear Errors.vi"("error in (no error)"=w1230) -> ()  [unwired: 5 in, 2 out]
          }
          frame "TransferEvtReportsToPmuImpair" {
            n489 = Unbundle By Name(w1241) -> ("PmuImpairModuleID"=w1239:i32)
            n490 = Unbundle By Name(w1242) -> ("EvtReportArray"=w1240:T4)
            n491 = call "WriteEvtReportsRequest.vi"("EvtReportArray"=w1240, "ModuleID"=w1239) -> ("error out"=w1234:errorcluster)  [unwired: 9 in]
            n492 = call <userlib>:"AddError.vi"("Severity"="Abort" ("String"), "Priority"=u8 3, "ErrorArray"=w1233, "error in (no error)"=w1234) -> ("ErrorArray"=w1235:errorcluster[], "error out"=w1236:errorcluster)  [unwired: 6 in]
            n493 = call <vilib>:"Clear Errors.vi"("error in (no error)"=w1236) -> ()  [unwired: 5 in, 2 out]
          }
          frame "TransferEvtReportsToOutputToFile" {
            n494 = Unbundle By Name(w1251) -> ("OutputToFileModuleID"=w1249:i32)
            n495 = Unbundle By Name(w1252) -> ("EvtReportArray"=w1250:T4)
            n496 = call "WriteEvtRptArrayRequest.vi"("EvtRptArray"=w1250, "ModuleID"=w1249) -> ("error out"=w1244:errorcluster)  [unwired: 9 in]
            n497 = call <userlib>:"AddError.vi"("Severity"="Abort" ("String"), "Priority"=u8 3, "ErrorArray"=w1243, "error in (no error)"=w1244) -> ("ErrorArray"=w1245:errorcluster[], "error out"=w1246:errorcluster)  [unwired: 6 in]
            n498 = call <vilib>:"Clear Errors.vi"("error in (no error)"=w1246) -> ()  [unwired: 5 in, 2 out]
          }
          frame "TransferPMUImpairReportsToOutputToFile" {
            n499 = Unbundle By Name(w1261) -> ("OutputToFileModuleID"=w1259:i32)
            n500 = Unbundle By Name(w1262) -> ("ImpairReportArray"=w1260:T4)
            n501 = call "WritePMUImpairRptArrayRequest.vi"("PmuImpairRptArray"=w1260, "ModuleID"=w1259) -> ("error out"=w1254:errorcluster)  [unwired: 9 in]
            n502 = call <userlib>:"AddError.vi"("Severity"="Abort" ("String"), "Priority"=u8 3, "ErrorArray"=w1253, "error in (no error)"=w1254) -> ("ErrorArray"=w1255:errorcluster[], "error out"=w1256:errorcluster)  [unwired: 6 in]
            n503 = call <vilib>:"Clear Errors.vi"("error in (no error)"=w1256) -> ()  [unwired: 5 in, 2 out]
          }
          frame "TransferPMUImpairReportsToApp" {
            n504 = Unbundle By Name(w1272) -> ("ImpairReportArray"=w1270:T4)
            n505 = Unbundle By Name(w1271) -> ("AppModuleID"=w1269:i32)
            n506 = call "WriteAppInputDataRequest.vi"("InputData"=w1270, "ModuleID"=w1269) -> ("error out"=w1264:errorcluster)  [unwired: 9 in]
            n507 = call <userlib>:"AddError.vi"("Severity"="Abort" ("String"), "Priority"=u8 3, "ErrorArray"=w1263, "error in (no error)"=w1264) -> ("ErrorArray"=w1265:errorcluster[], "error out"=w1266:errorcluster)  [unwired: 6 in]
            n508 = call <vilib>:"Clear Errors.vi"("error in (no error)"=w1266) -> ()  [unwired: 5 in, 2 out]
          }
          frame "TransferFlagsToOutputToFile" {
            n509 = Unbundle By Name(w1281) -> ("OutputToFileModuleID"=w1280:i32)
            n510 = Unbundle By Name(w1282) -> ("FlagImpArray"=w1273:T9)
            n511 = call "WriteFlagImpairArrayRequest.vi"("u32FlagImpairArray"=w1273, "ModuleID"=w1280) -> ("error out"=w1275:errorcluster)  [unwired: 9 in]
            n512 = call <userlib>:"AddError.vi"("Severity"="Abort" ("String"), "Priority"=u8 3, "ErrorArray"=w1274, "error in (no error)"=w1275) -> ("ErrorArray"=w1276:errorcluster[], "error out"=w1277:errorcluster)  [unwired: 6 in]
            n513 = call <vilib>:"Clear Errors.vi"("error in (no error)"=w1277) -> ()  [unwired: 5 in, 2 out]
          }
          frame "TransferPktDlyToOutputToFile" {
            n514 = Unbundle By Name(w1291) -> ("OutputToFileModuleID"=w1290:i32)
            n515 = Unbundle By Name(w1292) -> ("NetworkTime"=w1283:T7)
            n516 = call "WriteNetTimeArrayRequest.vi"("NetTimeArray"=w1283, "ModuleID"=w1290) -> ("error out"=w1285:errorcluster)  [unwired: 9 in]
            n517 = call <userlib>:"AddError.vi"("Severity"="Abort" ("String"), "Priority"=u8 3, "ErrorArray"=w1284, "error in (no error)"=w1285) -> ("ErrorArray"=w1286:errorcluster[], "error out"=w1287:errorcluster)  [unwired: 6 in]
            n518 = call <vilib>:"Clear Errors.vi"("error in (no error)"=w1287) -> ()  [unwired: 5 in, 2 out]
          }
          frame "TransferPtkLossToOutputToFile" {
            n519 = Unbundle By Name(w1301) -> ("OutputToFileModuleID"=w1300:i32)
            n520 = Unbundle By Name(w1302) -> ("PktLoss"=w1293:T8)
            n521 = call "WritePktLossArrayRequest.vi"("PktLossArray"=w1293, "ModuleID"=w1300) -> ("error out"=w1295:errorcluster)  [unwired: 9 in]
            n522 = call <userlib>:"AddError.vi"("Severity"="Abort" ("String"), "Priority"=u8 3, "ErrorArray"=w1294, "error in (no error)"=w1295) -> ("ErrorArray"=w1296:errorcluster[], "error out"=w1297:errorcluster)  [unwired: 6 in]
            n523 = call <vilib>:"Clear Errors.vi"("error in (no error)"=w1297) -> ()  [unwired: 5 in, 2 out]
          }
          frame "OutputErrorsToFile" {
            # "File Name:  Current Timestamp_Bus#_PMUImpairment"
            n524 = Unbundle By Name(w1317) -> ("OutputToFileModuleID"=w1316:i32)
            n525 = Get Date/Time In Seconds() -> (seconds since 1Jan1904=w1309:timestamp)
            n526 = Unbundle By Name(w1318) -> ("BusNumber"=w1305:u8)
            n527 = Format Date/Time String(time format string (%c)="%Y%m%d%H%M%S", seconds (now)=w1309) -> (date/time string=w1306:string)  [unwired: 1 in]
            n528 = Format Into String(format string="%s_Bus%d_PMUImpairment", w1306, w1305) -> (resulting string=w1304:string, error out=w1303:errorcluster)  [unwired: 2 in]
            n529 = call "OutputErrorFileRequest.vi"("error in (no error)"=w1303, "Filename"=w1304, "ModuleID"=w1316) -> ("error out"=w1311:errorcluster)  [unwired: 8 in]
            n530 = call <userlib>:"AddError.vi"("Severity"="Abort" ("String"), "Priority"=u8 3, "ErrorArray"=w1310, "error in (no error)"=w1311) -> ("ErrorArray"=w1312:errorcluster[], "error out"=w1313:errorcluster)  [unwired: 6 in]
            n531 = call <vilib>:"Clear Errors.vi"("error in (no error)"=w1313) -> ()  [unwired: 5 in, 2 out]
          }
          frame "OutputImpairedFileRequest" {
            n532 = Unbundle By Name(w1326) -> ("OutputToFileModuleID"=w1325:i32)
            n533 = call "OutputImpairFileRequest.vi"("ModuleID"=w1325) -> ("error out"=w1320:errorcluster)  [unwired: 10 in]
            n534 = call <userlib>:"AddError.vi"("Severity"="Abort" ("String"), "Priority"=u8 3, "ErrorArray"=w1319, "error in (no error)"=w1320) -> ("ErrorArray"=w1321:errorcluster[], "error out"=w1322:errorcluster)  [unwired: 6 in]
            n535 = call <vilib>:"Clear Errors.vi"("error in (no error)"=w1322) -> ()  [unwired: 5 in, 2 out]
          }
          frame "TransferEvtSignalToPmuImpair" {
            n536 = Unbundle By Name(w1336) -> ("PmuImpairModuleID"=w1335:i32)
            n537 = Unbundle By Name(w1337) -> ("EventSignalArray"=w1328:T6)
            n538 = call "WriteEvtSignalRequest.vi"("EvtSignalArray"=w1328, "ModuleID"=w1335) -> ("error out"=w1330:errorcluster)  [unwired: 9 in]
            n539 = call <userlib>:"AddError.vi"("Severity"="Abort" ("String"), "Priority"=u8 3, "ErrorArray"=w1329, "error in (no error)"=w1330) -> ("ErrorArray"=w1331:errorcluster[], "error out"=w1332:errorcluster)  [unwired: 6 in]
            n540 = call <vilib>:"Clear Errors.vi"("error in (no error)"=w1332) -> ()  [unwired: 5 in, 2 out]
          }
          frame "WriteNetImpairParams" {
            # "Write the event parameters to the event module"
            n541 = Unbundle By Name(w1353) -> ("NetworkImpairModuleID"=w1349:i32)
            n542 = Variant To Data(type=T1 {"BusNumber"=0, "EvtPluginINIFilePath"=path "", "EvtParams"=[], "EvtConfig"={"UTC Time 0"=timestamp(0 s since 1904-01-01), "Nominal Frequency"=60, "Reporting Rate"=60, "Fsamp"=960, "PosSeq"=FALSE}, "Start Time"=0.0, "End Time"=0.0, "PmuImpairPluginINIFilePath"=path "", "PmuImpairParams "=[["960"], ["8.19"], ["164"]], "PmuImpairConfig"={"FilterType"="", "bPosSeq"=TRUE}, "NetImpPluginINIFilePath"=path "", "NetImpParams"=[], "FlagImpPluginINIFilePath"=path "", "FlagImpParams"=[], "EvtReportArray"=[], "EventSignalArray"=[], "ImpairReportArray"=[], "NetworkTime"=[], "PktLoss"=[], "FlagImpArray"=[], "OutputToFilePluginINIFilePath"=path "", "Output File Path"=path "", "clConfigOptions"={"TIME_BASE"=1000000, "STN"="Bus_1", "IDCODE"=0, "rdoPolRect"=enum."Rectangular", "rdoFloatInt"=enum."Float", "PHUNIT"=1000000, "rdoFreqDfreq"=enum."Float", "CHNAM"=["VA", "VB", "VC", "V+", "IA", "IB", "IC", "I+"], "chkCfg2Prefix"=TRUE}, "AppPluginINIFilePath"=path "", "AppConfig"=variant, "AppOutput"=variant} ("clBusData"), Variant=w1351) -> (data=w1350:T1, error out=w1341:errorcluster)  [unwired: 1 in]
            n543 = Unbundle By Name(w1350) -> ("NetImpParams"=w1338:string[][])
            n544 = call "2DstrTableTodblArray.vi"("strTable"=w1338) -> ("dbl2DArray"=w1342:dbl[][])  [unwired: 10 in]
            n545 = call "WriteNetImpParamsRequest.vi"("error in (no error)"=w1341, "dblNetImpParams"=w1342, "ModuleID"=w1349) -> ("error out"=w1344:errorcluster)  [unwired: 8 in]
            n546 = in-place {
              in-place-border: w1338 -> [w1354]
              n547 = in-place-cluster #20(w1340) -> ()  [unwired: 1 out]
              n548 = in-place-cluster #20("NetImpParams"=w1354) -> (w1339:T1)
            }
            n549 = call <userlib>:"AddError.vi"("Severity"="Abort" ("String"), "Priority"=u8 3, "ErrorArray"=w1343, "error in (no error)"=w1344) -> ("ErrorArray"=w1345:errorcluster[], "error out"=w1346:errorcluster)  [unwired: 6 in]
            n550 = call <vilib>:"Clear Errors.vi"("error in (no error)"=w1346) -> ()  [unwired: 5 in, 2 out]
          }
          frame "ReadNetImpairParams" {
            n551 = Unbundle By Name(w1369) -> ("NetworkImpairModuleID"=w1356:i32)
            n552 = call "ObtainBroadcastForRegistration.vi"() -> ("error out"=w1360:errorcluster, "NetImpBroadcast"=w1370:T18)  [unwired: 10 in]
            n553 = register-events(error in=w1360, w1370) -> (reference out=w1357:refnum<event-registration>, error out=w1359:errorcluster)  [unwired: 1 in]
            n554 = call "ReadNetImpParamsRequest.vi"("error in (no error)"=w1359, "ModuleID"=w1356) -> ("error out"=w1358:errorcluster)  [unwired: 9 in]
            n555 = case shown="No Error" w1358 {
              selector: w1358 -> [w1375 w1383]
              tunnel: [w1378 w1382] -> w1362
              tunnel: [w1375 w1383] -> w1361
              tunnel: w1363 -> [w1374 w1382]
              tunnel: w1356 -> [w1373 _]
              tunnel: w1355 -> [w1372 _]
              tunnel: w1357 -> [w1371 _]
              frame No Error {
                n556 = Bundle By Name(cluster=T12 {"ModuleType"=enum."PMU", "ModuleID"=0, "UsrEvtRef"=variant, "ScriptCmd"=""} ("GetBdcstData"), "UsrEvtRef"=w1371, "ModuleID"=w1373, "ModuleType"=ModuleType."Network", "ScriptCmd"=w1372) -> (w1379:T12)
                n557 = call "Enqueue.vi"("Priority (f)"=TRUE, "ErrorArray"=w1374, "Data"=w1379, "Msg"="GetBroadcast") -> ("ErrorArray"=w1378:errorcluster[])  [unwired: 7 in]
              }
              frame Error {
              }
            }
            n558 = call <userlib>:"AddError.vi"("Severity"="Abort" ("String"), "Priority"=u8 3, "ErrorArray"=w1362, "error in (no error)"=w1361) -> ("ErrorArray"=w1365:errorcluster[], "error out"=w1366:errorcluster)  [unwired: 6 in]
            n559 = call <vilib>:"Clear Errors.vi"("error in (no error)"=w1366) -> ()  [unwired: 5 in, 2 out]
          }
          frame "TransferTimeArrayToNetImpair" {
            n560 = Unbundle By Name(w1396) -> ("NetworkImpairModuleID"=w1390:i32)
            n561 = Unbundle By Name(w1395) -> ("EvtConfig.Reporting Rate"=w1394:u16, "End Time"=w1393:dbl, "Start Time"=w1392:dbl)
            n562 = To Double Precision Float(number=w1394) -> (double precision float=w1398:dbl)
            n563 = Reciprocal(x=w1398) -> (1/x=w1397:dbl)
            n564 = call-poly <vilib>:"Ramp Pattern.vi"("start"=w1392, "end"=w1393, "delta"=w1397) -> ("Ramp Pattern"=w1391:dbl[])  [unwired: 6 in, 2 out]
            n565 = call "WriteTimeArrayRequest.vi"("TimeArray"=w1391, "Module ID"=w1390) -> ("error out"=w1384:errorcluster)  [unwired: 9 in]
            n566 = call <userlib>:"AddError.vi"("Severity"="Abort" ("String"), "Priority"=u8 3, "ErrorArray"=w1385, "error in (no error)"=w1384) -> ("ErrorArray"=w1386:errorcluster[], "error out"=w1387:errorcluster)  [unwired: 6 in]
            n567 = call <vilib>:"Clear Errors.vi"("error in (no error)"=w1387) -> ()  [unwired: 5 in, 2 out]
          }
          frame "WriteFlagImpairParams" {
            # "Write the event parameters to the event module"
            n568 = Variant To Data(type=T1 {"BusNumber"=0, "EvtPluginINIFilePath"=path "", "EvtParams"=[], "EvtConfig"={"UTC Time 0"=timestamp(0 s since 1904-01-01), "Nominal Frequency"=60, "Reporting Rate"=60, "Fsamp"=960, "PosSeq"=FALSE}, "Start Time"=0.0, "End Time"=0.0, "PmuImpairPluginINIFilePath"=path "", "PmuImpairParams "=[["960"], ["8.19"], ["164"]], "PmuImpairConfig"={"FilterType"="", "bPosSeq"=TRUE}, "NetImpPluginINIFilePath"=path "", "NetImpParams"=[], "FlagImpPluginINIFilePath"=path "", "FlagImpParams"=[], "EvtReportArray"=[], "EventSignalArray"=[], "ImpairReportArray"=[], "NetworkTime"=[], "PktLoss"=[], "FlagImpArray"=[], "OutputToFilePluginINIFilePath"=path "", "Output File Path"=path "", "clConfigOptions"={"TIME_BASE"=1000000, "STN"="Bus_1", "IDCODE"=0, "rdoPolRect"=enum."Rectangular", "rdoFloatInt"=enum."Float", "PHUNIT"=1000000, "rdoFreqDfreq"=enum."Float", "CHNAM"=["VA", "VB", "VC", "V+", "IA", "IB", "IC", "I+"], "chkCfg2Prefix"=TRUE}, "AppPluginINIFilePath"=path "", "AppConfig"=variant, "AppOutput"=variant} ("clBusData"), Variant=w1412) -> (data=w1411:T1, error out=w1402:errorcluster)  [unwired: 1 in]
            n569 = Unbundle By Name(w1414) -> ("FlagImpairModuleID"=w1410:i32)
            n570 = Unbundle By Name(w1411) -> ("FlagImpParams"=w1399:string[][])
            n571 = call "2DstrTableTodblArray.vi"("strTable"=w1399) -> ("dbl2DArray"=w1403:dbl[][])  [unwired: 10 in]
            n572 = call "WriteFlagImpairParamsRequest.vi"("error in (no error)"=w1402, "dblFlagImpairParams"=w1403, "ModuleID"=w1410) -> ("error out"=w1405:errorcluster)  [unwired: 8 in]
            n573 = in-place {
              in-place-border: w1399 -> [w1415]
              n574 = in-place-cluster #21(w1401) -> ()  [unwired: 1 out]
              n575 = in-place-cluster #21("FlagImpParams"=w1415) -> (w1400:T1)
            }
            n576 = call <userlib>:"AddError.vi"("Severity"="Abort" ("String"), "Priority"=u8 3, "ErrorArray"=w1404, "error in (no error)"=w1405) -> ("ErrorArray"=w1406:errorcluster[], "error out"=w1407:errorcluster)  [unwired: 6 in]
            n577 = call <vilib>:"Clear Errors.vi"("error in (no error)"=w1407) -> ()  [unwired: 5 in, 2 out]
          }
          frame "ReadFlagImpairParams" {
            n578 = Unbundle By Name(w1430) -> ("FlagImpairModuleID"=w1417:i32)
            n579 = call "ObtainBroadcastForRegistration.vi"() -> ("error out"=w1422:errorcluster, "FlagImpairBroadcasts"=w1431:T19)  [unwired: 10 in]
            n580 = register-events(error in=w1422, w1431) -> (reference out=w1419:refnum<event-registration>, error out=w1421:errorcluster)  [unwired: 1 in]
            n581 = call "ReadFlagImpairParamsRequest.vi"("error in (no error)"=w1421, "ModuleID"=w1417) -> ("error out"=w1420:errorcluster)  [unwired: 9 in]
            n582 = case shown="No Error" w1420 {
              selector: w1420 -> [w1436 w1444]
              tunnel: [w1439 w1443] -> w1423
              tunnel: [w1436 w1444] -> w1418
              tunnel: w1424 -> [w1435 w1443]
              tunnel: w1417 -> [w1434 _]
              tunnel: w1416 -> [w1433 _]
              tunnel: w1419 -> [w1432 _]
              frame No Error {
                n583 = Bundle By Name(cluster=T12 {"ModuleType"=enum."PMU", "ModuleID"=0, "UsrEvtRef"=variant, "ScriptCmd"=""} ("GetBdcstData"), "UsrEvtRef"=w1432, "ModuleID"=w1434, "ModuleType"=ModuleType."Flag", "ScriptCmd"=w1433) -> (w1440:T12)
                n584 = call "Enqueue.vi"("Priority (f)"=TRUE, "ErrorArray"=w1435, "Data"=w1440, "Msg"="GetBroadcast") -> ("ErrorArray"=w1439:errorcluster[])  [unwired: 7 in]
              }
              frame Error {
              }
            }
            n585 = call <userlib>:"AddError.vi"("Severity"="Abort" ("String"), "Priority"=u8 3, "ErrorArray"=w1423, "error in (no error)"=w1418) -> ("ErrorArray"=w1426:errorcluster[], "error out"=w1427:errorcluster)  [unwired: 6 in]
            n586 = call <vilib>:"Clear Errors.vi"("error in (no error)"=w1427) -> ()  [unwired: 5 in, 2 out]
          }
          frame "WritePmuConfig" {
            n587 = property class="Bus.lvclass"(reference=w1454) -> ("Accessors:PmuImpairModuleID"=w1453:i32)  [unwired: 1 in, 2 out]
            n588 = Variant To Data(type=T1 {"BusNumber"=0, "EvtPluginINIFilePath"=path "", "EvtParams"=[], "EvtConfig"={"UTC Time 0"=timestamp(0 s since 1904-01-01), "Nominal Frequency"=60, "Reporting Rate"=60, "Fsamp"=960, "PosSeq"=FALSE}, "Start Time"=0.0, "End Time"=0.0, "PmuImpairPluginINIFilePath"=path "", "PmuImpairParams "=[["960"], ["8.19"], ["164"]], "PmuImpairConfig"={"FilterType"="", "bPosSeq"=TRUE}, "NetImpPluginINIFilePath"=path "", "NetImpParams"=[], "FlagImpPluginINIFilePath"=path "", "FlagImpParams"=[], "EvtReportArray"=[], "EventSignalArray"=[], "ImpairReportArray"=[], "NetworkTime"=[], "PktLoss"=[], "FlagImpArray"=[], "OutputToFilePluginINIFilePath"=path "", "Output File Path"=path "", "clConfigOptions"={"TIME_BASE"=1000000, "STN"="Bus_1", "IDCODE"=0, "rdoPolRect"=enum."Rectangular", "rdoFloatInt"=enum."Float", "PHUNIT"=1000000, "rdoFreqDfreq"=enum."Float", "CHNAM"=["VA", "VB", "VC", "V+", "IA", "IB", "IC", "I+"], "chkCfg2Prefix"=TRUE}, "AppPluginINIFilePath"=path "", "AppConfig"=variant, "AppOutput"=variant} ("clBusData"), Variant=w1459) -> (data=w1456:T1, error out=w1452:errorcluster)  [unwired: 1 in]
            n589 = Unbundle By Name(w1456) -> ("clConfigOptions"=w1455:T10)
            n590 = in-place {
              in-place-border: w1455 -> [w1460]
              n591 = in-place-cluster #22(w1457) -> ()  [unwired: 1 out]
              n592 = in-place-cluster #22("clConfigOptions"=w1460) -> (w1445:T1)
            }
            n593 = call "WritePMUConfigRequest.vi"("error in (no error)"=w1452, "PmuConfig"=w1455, "ModuleID"=w1453) -> ("error out"=w1447:errorcluster)  [unwired: 8 in]
            n594 = call <userlib>:"AddError.vi"("Severity"="Abort" ("String"), "Priority"=u8 3, "ErrorArray"=w1446, "error in (no error)"=w1447) -> ("ErrorArray"=w1448:errorcluster[], "error out"=w1449:errorcluster)  [unwired: 6 in]
            n595 = call <vilib>:"Clear Errors.vi"("error in (no error)"=w1449) -> ()  [unwired: 5 in, 2 out]
          }
          frame "TransferEvtConfigToApp" {
            n596 = Unbundle By Name(w1469) -> ("AppModuleID"=w1467:i32)
            n597 = Unbundle By Name(w1468) -> ("EvtConfig"=w1461:T2)
            n598 = call "WriteEvtConfigRequest.vi"("InputData"=w1461, "ModuleID"=w1467) -> ("error out"=w1462:errorcluster)  [unwired: 9 in]
            n599 = call <userlib>:"AddError.vi"("Severity"="Abort", "Priority"=u8 3, "ErrorArray"=w1463, "error in (no error)"=w1462) -> ("ErrorArray"=w1466:errorcluster[])  [unwired: 6 in, 1 out]
          }
          frame "Initialize" {
            # "Error Check, the queue should be empty when this is called"
            # "The state called upon entry"
            n600 = call "ObtainSMQueue.vi"("ErrorArray"=w1481) -> ("ErrorArray"=w1474:errorcluster[], "QueRef"=w1480:T23)  [unwired: 9 in]
            n601 = Get Queue Status(queue=w1480) -> (error out=w1473:errorcluster, # elements in queue=w1478:i32)  [unwired: 2 in, 6 out]
            n602 = Equal To 0?(x=w1478) -> (x = 0?=w1472:bool)
            n603 = call <userlib>:"AddError.vi"("Severity"="Abort" ("String"), "Priority"=u8 3, "ErrorArray"=w1474, "error in (no error)"=w1473) -> ("ErrorArray"=w1471:errorcluster[], "error out"=w1475:errorcluster)  [unwired: 6 in]
            n604 = call <vilib>:"Clear Errors.vi"("error in (no error)"=w1475) -> ()  [unwired: 5 in, 2 out]
            n605 = case shown="True" w1472 {
              tunnel: [w1485 w1501] -> w1482
              tunnel: w1479 -> [_ w1500]
              tunnel: w1471 -> [w1483 w1496]
              frame False {
                # "Initialize was called with script elements still in the queue"
                n606 = xnode "Error Ring"() -> ("error out"=w1484:errorcluster)
                n607 = call <userlib>:"AddError.vi"("Severity"="Abort" ("String"), "Priority"=u8 3, "ErrorArray"=w1483, "error in (no error)"=w1484) -> ("ErrorArray"=w1485:errorcluster[], "error out"=w1486:errorcluster)  [unwired: 6 in]
                n608 = call <vilib>:"Clear Errors.vi"("error in (no error)"=w1486) -> ()  [unwired: 5 in, 2 out]
              }
              frame True {
                w1502 = string[] []
                # "Enqueue the script"
                n609 = Variant To Data(type=w1502, Variant=w1500) -> (data=w1503:string[], error out=w1494:errorcluster)  [unwired: 1 in]
                n610 = call <userlib>:"AddError.vi"("Severity"="Abort" ("String"), "Priority"=u8 3, "ErrorArray"=w1496, "error in (no error)"=w1494) -> ("ErrorArray"=w1495:errorcluster[], "error out"=w1497:errorcluster)  [unwired: 6 in]
                n611 = call <vilib>:"Clear Errors.vi"("error in (no error)"=w1497) -> ()  [unwired: 5 in, 2 out]
                n612 = for {
                  tunnel: w1503 -> [w1515] mode=indexing
                  tunnel: w1502 -> [w1514]
                  tunnel: w1495 -> [w1505]
                  tunnel: [w1504] -> w1501 mode=concatenating
                  n613 = Spreadsheet String To Array(delimiter (Tab)="," ("format string"), format string="%s", spreadsheet string=w1515, array type (2D Dbl)=w1514) -> (array=w1511:string[])
                  n614 = Split 1D Array(array=w1511, index=1) -> (first subarray=w1507:string[], second subarray=w1509:string[])
                  n615 = To Variant(anything=w1509) -> (Variant=w1508:variant)
                  n616 = Index Array(array=w1507) -> (element=w1506:string)  [unwired: 1 in]
                  n617 = call "Enqueue.vi"("ErrorArray"=w1505, "Data"=w1508, "Msg"=w1506) -> ("ErrorArray"=w1504:errorcluster[])  [unwired: 8 in]
                }
              }
            }
          }
          frame "Abort" {
            # "Note, if any cleanup is needed before stop, do it here.  \n\nOne idea would be to use the queue data to tell abort what needs to be done."
            # "Comes here if the SM is aborted by the user or a script"
            n618 = call "Enqueue.vi"("Priority (f)"=TRUE, "ErrorArray"=w1517, "Msg"="Stop") -> ("ErrorArray"=w1520:errorcluster[])  [unwired: 8 in]
          }
          frame "Stop" {
            # "Destroy the Queue"
            # "Flush the Queue"
            n619 = call "ObtainSMQueue.vi"("ErrorArray"=w1532) -> ("ErrorArray"=w1525:errorcluster[], "QueRef"=w1531:T23)  [unwired: 9 in]
            n620 = Flush Queue(queue=w1531) -> (queue out=w1530:T23, error out=w1529:errorcluster)  [unwired: 1 in, 1 out]
            n621 = Release Queue(queue=w1530, error in (no error)=w1529) -> (error out=w1523:errorcluster)  [unwired: 1 in, 2 out]
            n622 = call <userlib>:"AddError.vi"("Severity"="Abort" ("String"), "Priority"=u8 3, "ErrorArray"=w1525, "error in (no error)"=w1523) -> ("ErrorArray"=w1524:errorcluster[], "error out"=w1526:errorcluster)  [unwired: 6 in]
            n623 = To Variant(anything=w1521) -> (Variant=w1522:variant)
            n624 = call <vilib>:"Clear Errors.vi"("error in (no error)"=w1526) -> ()  [unwired: 5 in, 2 out]
          }
          frame Default {
            n625 = xnode "Error Ring"("parameter 0"=w1539) -> ("error out"=w1540:errorcluster)
            n626 = call <userlib>:"AddError.vi"("Severity"="Abort" ("String"), "Priority"=u8 3, "ErrorArray"=w1538, "error in (no error)"=w1540) -> ("ErrorArray"=w1537:errorcluster[], "error out"=w1536:errorcluster)  [unwired: 6 in]
            n627 = call <vilib>:"Clear Errors.vi"("error in (no error)"=w1536) -> ()  [unwired: 5 in, 2 out]
          }
          frame "Error" {
            n628 = Variant To Data(type=errorcluster[] [], Variant=w1558) -> (data=w1556:errorcluster[])  [unwired: 1 in, 1 out]
            n629 = call <userlib>:"ParseErrors.vi"("ErrorArray"=w1556) -> ("ErrorArray"=w1555:errorcluster[])  [unwired: 8 in, 2 out]
            n630 = for {
              tunnel: w1555 -> [w1568] mode=indexing
              tunnel: [w1560] -> w1554 mode=concatenating
              tunnel: w1551 -> [w1559]
              n631 = Unbundle By Name(w1568) -> ("source"=w1562:string)
              n632 = call <userlib>:"GeneralHandler.vi"("error in (no error)"=w1568) -> ("Severity"=w1563:string, "Stop"=w1565:bool, "Abort"=w1566:bool, "Continue"=w1567:bool)  [unwired: 7 in]
              n633 = Build Array(w1567, w1566, w1565) -> (w1564:bool[])
              n634 = Boolean Array To Number(Boolean array=w1564) -> (number=w1561:u32)
              n635 = case shown="4" w1561 {
                tunnel: w1563 -> [_ w1570 w1577 w1583]
                tunnel: [_ _ w1576 w1582] -> w1560
                tunnel: w1562 -> [_ w1569 _ _]
                tunnel: w1559 -> [_ _ _ w1581]
                frame 0, Default {
                  # "No dialogue button pressed"
                }
                frame 1 {
                  # "Continue button pressed"
                  n636 = case shown="Default" w1570 {
                    tunnel: w1569 -> [_ w1571]
                    frame Default {
                      # "Let the State machine continue."
                    }
                    frame "Log" {
                      # "TODO : this is unfinished code"
                      # "Write to log file?"
                      n637 = Get Date/Time String(want seconds? (F)=TRUE) -> (time string=w1574:string)  [unwired: 2 in, 1 out]
                      n638 = call <vilib>:"Space Constant.vi"() -> ("String"=w1573:string)
                      n639 = Concatenate Strings(w1574, w1573, w1571, "\r\n") -> ()  [unwired: 1 out]
                    }
                  }
                }
                frame 2 {
                  # "Abort Button Pressed"
                  n640 = case shown="Default" w1577 {
                    tunnel: [w1578] -> w1576
                    frame Default {
                      # "Note:  we may be able to use the queue data to tell the system if anything needs cleanup"
                      # "go to the abort state"
                      n641 = call "Enqueue.vi"("Priority (f)"=TRUE, "Msg"="Abort") -> ("ErrorArray"=w1578:errorcluster[])  [unwired: 9 in]
                    }
                  }
                }
                frame 4 {
                  # "Stop Button Pressed"
                  n642 = case shown="Default" w1583 {
                    tunnel: [w1589] -> w1582
                    tunnel: w1581 -> [w1586]
                    frame Default {
                      # "Immediatly stop the state machine and send a stop request up to the framework"
                      n643 = Unbundle By Name(w1586) -> ("BusNumber"=w1585:u8)
                      n644 = call "Enqueue.vi"("Priority (f)"=TRUE, "Msg"="Stop") -> ("ErrorArray"=w1588:errorcluster[])  [unwired: 9 in]
                      n645 = call "StopRequest.vi"("ErrorArray In"=w1588, "BusIndex"=w1585) -> ("ErrorArray Out"=w1589:errorcluster[])  [unwired: 9 in]
                    }
                  }
                }
              }
            }
            n646 = call <userlib>:"ClearErrors.vi"() -> ("ErrorArray"=w1553:errorcluster[])  [unwired: 11 in]
            n647 = Build Array (concatenate)(w1554, w1553) -> (w1552:errorcluster[])
          }
          frame "GetPmuImpairReports - unused" {
            # "This has been replaced by the bus Controller.  Gets the PMU Impaired reports from one bus"
            n648 = Unbundle By Name(w1604) -> ("PmuImpairModuleID"=w1591:i32)
            n649 = call "ObtainBroadcastForRegistration.vi"() -> ("error out"=w1598:errorcluster, "ImpairBroadcast"=w1603:T17)  [unwired: 10 in]
            n650 = register-events(error in=w1598, w1603) -> (reference out=w1592:refnum<event-registration>, error out=w1597:errorcluster)  [unwired: 1 in]
            n651 = call "GetImpairReportsRequest.vi"("error in (no error)"=w1597, "ModuleID"=w1591) -> ("error out"=w1593:errorcluster)  [unwired: 9 in]
            n652 = case shown="No Error" w1593 {
              selector: w1593 -> [w1609 w1617]
              tunnel: [w1612 w1616] -> w1594
              tunnel: [w1609 w1617] -> _
              tunnel: w1595 -> [w1608 w1616]
              tunnel: w1591 -> [w1607 _]
              tunnel: w1590 -> [w1606 _]
              tunnel: w1592 -> [w1605 _]
              frame No Error {
                n653 = Bundle By Name(cluster=T12 {"ModuleType"=enum."PMU", "ModuleID"=0, "UsrEvtRef"=variant, "ScriptCmd"=""} ("GetBdcstData"), "UsrEvtRef"=w1605, "ModuleID"=w1607, "ModuleType"=ModuleType."PMU", "ScriptCmd"=w1606) -> (w1613:T12)
                n654 = call "Enqueue.vi"("Priority (f)"=TRUE, "ErrorArray"=w1608, "Data"=w1613, "Msg"="GetBroadcast") -> ("ErrorArray"=w1612:errorcluster[])  [unwired: 7 in]
              }
              frame Error {
              }
            }
            n655 = call <userlib>:"AddError.vi"("Severity"="Abort" ("String"), "Priority"=u8 3, "ErrorArray"=w1594) -> ("ErrorArray"=w1599:errorcluster[], "error out"=w1600:errorcluster)  [unwired: 7 in]
            n656 = call <vilib>:"Clear Errors.vi"("error in (no error)"=w1600) -> ()  [unwired: 5 in, 2 out]
          }
          frame "GetNetImpairTime - unused" {
            n657 = Unbundle By Name(w1633) -> ("NetworkImpairModuleID"=w1620:i32)
            n658 = call "ObtainBroadcastForRegistration.vi"() -> ("error out"=w1626:errorcluster, "NetImpBroadcast"=w1632:T18)  [unwired: 10 in]
            n659 = register-events(error in=w1626, w1632) -> (reference out=w1621:refnum<event-registration>, error out=w1625:errorcluster)  [unwired: 1 in]
            n660 = call "GetNetTimeRequest.vi"("error in (no error)"=w1625, "ModuleID"=w1620) -> ("error out"=w1622:errorcluster)  [unwired: 9 in]
            n661 = case shown="No Error" w1622 {
              selector: w1622 -> [w1638 w1646]
              tunnel: [w1641 w1645] -> w1623
              tunnel: [w1638 w1646] -> w1618
              tunnel: w1624 -> [w1637 w1645]
              tunnel: w1620 -> [w1636 _]
              tunnel: w1619 -> [w1635 _]
              tunnel: w1621 -> [w1634 _]
              frame No Error {
                n662 = Bundle By Name(cluster=T12 {"ModuleType"=enum."PMU", "ModuleID"=0, "UsrEvtRef"=variant, "ScriptCmd"=""} ("GetBdcstData"), "UsrEvtRef"=w1634, "ModuleID"=w1636, "ModuleType"=ModuleType."Network", "ScriptCmd"=w1635) -> (w1642:T12)
                n663 = call "Enqueue.vi"("Priority (f)"=TRUE, "ErrorArray"=w1637, "Data"=w1642, "Msg"="GetBroadcast") -> ("ErrorArray"=w1641:errorcluster[])  [unwired: 7 in]
              }
              frame Error {
              }
            }
            n664 = call <userlib>:"AddError.vi"("Severity"="Abort" ("String"), "Priority"=u8 3, "ErrorArray"=w1623, "error in (no error)"=w1618) -> ("ErrorArray"=w1628:errorcluster[], "error out"=w1629:errorcluster)  [unwired: 6 in]
            n665 = call <vilib>:"Clear Errors.vi"("error in (no error)"=w1629) -> ()  [unwired: 5 in, 2 out]
          }
          frame "TransferTimeArrayToFlagImpair-unused" {
            n666 = Unbundle By Name(w1658) -> ("EvtConfig.Reporting Rate"=w1657:u16, "End Time"=w1656:dbl, "Start Time"=w1655:dbl)
            n667 = Unbundle By Name(w1659) -> ("FlagImpairModuleID"=w1653:i32)
            n668 = To Double Precision Float(number=w1657) -> (double precision float=w1661:dbl)
            n669 = Reciprocal(x=w1661) -> (1/x=w1660:dbl)
            n670 = call-poly <vilib>:"Ramp Pattern.vi"("start"=w1655, "end"=w1656, "delta"=w1660) -> ("Ramp Pattern"=w1654:dbl[])  [unwired: 6 in, 2 out]
            n671 = call "WriteTimeArrayRequest.vi"("dblTimeArray"=w1654, "ModuleID"=w1653) -> ("error out"=w1647:errorcluster)  [unwired: 9 in]
            n672 = call <userlib>:"AddError.vi"("Severity"="Abort" ("String"), "Priority"=u8 3, "ErrorArray"=w1648, "error in (no error)"=w1647) -> ("ErrorArray"=w1649:errorcluster[], "error out"=w1650:errorcluster)  [unwired: 6 in]
            n673 = call <vilib>:"Clear Errors.vi"("error in (no error)"=w1650) -> ()  [unwired: 5 in, 2 out]
          }
          frame "GetFlagImpairArray - unused" {
            n674 = Unbundle By Name(w1677) -> ("FlagImpairModuleID"=w1663:i32)
            n675 = call "ObtainBroadcastForRegistration.vi"() -> ("error out"=w1670:errorcluster, "FlagImpairBroadcasts"=w1676:T19)  [unwired: 10 in]
            n676 = register-events(error in=w1670, w1676) -> (reference out=w1664:refnum<event-registration>, error out=w1669:errorcluster)  [unwired: 1 in]
            n677 = call "GetFlagImpairmentArrayRequest.vi"("error in (no error)"=w1669, "ModuleID"=w1663) -> ("error out"=w1665:errorcluster)  [unwired: 9 in]
            n678 = case shown="No Error" w1665 {
              selector: w1665 -> [w1682 w1690]
              tunnel: [w1685 w1689] -> w1666
              tunnel: [w1682 w1690] -> w1667
              tunnel: w1668 -> [w1681 w1689]
              tunnel: w1663 -> [w1680 _]
              tunnel: w1662 -> [w1679 _]
              tunnel: w1664 -> [w1678 _]
              frame No Error {
                n679 = Bundle By Name(cluster=T12 {"ModuleType"=enum."PMU", "ModuleID"=0, "UsrEvtRef"=variant, "ScriptCmd"=""} ("GetBdcstData"), "UsrEvtRef"=w1678, "ModuleID"=w1680, "ModuleType"=ModuleType."Flag", "ScriptCmd"=w1679) -> (w1686:T12)
                n680 = call "Enqueue.vi"("Priority (f)"=TRUE, "ErrorArray"=w1681, "Data"=w1686, "Msg"="GetBroadcast") -> ("ErrorArray"=w1685:errorcluster[])  [unwired: 7 in]
              }
              frame Error {
              }
            }
            n681 = call <userlib>:"AddError.vi"("Severity"="Abort" ("String"), "Priority"=u8 3, "ErrorArray"=w1666, "error in (no error)"=w1667) -> ("ErrorArray"=w1672:errorcluster[], "error out"=w1673:errorcluster)  [unwired: 6 in]
            n682 = call <vilib>:"Clear Errors.vi"("error in (no error)"=w1673) -> ()  [unwired: 5 in, 2 out]
          }
          frame "AggregatePmuImpairRpts - unused" {
            # "This should be replaced in the script by the aggregate command Gets the PMU Impaired reports from all buses and indexes them together based on time stamp"
            n683 = call "GetSetFrameworkData.vi"() -> ("clFrameworkData Out"=w1709:T22)  [unwired: 11 in]
            n684 = call "ObtainBroadcastForRegistration.vi"() -> ("error out"=w1697:errorcluster, "ImpairBroadcast"=w1699:T17)  [unwired: 10 in]
            n685 = Unbundle By Name(w1709) -> ("BusClassInstances"=w1708:refnum<class "Bus.lvclass">[])
            n686 = register-events(w1699) -> (reference out=w1698:refnum<event-registration>)  [unwired: 2 in, 1 out]
            n687 = for {
              tunnel: w1710 -> [w1723]
              tunnel: w1708 -> [w1722] mode=indexing
              shift-right: [w1719] -> w1693
              shift-left: w1707 -> [w1718]
              shift-right: [w1716] -> w1703
              shift-left: T4 [{"Timestamp"=0.0, "Synx"=[], "Freq"=0.0, "ROCOF"=0.0, "ID"=0}] ("Aggregated Out") -> [w1715]
              tunnel: w1698 -> [w1714]
              tunnel: w1697 -> [w1713]
              tunnel: [w1711] -> w1696
              n688 = Unbundle By Name(w1722) -> ("PmuImpairModuleID"=w1725:i32)
              n689 = call "GetImpairReportsRequest.vi"("error in (no error)"=w1713, "ModuleID"=w1725) -> ("error out"=w1726:errorcluster)  [unwired: 9 in]
              n690 = event shown="[1] <ImpairBroadcast.ErrorReport>: User Event" {
                selector: w1714 -> [_ _ _]
                dyn-events: [_ _ _] -> w1711
                timeout: 10000 -> [_ _ _]
                tunnel: w1726 -> [w1730 _ w1736]
                tunnel: [w1728 _ _] -> w1717
                tunnel: [w1729 w1732 w1737] -> w1712
                tunnel: w1723 -> [_ _ w1738]
                event User Event {
                  n691 = event-data() -> ("Data"=w1731:variant)  [unwired: 1 in]
                  n692 = Variant To Data(error in=w1730, type=T4 [] ("clEvtReportArray"), Variant=w1731) -> (data=w1728:T4, error out=w1729:errorcluster)
                }
                event User Event {
                  n693 = event-data() -> ("Data"=w1733:variant)  [unwired: 1 in]
                  n694 = Variant To Data(type=T14 {"error"={"status"=FALSE, "code"=0, "source"=""}, "AdditionalInfo"=""} ("Cluster"), Variant=w1733) -> (data=w1734:T14)  [unwired: 1 in, 1 out]
                  n695 = Unbundle By Name(w1734) -> ("error"=w1732:errorcluster)
                }
                event Timeout {
                  n696 = event-data() -> ()  [unwired: 1 in, 1 out]
                  n697 = xnode "Error Ring"("parameter 0"=w1738) -> ("error out"=w1739:errorcluster)
                  n698 = Merge Errors(w1736, w1739) -> (w1737:errorcluster)
                }
              }
              n699 = call "AggregateReports.vi"("Additional In"=w1717, "Aggregated In"=w1715) -> ("Aggregated Out"=w1716:T4)  [unwired: 9 in]
              n700 = call <userlib>:"AddError.vi"("Severity"="Abort" ("String"), "Priority"=u8 3, "ErrorArray"=w1718, "error in (no error)"=w1712) -> ("ErrorArray"=w1719:errorcluster[])  [unwired: 6 in, 1 out]
            }
            n701 = Unregister For Events(event registration refnum=w1696) -> (error out=w1691:errorcluster)  [unwired: 1 in]
            n702 = Array Size(array=w1703) -> (size(s)=w1701:i32)
            n703 = Decrement(x=w1701) -> (x-1=w1700:i32)
            n704 = Delete From Array(array=w1703, index=w1700) -> (array with subset deleted=w1702:T4)  [unwired: 1 in, 1 out]
            n705 = call <userlib>:"AddError.vi"("Severity"="Abort" ("String"), "Priority"=u8 3, "ErrorArray"=w1693, "error in (no error)"=w1691) -> ("ErrorArray"=w1692:errorcluster[])  [unwired: 6 in, 1 out]
            n706 = Bundle By Name(cluster=w1705, "ImpairReportArray"=w1702) -> (w1704:T1)
          }
          frame "GetNetPktLoss - unused" {
            n707 = Unbundle By Name(w1762) -> ("NetworkImpairModuleID"=w1749:i32)
            n708 = call "ObtainBroadcastForRegistration.vi"() -> ("error out"=w1755:errorcluster, "NetImpBroadcast"=w1761:T18)  [unwired: 10 in]
            n709 = register-events(error in=w1755, w1761) -> (reference out=w1750:refnum<event-registration>, error out=w1754:errorcluster)  [unwired: 1 in]
            n710 = call "GetPktLossRequest.vi"("error in (no error)"=w1754, "ModuleID"=w1749) -> ("error out"=w1751:errorcluster)  [unwired: 9 in]
            n711 = case shown="No Error" w1751 {
              selector: w1751 -> [w1767 w1775]
              tunnel: [w1770 w1774] -> w1752
              tunnel: [w1767 w1775] -> w1748
              tunnel: w1753 -> [w1766 w1774]
              tunnel: w1749 -> [w1765 _]
              tunnel: w1747 -> [w1764 _]
              tunnel: w1750 -> [w1763 _]
              frame No Error {
                n712 = Bundle By Name(cluster=T12 {"ModuleType"=enum."PMU", "ModuleID"=0, "UsrEvtRef"=variant, "ScriptCmd"=""} ("GetBdcstData"), "UsrEvtRef"=w1763, "ModuleID"=w1765, "ModuleType"=ModuleType."Network", "ScriptCmd"=w1764) -> (w1771:T12)
                n713 = call "Enqueue.vi"("Priority (f)"=TRUE, "ErrorArray"=w1766, "Data"=w1771, "Msg"="GetBroadcast") -> ("ErrorArray"=w1770:errorcluster[])  [unwired: 7 in]
              }
              frame Error {
              }
            }
            n714 = call <userlib>:"AddError.vi"("Severity"="Abort" ("String"), "Priority"=u8 3, "ErrorArray"=w1752, "error in (no error)"=w1748) -> ("ErrorArray"=w1757:errorcluster[], "error out"=w1758:errorcluster)  [unwired: 6 in]
            n715 = call <vilib>:"Clear Errors.vi"("error in (no error)"=w1758) -> ()  [unwired: 5 in, 2 out]
          }
        }
        n716 = call "EnqueueError.vi"("ErrorArray"=w36) -> ("ErrorArray"=w37:errorcluster[])  [unwired: 10 in]
      }
    }
  }
  "ErrorArray Out" <- w13
  "Data out" <- w10
  "Bus" <- "Bus"
